vi "Cobra GUI_5.14.vi"(8 "error in":errorcluster) -> (0 "Error Out":errorcluster)   [LabVIEW 2019, in "GUI.lvlib"]
doc: "GUI 21.6.7"
uses:
  GUI.lvlib
  Private Controls/Main Waveform.ctl
  Private Controls/Profile Sequence.ctl
  Private Controls/System Graphs.ctl
  Private Controls/Module Graphs.ctl
  Private Controls/Dial Gauges.ctl
  Private Controls/Gauge Graphs/Compression Ratio.ctl
  Private Controls/Gauge Graphs/Subcooling.ctl
  Private Controls/Gauge Graphs/Superheat.ctl
  Private Controls/Gauge Graphs/Current.ctl
  Private Controls/Module Key Values.ctl
  Private Controls/Event.ctl
  Custom Controls/login.ctl
  Private Controls/Messaging Actions.ctl
  Private Controls/GUI Variables.ctl
  Private Controls/Network Data Down_set back.ctl
  Private Controls/NS New Data.ctl
  <vilib>/NI/STM/TCP/TCP Connection Info.ctl
  <vilib>/NI/STM/SubVIs/MetaDataElement.ctl
  Private Controls/Dataset.ctl
  Private Controls/System Status.ctl
  Private Controls/Module Status.ctl
  Private Controls/M2 Status.ctl
  Private Controls/Config Data.ctl
  <vilib>/Utility/miscctls.llb/LVPositionTypeDef.ctl
  Private Controls/WebDAV states.ctl
  <vilib>/NI/STM/TCP/TCP Read Options.ctl
  46123981-91be-4060-8772-f60ae0a7e702.vi
  <vilib>/Analysis/baseanly.llb/Mean (DBL).vi
  b9938fbe-5ccd-4e62-98e3-88d978d07e59.vi
  795e1a79-78c9-4e5b-9a6d-4827452a9509.vi
  894b418a-eb83-4c03-97c2-0273c02a970a.vi
  81edff22-585a-4beb-bf15-c06a681b6c24.vi
  <vilib>/NI/STM/TCP/Read Meta Data (TCP Ref).vi
  <vilib>/NI/STM/TCP/Get Connection Reference (TCP).vi
  <vilib>/NI/STM/TCP/Read Meta Data (TCP Clst).vi
  <vilib>/NI/STM/TCP/Read Message (TCP).vi
  <vilib>/NI/STM/TCP/Write Message (TCP).vi
  <vilib>/regexp/Match Regular Expression.xnode
  <vilib>/nisyscfg/nisyscfg.lvlib
  <resource>/objmgr/ni.dex.rc
  Private Controls/Save Log State.ctl
  <vilib>/Analysis/NI_AALBase.lvlib
  <vilib>/WebDAVClient/NI_WebDAV.lvlib
  <vilib>/NI/STM/NI STM.lvlib
  <vilib>/addons/_JKI.lib/Serialization/JSON/JKI JSON Serialization.lvlib
panel:
  out "RT Version":string=" May 1st 2021 Cobra GUI v1.0\n\nModule Core.  This is the main VI for a new module. This module is self contained in that it can run on it's own without any other top level VIs. Alternatively you can call this VI from a top level VI and use it as an actor. By default the front panel will open.\n" caption="Cobra GUI Version :"
  in  "Reboot RT":bool
  in  "Shutdown":bool caption="Stop RT"
  in  "M1 Feedback":u8(ring)=1 caption="Enable" items=["Evap Temp", "Case Temp", "Intec Temp", "TSD  Temp", "Autotune", "Extra"]
  in  "M2 Feedback":u8(ring)=1 caption="Enable" items=["Evap Temp", "Case Temp", "Intec Temp", "TSD  Temp", "Autotune", "Extra"]
  out "M2 Data":T1={"Set Temp"=20.0, "Read Temp"=0.0, "Package"="", "Force"=0.0, "Feedback"=1} caption="M2 Status" {"Feedback" items=["Evap Temp", "Case Temp", "Intec Temp", "TSD  Temp", "Autotune", "Extra"]; "Force" format="%4.1f"; "Read Temp" format="%4.1f"; "Set Temp" format="%4.0f"}
  out "M1 Data":T1={"Set Temp"=25.0, "Read Temp"=24.9375, "Package"="new_chip", "Force"=0.0, "Feedback"=1} caption="M1 Status" {"Feedback" items=["Evap Temp", "Case Temp", "Intec Temp", "TSD  Temp", "Autotune", "Extra"]; "Force" format="%4.1f"; "Read Temp" format="%4.1f"; "Set Temp" format="%4.0f"}
  out "Comp":bool caption="System"
  out "Stack light states":T2(ring) caption="System Status"
  in  "Change TSD":bool
  out "TSD Data":T3={"TSD Millivolts"=nan, "X factor"=1.0, "Offset"=0.0, "TSD Temp"=nan, "TSD Feedback"=FALSE, "TSD Max"=225.0, "TSD Min"=-60.0}
  out "M1 AC Load V":dbl
  in  "Net Cluster":T4={"Menu Ring"=0, "System Ready"=TRUE, "Manual IP"="", "Refresh"=FALSE, "IP Override"=FALSE} {"Menu Ring" items=["DemoCobra (192.168.1.76)", "DualCobra109 (192.168.2.9)", "Gen3Cobra127 (192.168.2.27)", "Gen3Cobra129 (192.168.2.29)", "KingCobra118 (192.168.2.18)", "QC-Test (192.168.1.57)", "SeaCobra (192.168.1.49)", "Small-Conduit (192.168.1.201)", "SoftwareTest (192.168.1.109)", "WCGen3Cobra135 (192.168.2.35)"]}
  out "AI (V)":dbl[](array[numeric])=[166.05056229495688, 163.3879875486135, 1.0149508946841042, 0.23376584646698365, 4300076.0, 10.427943481045022, 0.0, 0.0, 0.0, 0.0, 5.0, 5.0, 1625.0, 0.0, 0.0, 0.0, 0.0, 0.0, 0.0, 0.0, 0.0, 0.0, 0.0, 0.0, 0.0, 0.0, 0.0, 0.0, 0.0]
  out "data out":T5={"Condensing Pressure"=165.57116807812622, "Suction Pressure"=163.4397897916897, "Bypass steps"=0, "Operating Time"=0.0, "SubCooling"=-0.3521433751365066, "Superheat"=1.4584003876754537, "M1 Superheat"=0.3615205447980685, "M2 Superheat"=-44.244729455201934, "Autotune output"=0.0, "M1 Testing Elapsed Time"=0.0, "M2 Testing Elapsed Time"=0.0, "M1 Valve Control Mode"=0, "System Amps"=0.23203638796819376, "Compressor Run Time"=0.0, "SD card free Space"=31890.0, "Free Memory"=0.0, "M1 Pressure Feedback"=0.0, "M2 Pressure Feedback"=0.0, "Compression Ratio"=1.0119646390563775, "Serial Number"=0.0, "M1 AC Load V"=0.0, "M1 AC Load W"=10.333236906418378, "M1 DC Load W"=0.0, "M1 RH"=35.98163525597156, "RH Threshold"=120.0}
  in  "Tab Control":T6(tab)=enum."Debug"
  out "M2 Safe Temp and Head State":bool
  out "M2 Bin String":string
  out "M2 PV":dbl caption="M2 Read Temp" format="%4.1f"
  in  "M2 Package":u16(ring)=6 items=["new_chip", "AI_chip", "CPU", "GPU", "300", "250", "", "", "", ""]
  in  "M2 Set Temp":dbl=20.0 min=-50.0 max=150.0 step=5.0 format="%#.1f"
  in  "M2 Commands Panel":T7
  out "M1 Bin String":string
  in  "M1 Set Temp":dbl=25.0 min=-50.0 max=150.0 step=5.0 format="%#.1f"
  in  "M1 Package":u16(ring) items=["new_chip", "AI_chip", "CPU", "GPU", "300", "250", "", "", "", ""]
  out "M1 PV":dbl=24.9375 caption="M1 Read Temp" format="%4.1f"
  in  "M1 Commands Panel":T8={"M1 Enable"=TRUE, "M1 TSD Feedback"=FALSE}
  out "M1 Safe Temp and Head State":bool
  in  "M2 Power Drive Control":bool
  out "M1 Main Waveform":T9=[{"t0"=timestamp(3702896154.5972223 s since 1904-01-01), "dt"=1.0, "Y"=[25.0]}, {"t0"=timestamp(3702896154.5972223 s since 1904-01-01), "dt"=1.0, "Y"=[24.8046875]}, {"t0"=timestamp(3702896154.5972223 s since 1904-01-01), "dt"=1.0, "Y"=[24.9375]}, {"t0"=timestamp(3702896154.5972223 s since 1904-01-01), "dt"=1.0, "Y"=[nan]}]
  in  "M1 Power Drive Control":bool
  out "M2 Power Drive Indicator":bool caption="M2 Power Drive Control"
  out "M1 Power Drive Indicator":bool caption="M1 Power Drive Control"
  in  "Power On-Off":bool
  out "Play/Pause":bool
  out "M2 Main Waveform":T9=[{"t0"=timestamp(3702896154.5972223 s since 1904-01-01), "dt"=1.0, "Y"=[20.0]}, {"t0"=timestamp(3702896154.5972223 s since 1904-01-01), "dt"=1.0, "Y"=[0.0]}, {"t0"=timestamp(3702896154.5972223 s since 1904-01-01), "dt"=1.0, "Y"=[0.0]}, {"t0"=timestamp(3702896154.5972223 s since 1904-01-01), "dt"=1.0, "Y"=[0.0]}]
  out "M1 Channels":dbl[](array[numeric])=[25.0, 24.8046875, 24.9375, nan, 10.492394664499656] format="%4.1f"
  out "M2 Channels":dbl[](array[numeric])=[20.0, 0.0, 0.0, 0.0, 0.0] format="%4.1f"
  out "M1 Humidity":cluster{"M1 RH":dbl, "RH Threshold":dbl}(graph)={"M1 RH"=120.0, "RH Threshold"=35.98163525597156}
  out "Low Side RPM":dbl
  out "High Side RPM":dbl
  out "M2 Thermal State":T10(ring)
  out "System Graphs":T11={"Ambient Temp"=77.534379824996, "Suction Temp"=77.78750485181808, "Condensor Temp"=77.29531729966402, "Discharge Temp"=78.09687988460064, "Bypass Steps"=72.0}
  out "M1 Thermal State":T12(ring)=enum."Steady State"
  out "Gauges":T13={"Condensing Pressure(psi)"=165.57116807812622, "Compression Ratio"=1.0119646390563775, "Subcool"=-0.3368072880168427, "Superheat"=1.4200558413526494, "Current(A)"=0.2333286882987343, "Suction Pressure(psi)"=163.4397897916897} {"Suction Pressure(psi)" scale=0.0..100.0; "Current(A)" scale=5.0..15.0 scale format="%_1f"; "Superheat" scale=0.0..100.0; "Subcool" scale=-10.0..20.0 scale format="%#4.1f"; "Compression Ratio" scale=0.0..30.0 scale format="%#.0f"; "Condensing Pressure(psi)" scale=150.0..375.0}
  in  "Graph Tab CTL":enum32{"Head #1", "Head #2"}(tab)
  out "M1 Graphs":T18={"Case Temp"=24.9375, "Evap Temp"=24.8046875, "Heater Power (%)"=0.0, "EEV Steps"=0.0, "M1 AC Load(W)"=10.492394664499656} caption="Head #1"
  out "M2 Graphs":T18 caption="Head #2"
  in  "Login":T19
  in  "Package":bool
  in  "Configure":bool
  out "Errors":string[](array[string])
  in  "Event Tab":enum32{"Cobra Events", "GUI Events"}(tab)
  out "Event log":T20(array[cluster])=[{"Name"="M1 Set Point", "Time Stamp"=timestamp(3700388973.706829 s since 1904-01-01), "Code"="", "Source"="GUI Event", "Value"=25.0, "Boolean"=FALSE, "String"="", "Error"=FALSE, "Warning"=FALSE, " Fault"=FALSE}, {"Name"="M1 Setpoint Change", "Time Stamp"=timestamp(3700315331.502225 s since 1904-01-01), "Code"="", "Source"="APP:Send Set Temp", "Value"=0.0, "Boolean"=FALSE, "String"="", "Error"=FALSE, "Warning"=TRUE, " Fault"=FALSE}, {"Name"="Bypass Target Change", "Time Stamp"=timestamp(3700299509.350346 s since 1904-01-01), "Code"="", "Source"="Bypass:Get Target", "Value"=110.0, "Boolean"=FALSE, "String"="", "Error"=FALSE, "Warning"=FALSE, " Fault"=FALSE}, {"Name"="PID Bypassed", "Time Stamp"=timestamp(3700299508.870928 s since 1904-01-01), "Code"="", "Source"="APP:Set/Send PID Bypass", "Value"=0.0, "Boolean"=FALSE, "String"="", "Error"=FALSE, "Warning"=FALSE, " Fault"=FALSE}, {"Name"="Read Saved State", "Time Stamp"=timestamp(3700299508.498104 s since 1904-01-01), "Code"="", "Source"="", "Value"=0.0, "Boolean"=FALSE, "String"="", "Error"=FALSE, "Warning"=FALSE, " Fault"=FALSE}, {"Name"="EEV PID Output", "Time Stamp"=timestamp(3700299508.343369 s since 1904-01-01), "Code"="", "Source"="APP:Send EEV PID Out", "Value"=0.0, "Boolean"=FALSE, "String"="Value Change", "Error"=FALSE, "Warning"=FALSE, " Fault"=FALSE}, {"Name"="System Power", "Time Stamp"=timestamp(3700299507.820702 s since 1904-01-01), "Code"="", "Source"="GUI Event", "Value"=nan, "Boolean"=FALSE, "String"="", "Error"=FALSE, "Warning"=FALSE, " Fault"=FALSE}, {"Name"="Bypass PID Gains Change", "Time Stamp"=timestamp(3700299503.315827 s since 1904-01-01), "Code"="", "Source"="Bypass:Get Gains", "Value"=0.0, "Boolean"=FALSE, "String"="", "Error"=FALSE, "Warning"=FALSE, " Fault"=FALSE}, {"Name"="Bypass Target Change", "Time Stamp"=timestamp(3700299503.264928 s since 1904-01-01), "Code"="", "Source"="Bypass:Get Target", "Value"=5.0, "Boolean"=FALSE, "String"="", "Error"=FALSE, "Warning"=FALSE, " Fault"=FALSE}, {"Name"="Send EEV PID Target", "Time Stamp"=timestamp(3700299502.731363 s since 1904-01-01), "Code"="", "Source"="APP:Send EEV PID Target", "Value"=50.0, "Boolean"=FALSE, "String"="", "Error"=FALSE, "Warning"=FALSE, " Fault"=FALSE}, {"Name"="PID Bypassed", "Time Stamp"=timestamp(3700299502.601656 s since 1904-01-01), "Code"="", "Source"="APP:Set/Send PID Bypass", "Value"=0.0, "Boolean"=FALSE, "String"="", "Error"=FALSE, "Warning"=FALSE, " Fault"=FALSE}, {"Name"="Create New Datalog File", "Time Stamp"=timestamp(3700299502.01322 s since 1904-01-01), "Code"="", "Source"="", "Value"=0.0, "Boolean"=FALSE, "String"="", "Error"=FALSE, "Warning"=FALSE, " Fault"=FALSE}, {"Name"="Read Saved State", "Time Stamp"=timestamp(3700299501.897162 s since 1904-01-01), "Code"="", "Source"="", "Value"=0.0, "Boolean"=FALSE, "String"="", "Error"=FALSE, "Warning"=FALSE, " Fault"=FALSE}, {"Name"="System Power", "Time Stamp"=timestamp(3700299500.193215 s since 1904-01-01), "Code"="", "Source"="GUI Event", "Value"=nan, "Boolean"=TRUE, "String"="", "Error"=FALSE, "Warning"=FALSE, " Fault"=FALSE}, {"Name"="Thermal Status Change", "Time Stamp"=timestamp(3700299426.299148 s since 1904-01-01), "Code"="", "Source"="APP:Thermal Status", "Value"=0.0, "Boolean"=FALSE, "String"="", "Error"=FALSE, "Warning"=FALSE, " Fault"=FALSE}, {"Name"="M1 Setpoint Change", "Time Stamp"=timestamp(3700299426.185991 s since 1904-01-01), "Code"="", "Source"="APP:Send Set Temp", "Value"=25.0, "Boolean"=FALSE, "String"="", "Error"=FALSE, "Warning"=TRUE, " Fault"=FALSE}, {"Name"="Bypass Target Change", "Time Stamp"=timestamp(3700146637.449938 s since 1904-01-01), "Code"="", "Source"="Bypass:Get Target", "Value"=110.0, "Boolean"=FALSE, "String"="", "Error"=FALSE, "Warning"=FALSE, " Fault"=FALSE}, {"Name"="PID Bypassed", "Time Stamp"=timestamp(3700146637.072199 s since 1904-01-01), "Code"="", "Source"="APP:Set/Send PID Bypass", "Value"=0.0, "Boolean"=FALSE, "String"="", "Error"=FALSE, "Warning"=FALSE, " Fault"=FALSE}, {"Name"="Read Saved State", "Time Stamp"=timestamp(3700146636.7019 s since 1904-01-01), "Code"="", "Source"="", "Value"=0.0, "Boolean"=FALSE, "String"="", "Error"=FALSE, "Warning"=FALSE, " Fault"=FALSE}, {"Name"="EEV PID Output", "Time Stamp"=timestamp(3700146636.547449 s since 1904-01-01), "Code"="", "Source"="APP:Send EEV PID Out", "Value"=0.0, "Boolean"=FALSE, "String"="Value Change", "Error"=FALSE, "Warning"=FALSE, " Fault"=FALSE}, {"Name"="System Power", "Time Stamp"=timestamp(3700146635.436145 s since 1904-01-01), "Code"="", "Source"="GUI Event", "Value"=nan, "Boolean"=FALSE, "String"="", "Error"=FALSE, "Warning"=FALSE, " Fault"=FALSE}, {"Name"="Bypass Reset", "Time Stamp"=timestamp(3700145043.86988 s since 1904-01-01), "Code"="", "Source"="Bypass:Reset Bypass", "Value"=0.0, "Boolean"=FALSE, "String"="", "Error"=FALSE, "Warning"=FALSE, " Fault"=FALSE}, {"Name"="Bypass Reset", "Time Stamp"=timestamp(3700145042.728279 s since 1904-01-01), "Code"="", "Source"="Bypass:Reset Bypass", "Value"=0.0, "Boolean"=TRUE, "String"="", "Error"=FALSE, "Warning"=FALSE, " Fault"=FALSE}, {"Name"="Bypass PID Gains Change", "Time Stamp"=timestamp(3700145042.677721 s since 1904-01-01), "Code"="", "Source"="Bypass:Get Gains", "Value"=0.0, "Boolean"=FALSE, "String"="", "Error"=FALSE, "Warning"=FALSE, " Fault"=FALSE}, {"Name"="Send EEV PID Target", "Time Stamp"=timestamp(3700145041.342134 s since 1904-01-01), "Code"="", "Source"="APP:Send EEV PID Target", "Value"=10.0, "Boolean"=FALSE, "String"="", "Error"=FALSE, "Warning"=FALSE, " Fault"=FALSE}, {"Name"="EEV PID Output", "Time Stamp"=timestamp(3700145041.326132 s since 1904-01-01), "Code"="", "Source"="APP:Send EEV PID Out", "Value"=0.0, "Boolean"=FALSE, "String"="Value Change", "Error"=FALSE, "Warning"=FALSE, " Fault"=FALSE}, {"Name"="M1 Setpoint Change", "Time Stamp"=timestamp(3700145041.207587 s since 1904-01-01), "Code"="", "Source"="APP:Send Set Temp", "Value"=-40.0, "Boolean"=FALSE, "String"="", "Error"=FALSE, "Warning"=TRUE, " Fault"=FALSE}, {"Name"="Bypass Reset", "Time Stamp"=timestamp(3700145028.649825 s since 1904-01-01), "Code"="", "Source"="Bypass:Reset Bypass", "Value"=0.0, "Boolean"=FALSE, "String"="", "Error"=FALSE, "Warning"=FALSE, " Fault"=FALSE}, {"Name"="Bypass Reset", "Time Stamp"=timestamp(3700145027.500021 s since 1904-01-01), "Code"="", "Source"="Bypass:Reset Bypass", "Value"=0.0, "Boolean"=TRUE, "String"="", "Error"=FALSE, "Warning"=FALSE, " Fault"=FALSE}, {"Name"="Bypass PID Gains Change", "Time Stamp"=timestamp(3700145027.445379 s since 1904-01-01), "Code"="", "Source"="Bypass:Get Gains", "Value"=0.0, "Boolean"=FALSE, "String"="", "Error"=FALSE, "Warning"=FALSE, " Fault"=FALSE}, {"Name"="Bypass Target Change", "Time Stamp"=timestamp(3700145027.393371 s since 1904-01-01), "Code"="", "Source"="Bypass:Get Target", "Value"=5.0, "Boolean"=FALSE, "String"="", "Error"=FALSE, "Warning"=FALSE, " Fault"=FALSE}, {"Name"="Send EEV PID Target", "Time Stamp"=timestamp(3700145026.918826 s since 1904-01-01), "Code"="", "Source"="APP:Send EEV PID Target", "Value"=50.0, "Boolean"=FALSE, "String"="", "Error"=FALSE, "Warning"=FALSE, " Fault"=FALSE}, {"Name"="PID Bypassed", "Time Stamp"=timestamp(3700145026.784981 s since 1904-01-01), "Code"="", "Source"="APP:Set/Send PID Bypass", "Value"=0.0, "Boolean"=FALSE, "String"="", "Error"=FALSE, "Warning"=FALSE, " Fault"=FALSE}, {"Name"="Create New Datalog File", "Time Stamp"=timestamp(3700145026.176328 s since 1904-01-01), "Code"="", "Source"="", "Value"=0.0, "Boolean"=FALSE, "String"="", "Error"=FALSE, "Warning"=FALSE, " Fault"=FALSE}, {"Name"="Read Saved State", "Time Stamp"=timestamp(3700145025.971426 s since 1904-01-01), "Code"="", "Source"="", "Value"=0.0, "Boolean"=FALSE, "String"="", "Error"=FALSE, "Warning"=FALSE, " Fault"=FALSE}, {"Name"="System Power", "Time Stamp"=timestamp(3700145024.855234 s since 1904-01-01), "Code"="", "Source"="GUI Event", "Value"=nan, "Boolean"=TRUE, "String"="", "Error"=FALSE, "Warning"=FALSE, " Fault"=FALSE}, {"Name"="Bypass Target Change", "Time Stamp"=timestamp(3700144860.396659 s since 1904-01-01), "Code"="", "Source"="Bypass:Get Target", "Value"=110.0, "Boolean"=FALSE, "String"="", "Error"=FALSE, "Warning"=FALSE, " Fault"=FALSE}, {"Name"="Mains Frequency", "Time Stamp"=timestamp(3700144859.665863 s since 1904-01-01), "Code"="", "Source"="Init System Module", "Value"=60.021391215683806, "Boolean"=FALSE, "String"="", "Error"=FALSE, "Warning"=FALSE, " Fault"=FALSE}, {"Name"="PID Bypassed", "Time Stamp"=timestamp(3700144856.200222 s since 1904-01-01), "Code"="", "Source"="APP:Set/Send PID Bypass", "Value"=0.0, "Boolean"=FALSE, "String"="", "Error"=FALSE, "Warning"=FALSE, " Fault"=FALSE}, {"Name"="M1 Setpoint Change", "Time Stamp"=timestamp(3700144856.062369 s since 1904-01-01), "Code"="", "Source"="APP:Send Set Temp", "Value"=25.0, "Boolean"=FALSE, "String"="", "Error"=FALSE, "Warning"=TRUE, " Fault"=FALSE}, {"Name"="Bypass Inintialize", "Time Stamp"=timestamp(3700144855.986915 s since 1904-01-01), "Code"="", "Source"="", "Value"=4594.0, "Boolean"=FALSE, "String"="Complete", "Error"=FALSE, "Warning"=FALSE, " Fault"=FALSE}, {"Name"="M1 EEV Check Position", "Time Stamp"=timestamp(3700144845.750249 s since 1904-01-01), "Code"="", "Source"="EEV:Check Position", "Value"=0.0, "Boolean"=FALSE, "String"="", "Error"=FALSE, "Warning"=FALSE, " Fault"=FALSE}, {"Name"="", "Time Stamp"=timestamp(3700144845.71115 s since 1904-01-01), "Code"="", "Source"="EEV:Config", "Value"=0.0, "Boolean"=FALSE, "String"="", "Error"=FALSE, "Warning"=FALSE, " Fault"=FALSE}, {"Name"="Config Loaded", "Time Stamp"=timestamp(3700144844.323102 s since 1904-01-01), "Code"="", "Source"="Config Read Initialize", "Value"=0.0, "Boolean"=FALSE, "String"="", "Error"=FALSE, "Warning"=FALSE, " Fault"=FALSE}, {"Name"="Config Read", "Time Stamp"=timestamp(3700144844.317077 s since 1904-01-01), "Code"="Found", "Source"="M2 TSD", "Value"=0.0, "Boolean"=FALSE, "String"="V Offset", "Error"=FALSE, "Warning"=FALSE, " Fault"=FALSE}, {"Name"="Config Read", "Time Stamp"=timestamp(3700144844.305088 s since 1904-01-01), "Code"="Found", "Source"="M2 TSD", "Value"=1.0, "Boolean"=FALSE, "String"="Gain", "Error"=FALSE, "Warning"=FALSE, " Fault"=FALSE}, {"Name"="Config Read", "Time Stamp"=timestamp(3700144844.293052 s since 1904-01-01), "Code"="Found", "Source"="M1 TSD", "Value"=0.0, "Boolean"=FALSE, "String"="Offset", "Error"=FALSE, "Warning"=FALSE, " Fault"=FALSE}, {"Name"="Config Read", "Time Stamp"=timestamp(3700144844.273617 s since 1904-01-01), "Code"="Found", "Source"="M1 T-Case Calibration", "Value"=0.0, "Boolean"=FALSE, "String"="Offset", "Error"=FALSE, "Warning"=FALSE, " Fault"=FALSE}, {"Name"="Config Read", "Time Stamp"=timestamp(3700144844.259388 s since 1904-01-01), "Code"="Found", "Source"="Heater PID TSD", "Value"=0.264, "Boolean"=FALSE, "String"="Integral Value", "Error"=FALSE, "Warning"=FALSE, " Fault"=FALSE}, {"Name"="Config Read", "Time Stamp"=timestamp(3700144844.236238 s since 1904-01-01), "Code"="Found", "Source"="M2 EEV PID", "Value"=-1.0, "Boolean"=FALSE, "String"="Gain P", "Error"=FALSE, "Warning"=FALSE, " Fault"=FALSE}, {"Name"="Config Read", "Time Stamp"=timestamp(3700144844.209533 s since 1904-01-01), "Code"="Found", "Source"="EEV PID", "Value"=0.0, "Boolean"=FALSE, "String"="Gain D", "Error"=FALSE, "Warning"=FALSE, " Fault"=FALSE}, {"Name"="Config Read", "Time Stamp"=timestamp(3700144844.188812 s since 1904-01-01), "Code"="Found", "Source"="EEV PID", "Value"=30.0, "Boolean"=FALSE, "String"="SS Steps", "Error"=FALSE, "Warning"=FALSE, " Fault"=FALSE}, {"Name"="Config Read", "Time Stamp"=timestamp(3700144844.156754 s since 1904-01-01), "Code"="Found", "Source"="EEV PID", "Value"=70.0, "Boolean"=FALSE, "String"="EBB Steps Open", "Error"=FALSE, "Warning"=FALSE, " Fault"=FALSE}, {"Name"="Config Read", "Time Stamp"=timestamp(3700144844.131652 s since 1904-01-01), "Code"="Found", "Source"="EEV PID", "Value"=50.0, "Boolean"=FALSE, "String"="RU Target", "Error"=FALSE, "Warning"=FALSE, " Fault"=FALSE}, {"Name"="Config Read", "Time Stamp"=timestamp(3700144844.102271 s since 1904-01-01), "Code"="Found", "Source"="Set Point Range", "Value"=-50.0, "Boolean"=FALSE, "String"="Min", "Error"=FALSE, "Warning"=FALSE, " Fault"=FALSE}, {"Name"="Config Read", "Time Stamp"=timestamp(3700144844.07361 s since 1904-01-01), "Code"="Found", "Source"="M2 Heater PID", "Value"=0.0, "Boolean"=FALSE, "String"="Derivative Value", "Error"=FALSE, "Warning"=FALSE, " Fault"=FALSE}, {"Name"="M1 EEV Check Position", "Time Stamp"=timestamp(3700144844.059525 s since 1904-01-01), "Code"="", "Source"="", "Value"=0.0, "Boolean"=TRUE, "String"="Complete", "Error"=FALSE, "Warning"=FALSE, " Fault"=FALSE}, {"Name"="Config Read", "Time Stamp"=timestamp(3700144844.04058 s since 1904-01-01), "Code"="Found", "Source"="Heater PID", "Value"=8.207, "Boolean"=FALSE, "String"="Proportional Value", "Error"=FALSE, "Warning"=FALSE, " Fault"=FALSE}, {"Name"="Config Read", "Time Stamp"=timestamp(3700144844.027634 s since 1904-01-01), "Code"="Found", "Source"="Piston Settings", "Value"=5000.0, "Boolean"=FALSE, "String"="Delay (ms)", "Error"=FALSE, "Warning"=FALSE, " Fault"=FALSE}, {"Name"="Config Read", "Time Stamp"=timestamp(3700144844.012692 s since 1904-01-01), "Code"="Found", "Source"="Piston Settings", "Value"=0.4, "Boolean"=FALSE, "String"="Transition Force", "Error"=FALSE, "Warning"=FALSE, " Fault"=FALSE}, {"Name"="Config Read", "Time Stamp"=timestamp(3700144843.999205 s since 1904-01-01), "Code"="Found", "Source"="Bypass PID", "Value"=0.0, "Boolean"=FALSE, "String"="Derivative Value", "Error"=FALSE, "Warning"=FALSE, " Fault"=FALSE}, {"Name"="Config Value Read", "Time Stamp"=timestamp(3700144843.985241 s since 1904-01-01), "Code"="", "Source"="", "Value"=0.0, "Boolean"=TRUE, "String"="Cascade", "Error"=FALSE, "Warning"=FALSE, " Fault"=FALSE}, {"Name"="Config Value Read", "Time Stamp"=timestamp(3700144843.957428 s since 1904-01-01), "Code"="", "Source"="", "Value"=0.0, "Boolean"=TRUE, "String"="Benchtop", "Error"=FALSE, "Warning"=FALSE, " Fault"=FALSE}, {"Name"="Config Value Read", "Time Stamp"=timestamp(3700144843.937723 s since 1904-01-01), "Code"="", "Source"="", "Value"=0.0, "Boolean"=TRUE, "String"="HandClamp", "Error"=FALSE, "Warning"=FALSE, " Fault"=FALSE}, {"Name"="Config Value Read", "Time Stamp"=timestamp(3700144843.913773 s since 1904-01-01), "Code"="", "Source"="", "Value"=0.0, "Boolean"=TRUE, "String"="FTC200", "Error"=FALSE, "Warning"=FALSE, " Fault"=FALSE}, {"Name"="Read Saved State", "Time Stamp"=timestamp(3700144843.835266 s since 1904-01-01), "Code"="", "Source"="", "Value"=0.0, "Boolean"=FALSE, "String"="", "Error"=FALSE, "Warning"=FALSE, " Fault"=FALSE}, {"Name"="EMO Not Detected", "Time Stamp"=timestamp(3700144843.758465 s since 1904-01-01), "Code"="", "Source"="", "Value"=0.0, "Boolean"=FALSE, "String"="", "Error"=FALSE, "Warning"=FALSE, " Fault"=FALSE}, {"Name"="EEV PID Output", "Time Stamp"=timestamp(3700144843.701921 s since 1904-01-01), "Code"="", "Source"="APP:Send EEV PID Out", "Value"=2000.0, "Boolean"=FALSE, "String"="Value Change", "Error"=FALSE, "Warning"=FALSE, " Fault"=FALSE}, {"Name"="Read Compressor Minutes", "Time Stamp"=timestamp(3700144843.672015 s since 1904-01-01), "Code"="", "Source"="", "Value"=3551.0, "Boolean"=TRUE, "String"="PASS", "Error"=FALSE, "Warning"=FALSE, " Fault"=FALSE}, {"Name"="FPGA Load Complete", "Time Stamp"=timestamp(3700144843.612085 s since 1904-01-01), "Code"="", "Source"="Init FPGA IO.vi", "Value"=0.0, "Boolean"=FALSE, "String"="", "Error"=FALSE, "Warning"=FALSE, " Fault"=FALSE}, {"Name"="Pressure Test", "Time Stamp"=timestamp(3700144841.60851 s since 1904-01-01), "Code"="", "Source"="Init FPGA IO 2.0.vi", "Value"=1.0061036087586785, "Boolean"=FALSE, "String"="FAIL", "Error"=FALSE, "Warning"=TRUE, " Fault"=FALSE}, {"Name"="Stop LCD", "Time Stamp"=timestamp(3700144836.391427 s since 1904-01-01), "Code"="", "Source"="Init FPGA IO.vi", "Value"=11.0, "Boolean"=FALSE, "String"="", "Error"=FALSE, "Warning"=FALSE, " Fault"=FALSE}, {"Name"="wait", "Time Stamp"=timestamp(3700144835.388984 s since 1904-01-01), "Code"="", "Source"="Init FPGA IO.vi", "Value"=10.0, "Boolean"=FALSE, "String"="", "Error"=FALSE, "Warning"=FALSE, " Fault"=FALSE}, {"Name"="IP Address", "Time Stamp"=timestamp(3700144834.385193 s since 1904-01-01), "Code"="", "Source"="Init FPGA IO.vi", "Value"=12.0, "Boolean"=FALSE, "String"="þQ", "Error"=FALSE, "Warning"=FALSE, " Fault"=FALSE}, {"Name"="wait", "Time Stamp"=timestamp(3700144832.839035 s since 1904-01-01), "Code"="", "Source"="Init FPGA IO.vi", "Value"=10.0, "Boolean"=FALSE, "String"="", "Error"=FALSE, "Warning"=FALSE, " Fault"=FALSE}, {"Name"="Rev Display", "Time Stamp"=timestamp(3700144831.835933 s since 1904-01-01), "Code"="", "Source"="Init FPGA IO.vi", "Value"=9.0, "Boolean"=FALSE, "String"="Ver: CC 21.4.8.1", "Error"=FALSE, "Warning"=FALSE, " Fault"=FALSE}, {"Name"="wait", "Time Stamp"=timestamp(3700144831.786862 s since 1904-01-01), "Code"="", "Source"="Init FPGA IO.vi", "Value"=10.0, "Boolean"=FALSE, "String"="", "Error"=FALSE, "Warning"=FALSE, " Fault"=FALSE}, {"Name"="Chroma Display", "Time Stamp"=timestamp(3700144830.785101 s since 1904-01-01), "Code"="", "Source"="Init FPGA IO.vi", "Value"=8.0, "Boolean"=FALSE, "String"="Chroma ATE", "Error"=FALSE, "Warning"=FALSE, " Fault"=FALSE}, {"Name"="wait", "Time Stamp"=timestamp(3700144830.711098 s since 1904-01-01), "Code"="", "Source"="Init FPGA IO.vi", "Value"=10.0, "Boolean"=FALSE, "String"="", "Error"=FALSE, "Warning"=FALSE, " Fault"=FALSE}, {"Name"="Clear LCD Text", "Time Stamp"=timestamp(3700144829.705271 s since 1904-01-01), "Code"="", "Source"="Init FPGA IO.vi", "Value"=0.0, "Boolean"=FALSE, "String"="", "Error"=FALSE, "Warning"=FALSE, " Fault"=FALSE}, {"Name"="BootLoad", "Time Stamp"=timestamp(3700144828.60264 s since 1904-01-01), "Code"="", "Source"="Init FPGA IO.vi", "Value"=0.0, "Boolean"=FALSE, "String"="", "Error"=FALSE, "Warning"=FALSE, " Fault"=FALSE}, {"Name"="Extra Settings Loaded", "Time Stamp"=timestamp(3700144827.700333 s since 1904-01-01), "Code"="", "Source"="", "Value"=0.0, "Boolean"=FALSE, "String"="", "Error"=FALSE, "Warning"=FALSE, " Fault"=FALSE}, {"Name"="Warmup ", "Time Stamp"=timestamp(3700144827.667711 s since 1904-01-01), "Code"="", "Source"="Extra Settings", "Value"=0.0, "Boolean"=FALSE, "String"="", "Error"=FALSE, "Warning"=TRUE, " Fault"=FALSE}, {"Name"="Heads Disabled", "Time Stamp"=timestamp(3700144827.642226 s since 1904-01-01), "Code"="", "Source"="Extra Settings", "Value"=0.0, "Boolean"=TRUE, "String"="", "Error"=FALSE, "Warning"=FALSE, " Fault"=FALSE}, {"Name"="Low Amperage", "Time Stamp"=timestamp(3700144827.619487 s since 1904-01-01), "Code"="", "Source"="Extra Settings", "Value"=0.0, "Boolean"=TRUE, "String"="", "Error"=FALSE, "Warning"=FALSE, " Fault"=FALSE}, {"Name"="Warnings/Faults 1", "Time Stamp"=timestamp(3700144827.570458 s since 1904-01-01), "Code"="", "Source"="Extra Settings 3", "Value"=0.0, "Boolean"=TRUE, "String"="", "Error"=FALSE, "Warning"=FALSE, " Fault"=FALSE}, {"Name"="Read System Settings", "Time Stamp"=timestamp(3700144827.547197 s since 1904-01-01), "Code"="", "Source"="Read Extra Settings", "Value"=0.0, "Boolean"=FALSE, "String"="", "Error"=FALSE, "Warning"=TRUE, " Fault"=FALSE}, {"Name"="Config Loaded", "Time Stamp"=timestamp(3700144827.514774 s since 1904-01-01), "Code"="", "Source"="Config Read Initialize", "Value"=0.0, "Boolean"=FALSE, "String"="", "Error"=FALSE, "Warning"=FALSE, " Fault"=FALSE}, {"Name"="Config Read", "Time Stamp"=timestamp(3700144827.494679 s since 1904-01-01), "Code"="Found", "Source"="M1 T-Case Calibration", "Value"=0.0, "Boolean"=FALSE, "String"="Offset", "Error"=FALSE, "Warning"=FALSE, " Fault"=FALSE}, {"Name"="Config Read", "Time Stamp"=timestamp(3700144827.471638 s since 1904-01-01), "Code"="Found", "Source"="EEV PID", "Value"=0.0, "Boolean"=FALSE, "String"="Output Low", "Error"=FALSE, "Warning"=FALSE, " Fault"=FALSE}, {"Name"="Config Read", "Time Stamp"=timestamp(3700144827.449028 s since 1904-01-01), "Code"="Found", "Source"="EEV PID", "Value"=70.0, "Boolean"=FALSE, "String"="EBB Steps Open", "Error"=FALSE, "Warning"=FALSE, " Fault"=FALSE}, {"Name"="Config Read", "Time Stamp"=timestamp(3700144827.428326 s since 1904-01-01), "Code"="Found", "Source"="Set Point Range", "Value"=150.0, "Boolean"=FALSE, "String"="Max", "Error"=FALSE, "Warning"=FALSE, " Fault"=FALSE}, {"Name"="Config Read", "Time Stamp"=timestamp(3700144827.414612 s since 1904-01-01), "Code"="Found", "Source"="M2 Heater PID", "Value"=8.0, "Boolean"=FALSE, "String"="Proportional Value", "Error"=FALSE, "Warning"=FALSE, " Fault"=FALSE}, {"Name"="Config Read", "Time Stamp"=timestamp(3700144827.386952 s since 1904-01-01), "Code"="Found", "Source"="Bypass PID", "Value"=0.0, "Boolean"=FALSE, "String"="Derivative Value", "Error"=FALSE, "Warning"=FALSE, " Fault"=FALSE}, {"Name"="Config Value Read", "Time Stamp"=timestamp(3700144827.362201 s since 1904-01-01), "Code"="", "Source"="", "Value"=0.0, "Boolean"=TRUE, "String"="Sensors", "Error"=FALSE, "Warning"=FALSE, " Fault"=FALSE}] {"Value" format="%4.1f"; "Time Stamp" format="%<%x %.3X>T"}
  out "GUI Events":T21[](array[typedef]) {"Time Stamp" format="%<%x %.3X>T"}
  in  "Datalog":bool
  out "M2 Buffer":dbl(slide)=0.9999999999999998 scale=-4.0..4.0
  out "M2 Valve Output":dbl(knob) scale=0.0..100.0
  in  "Y-scale":bool
  out "Boot Up Time":timestamp=timestamp(3700144843.654765 s since 1904-01-01)
  out "M2 Heater %":dbl format="%3.0f"
  out "M2 Error":bool
  out "M2 Actuated":bool
  out "M2 Head State":enum16{"Disabled", "Run", "Error"}(ring)=enum."Run"
  out "M2 Thermal Status":T12(ring)
  in  "M2 EEV Manual":u16
  in  "M2 Heater Output":dbl
  in  "M1 EEV Manual":u16
  in  "Manual Bypass Mode":bool[](array[boolean])
  in  "M1 Heater output":dbl
  out "M1 Valve Output":dbl(knob) scale=0.0..100.0
  out "M1 Buffer":dbl(slide)=0.9999999999999998 scale=-4.0..4.0
  out "Detected Systems":string[](array[string])=["DemoCobra (192.168.1.76)", "DualCobra108 (192.168.2.8)", "Gen3Cobra123 (192.168.2.23)", "Gen3Cobra124 (192.168.2.24)", "Gen3Cobra125 (192.168.2.25)", "KingCobra115 (192.168.2.15)", "KingCobra117 (192.168.2.17)", "QC-Test (192.168.1.57)", "Small-Conduit (192.168.1.201)"]
  out "Data Rx Timestamp":timestamp=timestamp(3700634217.978288 s since 1904-01-01)
  out "M1 Superheat":dbl=0.3615205447980685 format="%#.1f"
  out "M1 Testing Elapsed Time":dbl caption="Test Elapsed Time" format="%<%H:%M:%S>t"
  out "TCP Connections":T22(array[cluster])=[{"port "=1300, "remote address"="", "Connection timeout ms"=100, "Waiting for connection"=TRUE, "Waiting for Command"=FALSE, "timeout ms"=5000}, {"port "=1100, "remote address"="", "Connection timeout ms"=100, "Waiting for connection"=TRUE, "Waiting for Command"=FALSE, "timeout ms"=-1}, {"port "=1000, "remote address"="", "Connection timeout ms"=100, "Waiting for connection"=TRUE, "Waiting for Command"=FALSE, "timeout ms"=60000}, {"port "=1001, "remote address"="", "Connection timeout ms"=100, "Waiting for connection"=TRUE, "Waiting for Command"=FALSE, "timeout ms"=60000}, {"port "=2100, "remote address"="", "Connection timeout ms"=100, "Waiting for connection"=FALSE, "Waiting for Command"=FALSE, "timeout ms"=-1}, {"port "=2001, "remote address"="", "Connection timeout ms"=100, "Waiting for connection"=FALSE, "Waiting for Command"=FALSE, "timeout ms"=60000}, {"port "=2000, "remote address"="", "Connection timeout ms"=100, "Waiting for connection"=FALSE, "Waiting for Command"=FALSE, "timeout ms"=5000}]
  out "Error":string[](array[string])
  in  "Cascade Compressor controls":T23 {"Manual Low Stage frequency" min=40.0 max=150.0 step=1.0; "Manual High stage frequency" min=50.0 max=150.0 step=1.0}
  out "TCP commands":string[](array[string])=["M1 ENABLE()\r\n", "Tue 23 Mar 2021 01:23:29 PM PDT"]
  out "M1 Head State":enum16{"Disabled", "Run", "Error"}(ring)
  out "M1 Thermal Status":T12(ring)=enum."Steady State"
  out "M1 Error":bool
  out "M1 Actuated":bool
  out "M1 Heater %":dbl format="%3.0f"
  out "Sleep":bool=TRUE
  out "Sleep Timer":dbl=-1.0
  out "Comp Temp":dbl=78.09687988460064 format="%#.1f"
  out "SOM":T24={"Software Version"="SW Version:CC 21.4.8.1", "CPU Usage"=40.953570959266244, "Memory Available"=353.72, "SOM Storage(MB)"=243.036, "SD card free space"=31.886} caption="System of Module" {"SD card free space" format="%#4.1f"; "CPU Usage" format="%#.1f"; "Memory Available" format="%#4.1f"; "SOM Storage(MB)" format="%4.1f"}
  out "Compressor Hours":dbl=59.65 caption="Comp hrs" format="%#.1f"
  out "Serial Number":string="204300076"
  in  "Graph Temp Unit":bool
  in  "Average Graph":bool
  in  "Fixed Y-Range":dbl=4.0
  in  "Login TO":i32=10 caption="Login Timeout(min)" min=-1
  in  "Iteration No":i32=2 caption="Head Load(W)"
  in  "Power Seq":T25=[{"Duration"=0, "Head Load(W)"=0, "Name"="Step1"}, {"Duration"=10, "Head Load(W)"=0, "Name"="Step2"}, {"Duration"=10, "Head Load(W)"=0, "Name"="Step3"}, {"Duration"=20, "Head Load(W)"=0, "Name"="Step4"}, {"Duration"=20, "Head Load(W)"=0, "Name"="Step5"}, {"Duration"=30, "Head Load(W)"=0, "Name"="Step6"}, {"Duration"=30, "Head Load(W)"=0, "Name"="Step7"}, {"Duration"=40, "Head Load(W)"=0, "Name"="Step8"}, {"Duration"=40, "Head Load(W)"=0, "Name"="Step9"}, {"Duration"=50, "Head Load(W)"=0, "Name"="Step10"}]
  in  "Pattern File":string(combo)="S1.ini" caption="Default Pattern Folder"
  in  "Seq Controls":T26
  out "Cycle":i32=1
  in  "Serial Port":string(combo)="COM5" caption="Default Pattern Folder"
  in  "Power":bool caption="Test/Stop"
  out "Time":dbl caption="Time(sec)" format="%<%H:%M:%S>t"
  in  "Reset Test":bool
  in  "Stop Test":bool
  in  "Start Test":bool
  out "Test Graph":dbl[](graph)
  out "Boot Time(s)":u32=8
  in  "Boot Time out(s)":u32=4
  out "Step":string
  out "Infinite Test":string caption="Infinite Cycle"
  out "Response":string
  in  "Command":string="VOLTAGE:AC 0"
  in  "Custom Command":bool caption="Send"
  # "System Module"
  # "M1 Module"
  # "M2 Module"
  # "Tuning"
  # "Manual Controls"
  # "AC Power Supply"
  # "on"
  # "Step"
  # "Duration"
  # "Heat Load(W)"
  # "off"
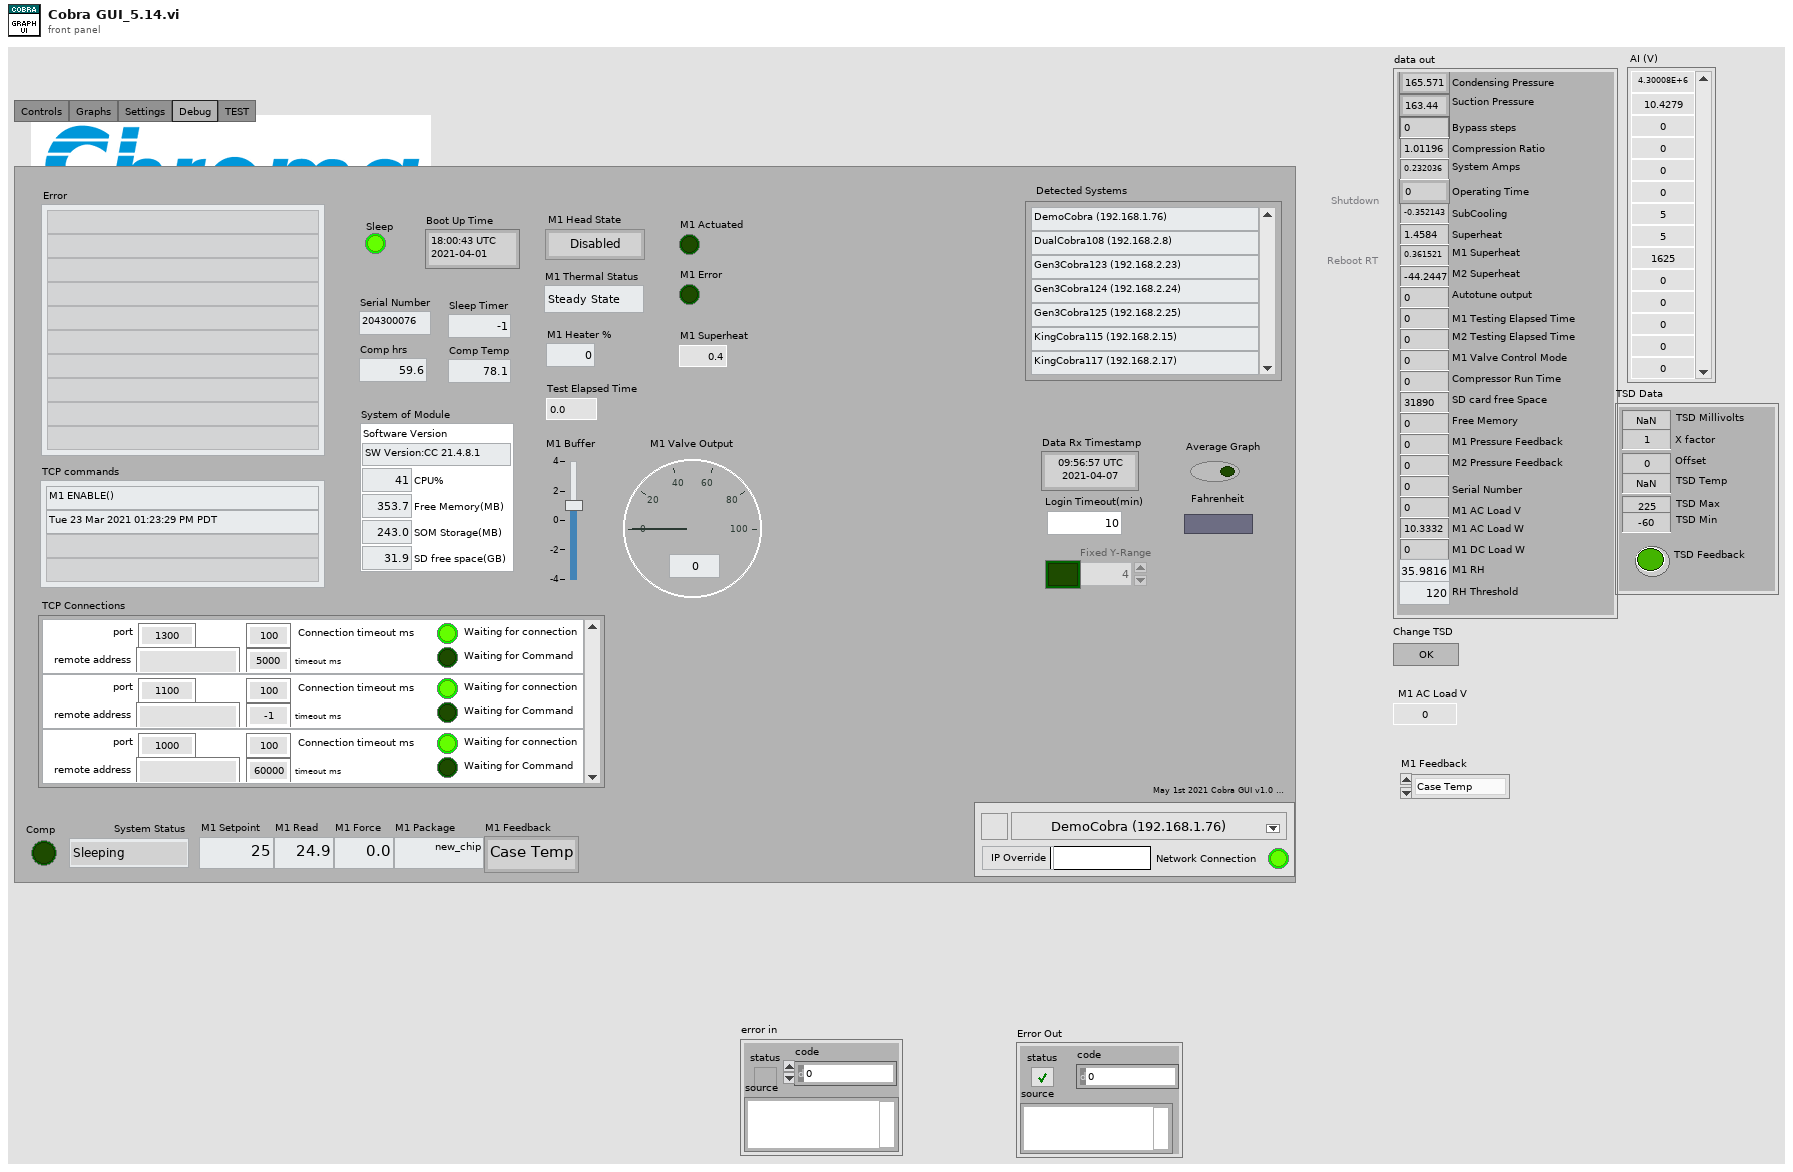
[diagram p1: front panel]
types:
  T1 = typedef "GUI.lvlib/Module Key Values.ctl" = cluster{"Set Temp":dbl, "Read Temp":dbl, "Package":string, "Force":dbl, "Feedback":u8}
  T2 = enum16{"Sleeping", "Warming up", "Ready", "Testing", "Restless", "Idle", "Sleeping Fault", "warning"}
  T3 = cluster{"TSD Millivolts":dbl, "X factor":dbl, "Offset":dbl, "TSD Temp":dbl, "TSD Feedback":bool, "TSD Max":dbl, "TSD Min":dbl}
  T4 = cluster{"Menu Ring":u16, "System Ready":bool, "Manual IP":string, "Refresh":bool, "IP Override":bool}
  T5 = cluster{"Condensing Pressure":dbl, "Suction Pressure":dbl, "Bypass steps":u16, "Operating Time":dbl, "SubCooling":dbl, "Superheat":dbl, "M1 Superheat":dbl, "M2 Superheat":dbl, "Autotune output":dbl, "M1 Testing Elapsed Time":dbl, "M2 Testing Elapsed Time":dbl, "M1 Valve Control Mode":u8, "System Amps":dbl, "Compressor Run Time":dbl, "SD card free Space":dbl, "Free Memory":dbl, "M1 Pressure Feedback":dbl, "M2 Pressure Feedback":dbl, "Compression Ratio":dbl, "Serial Number":dbl, "M1 AC Load V":dbl, "M1 AC Load W":dbl, "M1 DC Load W":dbl, "M1 RH":dbl, "RH Threshold":dbl}
  T6 = enum32{"Controls", "Graphs", "Settings", "Debug", "TEST"}
  T7 = cluster{"M2 Enable":bool, "M2 TSD Feedback":bool}
  T8 = cluster{"M1 Enable":bool, "M1 TSD Feedback":bool}
  T9 = typedef "GUI.lvlib/Main Waveform.ctl" = waveform(dbl)[]
  T10 = enum16{"Ramp Up", "Ramp Down", "Steady State", "Ebb and Flow", "Up", "Under Load", "Cryo Mode", "Shuttle Mode"}
  T11 = typedef "GUI.lvlib/System Graphs.ctl" = cluster{"Ambient Temp":dbl, "Suction Temp":dbl, "Condensor Temp":dbl, "Discharge Temp":dbl, "Bypass Steps":dbl}
  T12 = enum16{"Ramp Up", "Ramp Down", "Steady State", "Ebb and Flow", "Up", "Under Load", "Cryo Mode"}
  T13 = typedef "GUI.lvlib/Dial Gauges.ctl" = cluster{"Condensing Pressure(psi)":dbl, "Compression Ratio":T14, "Subcool":T15, "Superheat":T16, "Current(A)":T17, "Suction Pressure(psi)":dbl}
  T14 = typedef "GUI.lvlib/Compression Ratio.ctl" = dbl
  T15 = typedef "GUI.lvlib/Subcooling.ctl" = dbl
  T16 = typedef "GUI.lvlib/Superheat.ctl" = dbl
  T17 = typedef "GUI.lvlib/Current.ctl" = dbl
  T18 = typedef "GUI.lvlib/Module Graphs.ctl" = cluster{"Case Temp":dbl, "Evap Temp":dbl, "Heater Power (%)":dbl, "EEV Steps":dbl, "M1 AC Load(W)":dbl}
  T19 = typedef "GUI.lvlib/login.ctl" = bool
  T20 = cluster{"Name":string, "Time Stamp":timestamp, "Code":string, "Source":string, "Value":dbl, "Boolean":bool, "String":string, "Error":bool, "Warning":bool, " Fault":bool}[]
  T21 = typedef "GUI.lvlib/Event.ctl" = cluster{"Name":string, "Time Stamp":timestamp, "Code":i32, "Source":string, "Value":string, "Boolean":bool, "Description":string, "Error":bool, "Warning":bool, " Fault":bool}
  T22 = cluster{"port ":u16, "remote address":string, "Connection timeout ms":i32, "Waiting for connection":bool, "Waiting for Command":bool, "timeout ms":i32}[]
  T23 = cluster{"High Stage manual speed control":bool, "Manual High stage frequency":dbl, "Low Stage manual speed control":bool, "Manual Low Stage frequency":dbl}
  T24 = cluster{"Software Version":string, "CPU Usage":dbl, "Memory Available":dbl, "SOM Storage(MB)":dbl, "SD card free space":dbl}
  T25 = typedef "GUI.lvlib/Profile Sequence.ctl" = cluster{"Duration":i32, "Head Load(W)":u32, "Name":string}[]
  T26 = cluster{"Refresh Seq":bool, "Save Seq":bool, "Delete Seq":bool, "Clear Seq":bool}
  T27 = typedef "GUI.lvlib/GUI Variables.ctl" = cluster{"Core":cluster{"Current VI":refnum<vi>, "Close Panel on Exit?":bool, "VI Name":string, "VI Path":path}, "Log?":bool, "Current Case":string, "Shared Variable Address":string, "reader endpoint":refnum<k21>, "writer endpoint":refnum<k21>, "Detected Systems":string[], "IP Address":string, "Network Connection":bool, "URI Directory":string, "File list in SoM":string[], "System State":enum16{"Idle", "Running"}, "TTV Test":cluster{"Power Seq":T25, "PS Connection":bool, "OutputState":bool, "Step":i32, "Current Cycle":i32}, "Profile":cluster{"Profile Temp":bool, "Current Cycle":i32}, "M1 History Temps":dbl[][], "M2 History Temps":dbl[][], "System Ready":bool, "M2 Bootup":bool, "Network Data Down":T28, "Event Log":T21[], "Login":bool, "Connected System":string, "TCP connection info":T30, "TCP Connection":bool, "Dataset":T32}
  T28 = typedef "GUI.lvlib/Network Data Down_set back.ctl" = cluster{"M1 Commands":cluster{"Set Temp":dbl, "Power Drive":bool, "Feedback":u8, "Package":u16, "Enable":bool}, "M2 Commands":cluster{"Set Temp":dbl, "Power Drive":bool, "Feedback":u8, "Package ":u16, "Enable":bool}, "Config Data":cluster{"Packages":cluster{"DUT Force lbf":cluster{" 0":u32, " 1":u32, " 2":u32, "3":u32, "4":u32, "5":u32, " 6":u32, "7":u32, "8":u32, "9":u32}, "DUT Names":cluster{"0":string, "1":string, "2":string, "3":string, "4":string, "5":string, "6":string, "7":string, "8":string, "9":string}}, "Heater PID":cluster{"P":dbl, "I":dbl, "D":dbl}, "Piston Settings":cluster{"Forces Slope":dbl, "Forces Intercept":dbl, "Transition Force":dbl, "Up Force":dbl, "Diameter (mm)":dbl, "Delay (ms)":dbl, "Pressure Ramp Delay (ms)":dbl}, "Safe Temps":cluster{"Minimum":i32, "Enabled":bool, "Maximum":i32}, "System Settings":cluster{"Number of Heads":i32, "60Hz Power":bool, "FTC200":bool, "AutoStartup":bool, "Purge":bool, "Sensors":bool, "HandClamp":bool, "ATE":bool, "Benchtop":bool, "Production":bool, "Refrigerant":enum16{"r404a", "r507", "r508", "r410a", "r134a"}, "Handler":bool, "Shuttle":bool, "220V":bool, "Cascade":bool, "Suction Sensor":enum16{"YCQB02H01", "YCQB02L01", "Carel"}, "Discharge Sensor":enum16{"YCQB05H01", "YCQB05L01", "Carel"}}, "Stepper Settings ":cluster{"Microstepping":enum16{"Full", "Half", "Quarter", "1/16th"}, "Velocity":u8}, "Set Point Range":cluster{"Max":dbl, "Min":dbl}, "Pedestal Check DeltaT":dbl, "Ramp Delta T":dbl, "Ramp-SS Threshold":dbl, "SS Tolerance":dbl, "EEV PID":cluster{"Ramp Up Target":dbl, "Ramp Down Target":dbl, "Steady State Target":dbl, "Output":cluster{"Max":dbl, "Min":dbl}, "EBB and Flow Temp TH":dbl, "Cryomode EEV Max":dbl, "Valve minimum opening ":dbl, "Ramp Up EEV Steps":dbl, "Ramp Down EEV Steps":dbl, "SS EEV Steps Reset":dbl, "EBB and Flow Tol":dbl, "Gains":cluster{"P":dbl, "I":dbl, "D":dbl}, "Dissabled Target":dbl, "CryoMode Gains":cluster{"P":dbl, "I":dbl, "D":dbl}, "M1 SuperHeat Setpoint":dbl, "M2 Gains":cluster{"P":dbl, "I":dbl, "D":dbl}, "Flow Curve":enum16{""}}, "Sleep Timeout":dbl, "Bypass Values":cluster{"Bypass Valve":bool, "Flow Curve":enum16{"0", "1"}, "Output":cluster{"Max":u32, "Min":u32}, "Feedback":enum16{"Temperature", "Pressure", "Superheat", "Pressure 2.0"}, "Cyth Bypass":bool, "PID":cluster{"P":dbl, "I":dbl, "D":dbl}, "Pressure setpoint":i16, "Cryo Temp":i16, "Superheat Setpoint":i16, "Cryo Setpoint":i16}, "Default Temp":dbl, "InTEC":cluster{"Enabled":bool, "IP":string, "Port":u16}, "M1 TSD":cluster{"Gain":dbl, "Offset":dbl, "V Offset ":dbl}, "M2 TSD":cluster{"Gain":dbl, "Offset":dbl, "V Offset ":dbl}, "M1 T-Case Calibration":cluster{"Gain":dbl, "Offset":dbl}, "M2 T-Case Calibration":cluster{"Gain":dbl, "Offset":dbl}, "Heater PID TSD":cluster{"P":dbl, "I":dbl, "D":dbl}, "M2 Heater PID":cluster{"P":dbl, "I":dbl, "D":dbl}}, "System Power On Off":bool, "New Data":T29, "Stop RT":bool}
  T29 = typedef "GUI.lvlib/NS New Data.ctl" = enum16{"M1 Set Point", "M1 Power Drive", "M1 Feedback", "M1 Package", "M1 Enable", "M2 Set Point", "M2 Power Drive", "M2 Feedback", "M2 Package", "M2 Enable", "System Power", "Config Data", "Stop RT"}
  T30 = typedef "NI STM.lvlib/TCP Connection Info.ctl" = cluster{"connection ID":refnum<k5>, "meta data":T31[]}
  T31 = typedef "NI STM.lvlib/MetaDataElement.ctl" = string
  T32 = typedef "GUI.lvlib/Dataset.ctl" = cluster{"System Status":T33, "M1 Status":T34, "M2 Status":T35, "Config Data":T36}
  T33 = typedef "GUI.lvlib/System Status.ctl" = cluster{"Power On Off":bool, "Discharge Temp":dbl, "Liquid Temp":dbl, "Suction Temp":dbl, "Ambient Temp":dbl, "Sleep":bool, "System Status":u16, "M1 Actuated":bool, "M2 Actuated":bool, "Sleep Timer":dbl, "M1 Bin":cluster{"Bin String":string, "Bin Color":u16}, "M2 Bin":cluster{"Bin String":string, "Bin Color":u16}, "Discharge Pressure":dbl, "Suction Pressure":dbl, "Compression Ratio":dbl, "Compressor Amps":dbl, "Compressor Hours":dbl, "Bypass Steps":u16, "SubCooling":dbl, "SuperHeat":dbl, "Serial Number":string, "EMO detected":bool, "EMO Tripped":bool, "Thermal cutoff":bool, "Thermal cutoff 2":bool, "High Pressure switch":bool, "Running Time":timestamp, "SOM Status":cluster{"Boot Up Time":timestamp, "Software Version":string, "CPU Usage":dbl, "Memory Available":dbl, "SD card free space":dbl, "SOM Storage":dbl}, "Cascade Extra":cluster{"Discharge Temp High Side":dbl, "Suction Temp High Side":dbl, "Liquid Temp High side":dbl, "Discharge Pressure 2":dbl, "Suction Pressure 2":dbl, "Low Side RPM":dbl, "High Side RPM":dbl}}
  T34 = typedef "GUI.lvlib/Module Status.ctl" = cluster{"Case Temp":dbl, "Evap Temp":dbl, "Heater %":dbl, "EEV Steps":u32, "Set Temp":dbl, "Feedback":u8, "Power Drive":bool, "Piston Volts":dbl, "Safe Temp":bool, "Power":bool, "Thermal State":u16, "Error":bool, "In tollerance":bool, "Head State":u16, "Piston Force":dbl, "Package":string, "Dynamic SV":dbl, "PV":dbl, "TSD Temp":dbl, "DC Load Watts":dbl, "AC Load Watts":dbl, "Intec Feedback":dbl}
  T35 = typedef "GUI.lvlib/M2 Status.ctl" = cluster{"Case Temp":dbl, "Evap Temp":dbl, "Heater %":dbl, "EEV Steps":u32, "Set Temp":dbl, "Feedback":u8, "Power Drive":bool, "Piston Volts":dbl, "Safe Temp":bool, "Power":bool, "Thermal State":u16, "Error":bool, "In tollerance":bool, "Head State":u16, "Piston Force":dbl, "Package":string, "PV":dbl, "Dynamic SV":dbl, "TSD":dbl, "AC Load Watts":dbl}
  T36 = typedef "GUI.lvlib/Config Data.ctl" = cluster{"Packages":cluster{"DUT Force lbf":cluster{" 0":u32, " 1":u32, " 2":u32, "3":u32, "4":u32, "5":u32, " 6":u32, "7":u32, "8":u32, "9":u32}, "DUT Names":cluster{"0":string, "1":string, "2":string, "3":string, "4":string, "5":string, "6":string, "7":string, "8":string, "9":string}}, "Heater PID":cluster{"P":dbl, "I":dbl, "D":dbl}, "Piston Settings":cluster{"Forces Slope":dbl, "Forces Intercept":dbl, "Transition Force":dbl, "Up Force":dbl, "Diameter (mm)":dbl, "Delay (ms)":dbl, "Pressure Ramp Delay (ms)":dbl}, "Safe Temps":cluster{"Minimum":i32, "Enabled":bool, "Maximum":i32}, "System Settings":cluster{"Number of Heads":i32, "60Hz Power":bool, "FTC200":bool, "AutoStartup":bool, "Purge":bool, "Sensors":bool, "HandClamp":bool, "ATE":bool, "Benchtop":bool, "Production":bool, "Refrigerant":u16, "Handler":bool, "Shuttle":bool, "220V":bool, "Cascade":bool, "Suction Sensor":u16, "Discharge Sensor":u16}, "Stepper Settings ":cluster{"Microstepping":u16, "Velocity":u8}, "Set Point Range":cluster{"Max":dbl, "Min":dbl}, "Pedestal Check DeltaT":dbl, "Ramp Delta T":dbl, "Ramp-SS Threshold":dbl, "SS Tolerance":dbl, "EEV PID":cluster{"Ramp Up Target":dbl, "Ramp Down Target":dbl, "Steady State Target":dbl, "Output":cluster{"Max":dbl, "Min":dbl}, "EBB and Flow Temp TH":dbl, "Cryomode EEV Max":dbl, "Valve minimum opening ":dbl, "Ramp Up EEV Steps":dbl, "Ramp Down EEV Steps":dbl, "SS EEV Steps Reset":dbl, "EBB and Flow Tol":dbl, "Gains":cluster{"P":dbl, "I":dbl, "D":dbl}, "Dissabled Target":dbl, "CryoMode Gains":cluster{"P":dbl, "I":dbl, "D":dbl}, "M1 SuperHeat Setpoint":dbl, "M2 Gains":cluster{"P":dbl, "I":dbl, "D":dbl}, "Flow Curve":u16}, "Sleep Timeout":dbl, "Bypass Values":cluster{"Bypass Valve":bool, "Flow Curve":u16, "Output":cluster{"Max":u32, "Min":u32}, "Feedback":u16, "Cyth Bypass":bool, "PID":cluster{"P":dbl, "I":dbl, "D":dbl}, "Pressure setpoint":i16, "Cryo Temp":i16, "Superheat Setpoint":i16, "Cryo Setpoint":i16}, "Default Temp":dbl, "InTEC":cluster{"Enabled":bool, "IP":string, "Port":u16}, "M1 TSD":cluster{"Gain":dbl, "Offset":dbl, "V Offset ":dbl}, "M2 TSD":cluster{"Gain":dbl, "Offset":dbl, "V Offset ":dbl}, "M1 T-Case Calibration":cluster{"Gain":dbl, "Offset":dbl}, "M2 T-Case Calibration":cluster{"Gain":dbl, "Offset":dbl}, "Heater PID TSD":cluster{"P":dbl, "I":dbl, "D":dbl}, "M2 Heater PID":cluster{"P":dbl, "I":dbl, "D":dbl}}
  T37 = typedef "GUI.lvlib/Messaging Actions.ctl" = enum16{"Create", "Get", "Destroy"}
  T38 = typedef "GUI.lvlib/Save Log State.ctl" = enum16{"Idle", "Init", "Write", "Exit"}
  T39 = enum32{"Invalid", "Standard", "Closed", "Hidden", "Minimized", "Maximized"}
  T40 = enum8{"Enabled", "Disabled", "Disabled and Grayed Out"}
  T41 = enum32{"Page Enabled", "Page Disabled", "Page Disabled & Grayed"}
  T42 = typedef "LVPositionTypeDef.ctl" = cluster{"Left":i32, "Top":i32}
  T43 = cluster{"Set Temp":dbl, "Power Drive":bool, "Feedback":u8, "Package":u16, "Enable":bool}
  T44 = typedef "GUI.lvlib/WebDAV states.ctl" = enum16{"Open Sess", "Refresh Dir", "Create Dir", "Upload", "Download", "Delete", "Close Sess"}
  T45 = typedef "NI STM.lvlib/TCP Read Options.ctl" = cluster{"ignore timeout error":bool, "timeout ms (1000)":i32}
  T46 = enum16{"Supervisor", "Engineer", "Operator", "Guest"}
  T47 = cluster{"baud rate":u32, "data bits":u16, "parity":enum16{"None", "Odd", "Even", "Mark", "Space"}, "stop bits":u16, "flow control":u16}
  T48 = enum16{"Start Timer", "Read Time", "Pause", "Resume"}
  T49 = cluster{"Boot Up Time":timestamp, "Software Version":string, "CPU Usage":dbl, "Memory Available":dbl, "SD card free space":dbl, "SOM Storage":dbl}
  T50 = cluster{"0":string, "1":string, "2":string, "3":string, "4":string, "5":string, "6":string, "7":string, "8":string, "9":string}
  T51 = typedef "NI_WebDAV.lvlib/SessionHandle.ctl" = refnum<k1>
  T52 = typedef "NI_WebDAV.lvlib/FileInfo.ctl" = cluster{"type":string, "size":u64, "last modification":timestamp, "display name":string, "uri":string}
  T53 = cluster{"Power On Off":bool, "Discharge Temp":dbl, "Liquid Temp":dbl, "Suction Temp":dbl, "Ambient Temp":dbl, "Sleep":bool, "System Status":u16, "M1 Actuated":bool, "M2 Actuated":bool, "Sleep Timer":dbl, "M1 Bin":cluster{"Bin String":string, "Bin Color":u16}, "M2 Bin":cluster{"Bin String":string, "Bin Color":u16}, "Discharge Pressure":dbl, "Suction Pressure":dbl, "Compression Ratio":dbl, "Compressor Amps":dbl, "Compressor Hours":dbl, "Bypass Steps":u16, "SubCooling":dbl, "SuperHeat":dbl, "Serial Number":string, "EMO detected":bool, "EMO Tripped":bool, "Thermal cutoff":bool, "Thermal cutoff 2":bool, "High Pressure switch":bool, "Running Time":string, "SOM Status":cluster{"Boot Up Time":string, "Software Version":string, "CPU Usage":dbl, "Memory Available":dbl, "SD card free space":dbl, "SOM Storage":dbl}, "Cascade Extra":cluster{"Discharge Temp High Side":dbl, "Suction Temp High Side":dbl, "Liquid Temp High side":dbl, "Discharge Pressure 2":dbl, "Suction Pressure 2":dbl, "Low Side RPM":dbl, "High Side RPM":dbl}}
  T54 = cluster{"DUT Force lbf":cluster{" 0":u32, " 1":u32, " 2":u32, "3":u32, "4":u32, "5":u32, " 6":u32, "7":u32, "8":u32, "9":u32}, "DUT Names":cluster{"0":string, "1":string, "2":string, "3":string, "4":string, "5":string, "6":string, "7":string, "8":string, "9":string}}
  T55 = cluster{"Force - pounds":cluster{" 0":u32, " 1":u32, " 2":u32, "3":u32, "4":u32, "5":u32, " 6":u32, "7":u32, "8":u32, "9":u32}, "DUT Names":cluster{"0":string, "1":string, "2":string, "3":string, "4":string, "5":string, "6":string, "7":string, "8":string, "9":string}}
  T56 = enum16{"Left Button", "Center Button", "Right Button", "Window Close"}
  T57 = cluster{"Duration":i32, "Head Load(W)":u32, "Name":string}
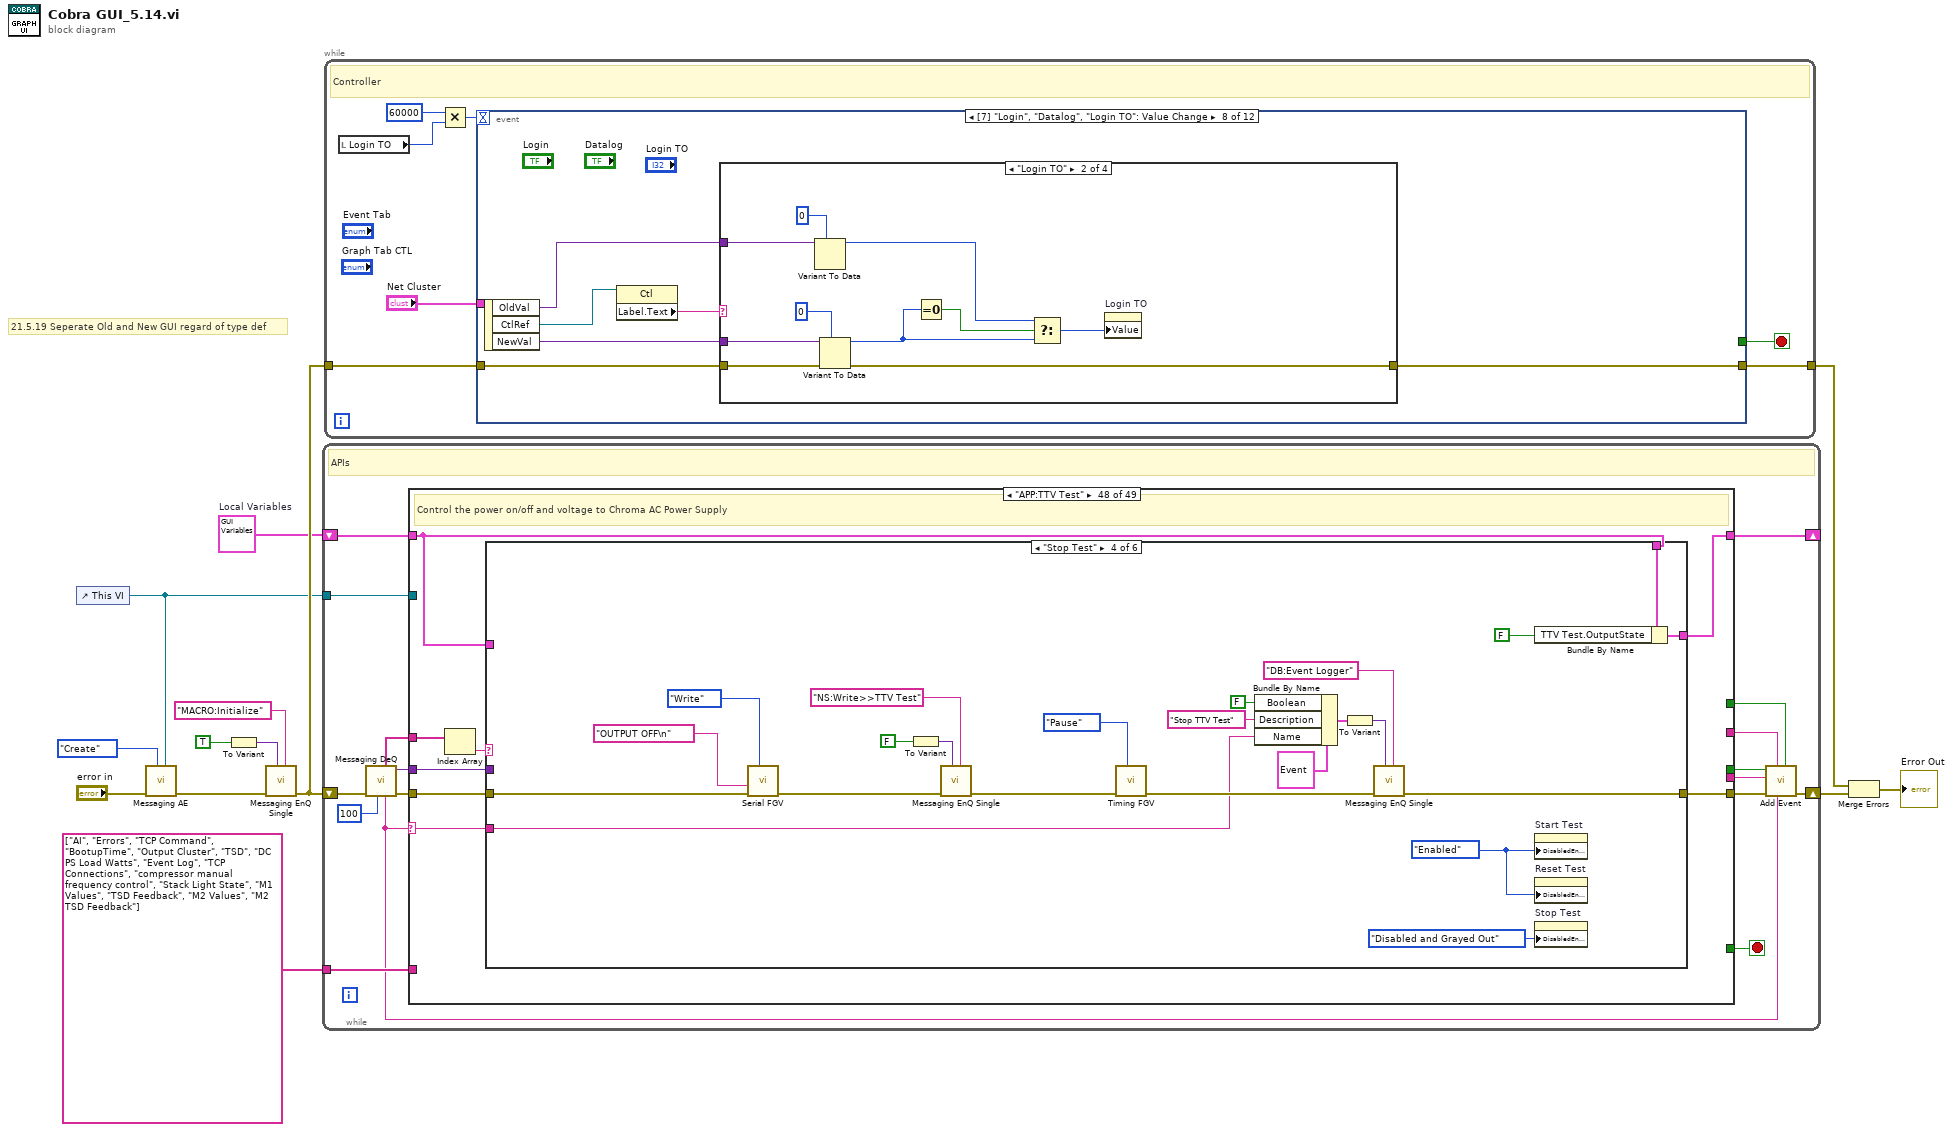
[diagram p0: block diagram]
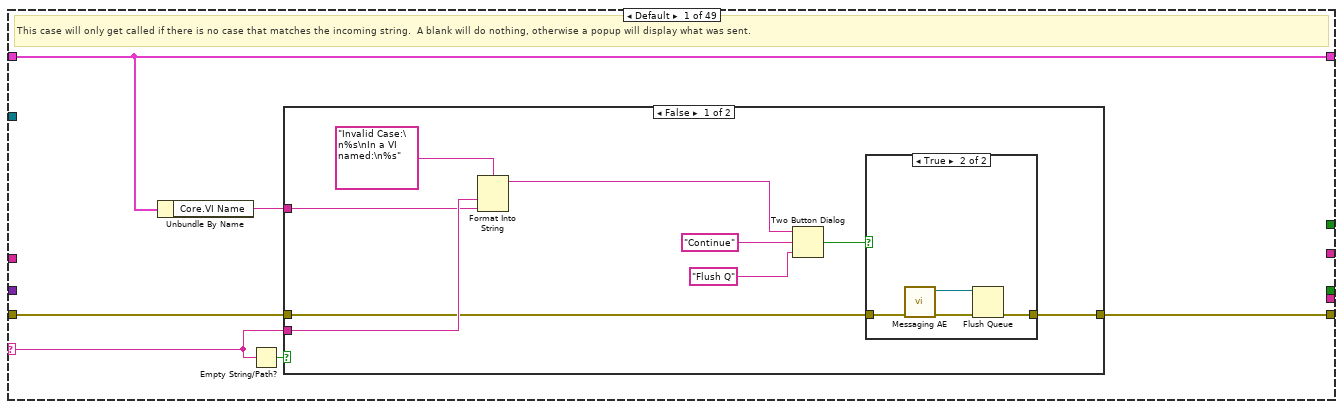
[diagram p2: hidden frame]
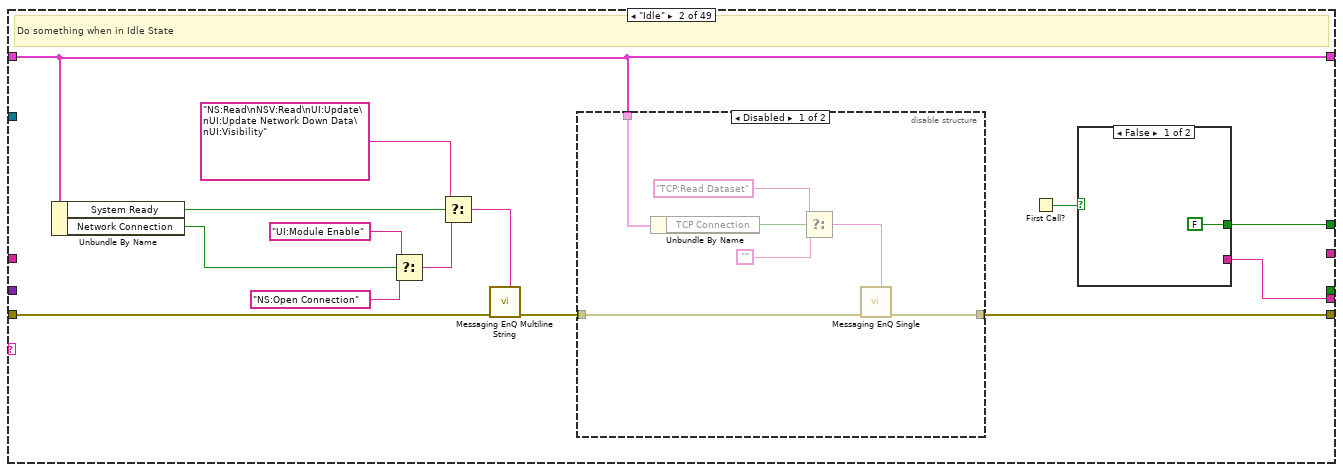
[diagram p5: hidden frame]
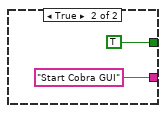
[diagram p7: hidden frame]
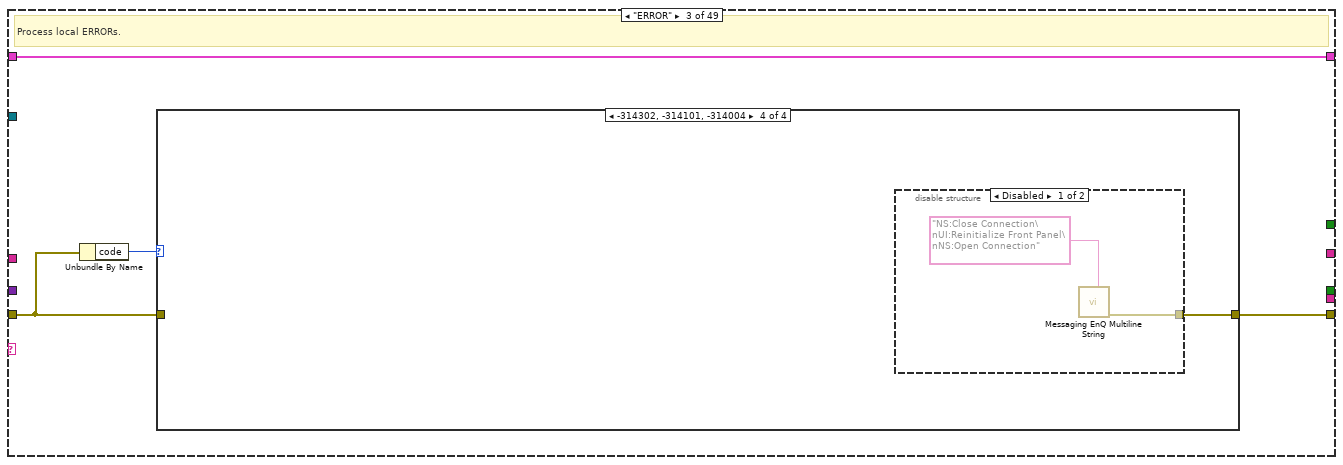
[diagram p8: hidden frame]
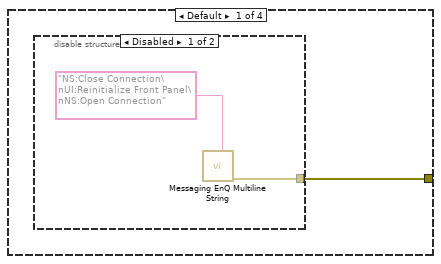
[diagram p9: hidden frame]
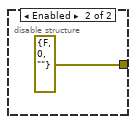
[diagram p10: hidden frame]
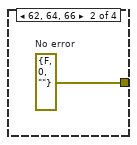
[diagram p11: hidden frame]
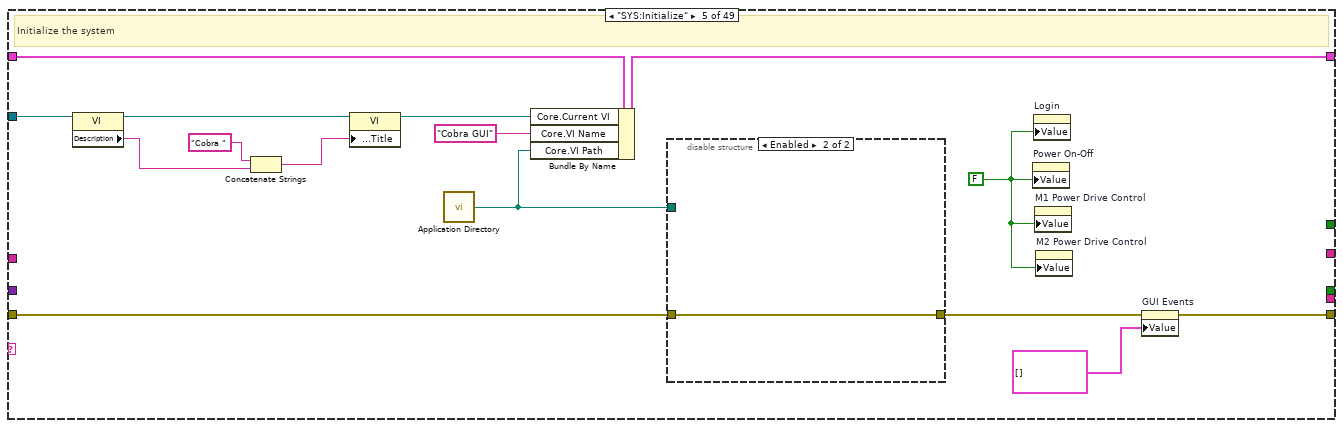
[diagram p15: hidden frame]
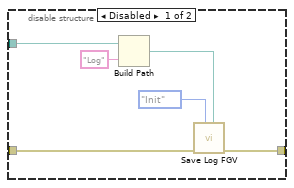
[diagram p16: hidden frame]
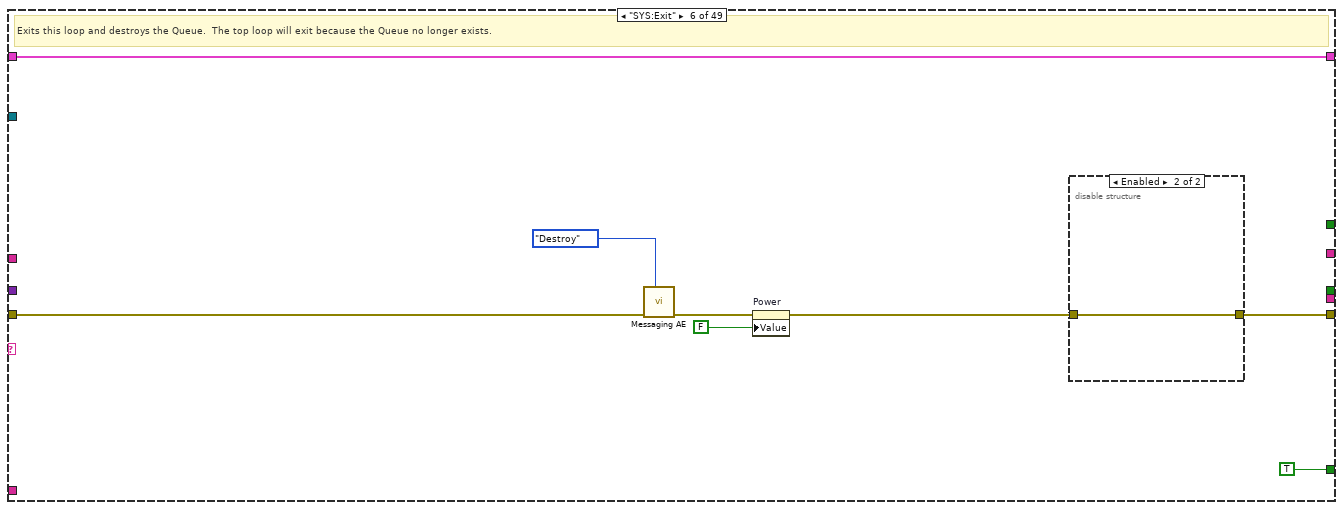
[diagram p17: hidden frame]
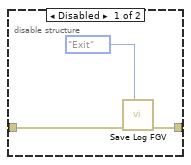
[diagram p18: hidden frame]
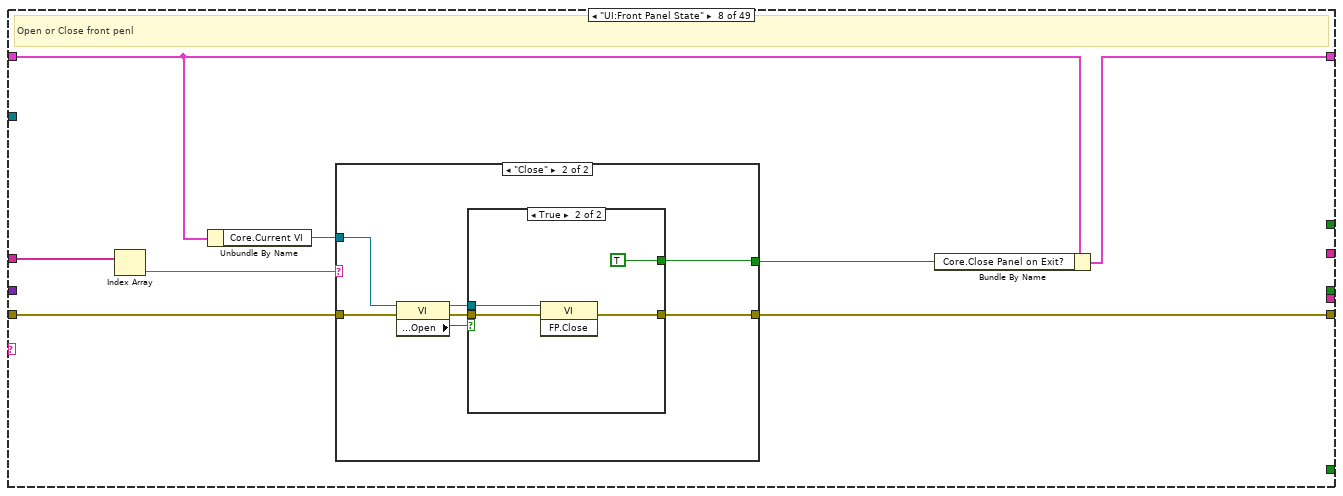
[diagram p20: hidden frame]
diagram:
  w2 = T27 {"Core"={"Current VI"=refnum, "Close Panel on Exit?"=FALSE, "VI Name"="", "VI Path"=path ""}, "Log?"=FALSE, "Current Case"="", "Shared Variable Address"="", "reader endpoint"="", "writer endpoint"="", "Detected Systems"=[], "IP Address"="", "Network Connection"=FALSE, "URI Directory"="", "File list in SoM"=[], "System State"=enum."Idle", "TTV Test"={"Power Seq"=[], "PS Connection"=FALSE, "OutputState"=FALSE, "Step"=0, "Current Cycle"=0}, "Profile"={"Profile Temp"=FALSE, "Current Cycle"=0}, "M1 History Temps"=[], "M2 History Temps"=[], "System Ready"=FALSE, "M2 Bootup"=FALSE, "Network Data Down"={"M1 Commands"={"Set Temp"=20.0, "Power Drive"=FALSE, "Feedback"=1, "Package"=0, "Enable"=FALSE}, "M2 Commands"={"Set Temp"=20.0, "Power Drive"=FALSE, "Feedback"=1, "Package "=0, "Enable"=FALSE}, "Config Data"={"Packages"={"DUT Force lbf"={" 0"=0, " 1"=0, " 2"=0, "3"=0, "4"=0, "5"=0, " 6"=0, "7"=0, "8"=0, "9"=0}, "DUT Names"={"0"="", "1"="", "2"="", "3"="", "4"="", "5"="", "6"="", "7"="", "8"="", "9"=""}}, "Heater PID"={"P"=0.0, "I"=0.0, "D"=0.0}, "Piston Settings"={"Forces Slope"=0.0, "Forces Intercept"=0.0, "Transition Force"=0.0, "Up Force"=0.0, "Diameter (mm)"=0.0, "Delay (ms)"=0.0, "Pressure Ramp Delay (ms)"=0.0}, "Safe Temps"={"Minimum"=17, "Enabled"=TRUE, "Maximum"=95}, "System Settings"={"Number of Heads"=0, "60Hz Power"=TRUE, "FTC200"=TRUE, "AutoStartup"=FALSE, "Purge"=TRUE, "Sensors"=TRUE, "HandClamp"=TRUE, "ATE"=TRUE, "Benchtop"=TRUE, "Production"=TRUE, "Refrigerant"=enum."r404a", "Handler"=TRUE, "Shuttle"=TRUE, "220V"=FALSE, "Cascade"=FALSE, "Suction Sensor"=enum."YCQB02H01", "Discharge Sensor"=enum."YCQB05H01"}, "Stepper Settings "={"Microstepping"=enum."Full", "Velocity"=8}, "Set Point Range"={"Max"=0.0, "Min"=0.0}, "Pedestal Check DeltaT"=0.0, "Ramp Delta T"=0.0, "Ramp-SS Threshold"=0.0, "SS Tolerance"=0.0, "EEV PID"={"Ramp Up Target"=0.0, "Ramp Down Target"=0.0, "Steady State Target"=0.0, "Output"={"Max"=0.0, "Min"=0.0}, "EBB and Flow Temp TH"=0.0, "Cryomode EEV Max"=0.0, "Valve minimum opening "=0.0, "Ramp Up EEV Steps"=0.0, "Ramp Down EEV Steps"=0.0, "SS EEV Steps Reset"=0.0, "EBB and Flow Tol"=0.0, "Gains"={"P"=0.0, "I"=0.0, "D"=0.0}, "Dissabled Target"=0.0, "CryoMode Gains"={"P"=0.0, "I"=0.0, "D"=0.0}, "M1 SuperHeat Setpoint"=0.0, "M2 Gains"={"P"=0.0, "I"=0.0, "D"=0.0}, "Flow Curve"=enum.""}, "Sleep Timeout"=0.0, "Bypass Values"={"Bypass Valve"=TRUE, "Flow Curve"=enum."0", "Output"={"Max"=0, "Min"=0}, "Feedback"=enum."Temperature", "Cyth Bypass"=TRUE, "PID"={"P"=0.0, "I"=0.0, "D"=0.0}, "Pressure setpoint"=0, "Cryo Temp"=0, "Superheat Setpoint"=0, "Cryo Setpoint"=0}, "Default Temp"=0.0, "InTEC"={"Enabled"=FALSE, "IP"="192.168.1.100", "Port"=5000}, "M1 TSD"={"Gain"=0.0, "Offset"=0.0, "V Offset "=0.0}, "M2 TSD"={"Gain"=0.0, "Offset"=0.0, "V Offset "=0.0}, "M1 T-Case Calibration"={"Gain"=0.0, "Offset"=0.0}, "M2 T-Case Calibration"={"Gain"=0.0, "Offset"=0.0}, "Heater PID TSD"={"P"=0.0, "I"=0.0, "D"=0.0}, "M2 Heater PID"={"P"=0.0, "I"=0.0, "D"=0.0}}, "System Power On Off"=FALSE, "New Data"=enum."M1 Set Point", "Stop RT"=FALSE}, "Event Log"=[], "Login"=FALSE, "Connected System"="", "TCP connection info"={"connection ID"=refnum, "meta data"=[]}, "TCP Connection"=FALSE, "Dataset"={"System Status"={"Power On Off"=FALSE, "Discharge Temp"=0.0, "Liquid Temp"=0.0, "Suction Temp"=0.0, "Ambient Temp"=0.0, "Sleep"=FALSE, "System Status"=0, "M1 Actuated"=FALSE, "M2 Actuated"=FALSE, "Sleep Timer"=0.0, "M1 Bin"={"Bin String"="", "Bin Color"=1}, "M2 Bin"={"Bin String"="", "Bin Color"=1}, "Discharge Pressure"=0.0, "Suction Pressure"=0.0, "Compression Ratio"=0.0, "Compressor Amps"=0.0, "Compressor Hours"=0.0, "Bypass Steps"=0, "SubCooling"=0.0, "SuperHeat"=0.0, "Serial Number"="", "EMO detected"=FALSE, "EMO Tripped"=FALSE, "Thermal cutoff"=FALSE, "Thermal cutoff 2"=FALSE, "High Pressure switch"=FALSE, "Running Time"=timestamp(0 s since 1904-01-01), "SOM Status"={"Boot Up Time"=timestamp(0 s since 1904-01-01), "Software Version"="", "CPU Usage"=0.0, "Memory Available"=0.0, "SD card free space"=0.0, "SOM Storage"=0.0}, "Cascade Extra"={"Discharge Temp High Side"=0.0, "Suction Temp High Side"=0.0, "Liquid Temp High side"=0.0, "Discharge Pressure 2"=0.0, "Suction Pressure 2"=0.0, "Low Side RPM"=0.0, "High Side RPM"=0.0}}, "M1 Status"={"Case Temp"=0.0, "Evap Temp"=0.0, "Heater %"=0.0, "EEV Steps"=0, "Set Temp"=0.0, "Feedback"=0, "Power Drive"=FALSE, "Piston Volts"=0.0, "Safe Temp"=FALSE, "Power"=FALSE, "Thermal State"=0, "Error"=FALSE, "In tollerance"=FALSE, "Head State"=0, "Piston Force"=0.0, "Package"="", "Dynamic SV"=0.0, "PV"=0.0, "TSD Temp"=0.0, "DC Load Watts"=0.0, "AC Load Watts"=0.0, "Intec Feedback"=0.0}, "M2 Status"={"Case Temp"=0.0, "Evap Temp"=0.0, "Heater %"=0.0, "EEV Steps"=0, "Set Temp"=0.0, "Feedback"=0, "Power Drive"=FALSE, "Piston Volts"=0.0, "Safe Temp"=FALSE, "Power"=FALSE, "Thermal State"=0, "Error"=FALSE, "In tollerance"=FALSE, "Head State"=0, "Piston Force"=0.0, "Package"="", "PV"=0.0, "Dynamic SV"=0.0, "TSD"=0.0, "AC Load Watts"=0.0}, "Config Data"={"Packages"={"DUT Force lbf"={" 0"=0, " 1"=0, " 2"=0, "3"=0, "4"=0, "5"=0, " 6"=0, "7"=0, "8"=0, "9"=0}, "DUT Names"={"0"="", "1"="", "2"="", "3"="", "4"="", "5"="", "6"="", "7"="", "8"="", "9"=""}}, "Heater PID"={"P"=0.0, "I"=0.0, "D"=0.0}, "Piston Settings"={"Forces Slope"=0.0, "Forces Intercept"=0.0, "Transition Force"=0.0, "Up Force"=0.0, "Diameter (mm)"=0.0, "Delay (ms)"=0.0, "Pressure Ramp Delay (ms)"=0.0}, "Safe Temps"={"Minimum"=17, "Enabled"=TRUE, "Maximum"=95}, "System Settings"={"Number of Heads"=0, "60Hz Power"=TRUE, "FTC200"=TRUE, "AutoStartup"=FALSE, "Purge"=TRUE, "Sensors"=TRUE, "HandClamp"=TRUE, "ATE"=TRUE, "Benchtop"=TRUE, "Production"=TRUE, "Refrigerant"=0, "Handler"=TRUE, "Shuttle"=TRUE, "220V"=FALSE, "Cascade"=FALSE, "Suction Sensor"=0, "Discharge Sensor"=0}, "Stepper Settings "={"Microstepping"=0, "Velocity"=8}, "Set Point Range"={"Max"=0.0, "Min"=0.0}, "Pedestal Check DeltaT"=0.0, "Ramp Delta T"=0.0, "Ramp-SS Threshold"=0.0, "SS Tolerance"=0.0, "EEV PID"={"Ramp Up Target"=0.0, "Ramp Down Target"=0.0, "Steady State Target"=0.0, "Output"={"Max"=0.0, "Min"=0.0}, "EBB and Flow Temp TH"=0.0, "Cryomode EEV Max"=0.0, "Valve minimum opening "=0.0, "Ramp Up EEV Steps"=0.0, "Ramp Down EEV Steps"=0.0, "SS EEV Steps Reset"=0.0, "EBB and Flow Tol"=0.0, "Gains"={"P"=0.0, "I"=0.0, "D"=0.0}, "Dissabled Target"=0.0, "CryoMode Gains"={"P"=0.0, "I"=0.0, "D"=0.0}, "M1 SuperHeat Setpoint"=0.0, "M2 Gains"={"P"=0.0, "I"=0.0, "D"=0.0}, "Flow Curve"=0}, "Sleep Timeout"=0.0, "Bypass Values"={"Bypass Valve"=TRUE, "Flow Curve"=0, "Output"={"Max"=0, "Min"=0}, "Feedback"=0, "Cyth Bypass"=TRUE, "PID"={"P"=0.0, "I"=0.0, "D"=0.0}, "Pressure setpoint"=0, "Cryo Temp"=0, "Superheat Setpoint"=0, "Cryo Setpoint"=0}, "Default Temp"=0.0, "InTEC"={"Enabled"=FALSE, "IP"="192.168.1.100", "Port"=5000}, "M1 TSD"={"Gain"=0.0, "Offset"=0.0, "V Offset "=0.0}, "M2 TSD"={"Gain"=0.0, "Offset"=0.0, "V Offset "=0.0}, "M1 T-Case Calibration"={"Gain"=0.0, "Offset"=0.0}, "M2 T-Case Calibration"={"Gain"=0.0, "Offset"=0.0}, "Heater PID TSD"={"P"=0.0, "I"=0.0, "D"=0.0}, "M2 Heater PID"={"P"=0.0, "I"=0.0, "D"=0.0}}}}  # Local Variables
  # "21.5.19 Seperate Old and New GUI regard of type def"
  n1 = control-ref of="This VI"() -> (w1:refnum<vi>)
  n2 = call "Messaging AE.vi"("VI Refnum"=w1, "Action"=Messaging_Actions."Create", "Error In"="error in") -> ("Error Out"=w6:errorcluster)  [unwired: 7 in, 1 out]
  n3 = To Variant(anything=TRUE ("kill")) -> (Variant=w8:variant)
  n4 = call "Messaging EnQ Single.vi"("Command"="MACRO:Initialize", "Data"=w8, "error in (no error)"=w6) -> ("error out"=w10:errorcluster)  [unwired: 8 in]
  n5 = while {
    shift-right: [w20] -> w12
    shift-left: w10 -> [w29]
    shift-right: [w27] -> _
    shift-left: w2 -> [w23]
    tunnel: string[] ["AI", "Errors", "TCP Command", "BootupTime", "Output Cluster", "TSD", "DC PS Load Watts", "Event Log", "TCP Connections", "compressor manual frequency control", "Stack Light State", "M1 Values", "TSD Feedback", "M2 Values", "M2 TSD Feedback"] -> [w22]
    tunnel: w1 -> [w14]
    stop <- w30 stop-if-true
    # "APIs"
    n6 = call "Messaging DeQ.vi"("Time out"=100 ("SV Update Rate"), "Error In"=w29) -> ("error out"=w28:errorcluster, "Data"=w25:variant, "Command"=w19:string, "[String Data]"=w24:string[])  [unwired: 6 in]
    n7 = case shown="\"APP:TTV Test\"" w19 {
      selector: w19 -> [w32 _ _ _ _ _ _ _ _ _ _ _ _ _ _ _ _ _ _ _ _ _ _ _ _ _ _ _ _ _ _ _ _ _ _ _ _ _ _ _ _ _ _ w1752 _ _ _ w1976 _]
      tunnel: w28 -> [w34 w65 w77 w90 w105 w117 w126 w134 w163 w517 w546 w552 w622 w631 w678 w683 w707 w745 w807 w826 w834 w854 w858 w862 w871 w885 w905 w924 w937 w983 w1168 w1175 w1285 w1434 w1445 w1474 w1477 w1490 w1504 w1593 w1712 w1716 w1732 w1760 w1771 w1773 w1804 w1981 w2303]
      tunnel: [w33 w60 w78 w90 w101 w116 w126 w133 w163 w510 w531 w550 w602 w644 w678 w682 w716 w745 w807 w809 w830 w842 w857 w862 w867 w876 w892 w920 w938 w989 w1168 w1173 w1284 w1434 w1442 w1473 w1477 w1482 w1499 w1597 w1705 w1716 w1733 w1755 w1771 w1781 w1801 w1979 w2305] -> w21
      tunnel: [_ _ _ _ _ TRUE _ _ _ _ _ _ _ _ _ _ _ _ _ _ _ _ _ _ _ _ _ _ _ _ _ _ _ _ _ _ _ _ _ _ _ _ _ _ _ _ _ _ _] -> w30
      tunnel: [w31 w53 w76 w89 w98 w118 w125 w128 w162 w520 w547 w551 w620 w647 w663 w704 w708 w746 w806 w808 w837 w853 w859 w861 w869 w883 w894 w918 w940 w981 w1167 w1179 w1288 w1433 w1446 w1471 w1476 w1484 w1495 w1596 w1711 w1715 w1728 w1756 w1770 w1780 w1800 w1978 w2306] -> w27
      tunnel: w23 -> [w31 w53 w76 w89 w99 w118 w125 w129 w161 w520 w547 w551 w619 w647 w662 w684 w708 w746 w806 w808 w837 w853 w859 w861 w870 w881 w902 w919 w931 w982 w1167 w1179 w1288 w1433 w1448 w1471 w1476 w1485 w1496 w1596 w1711 w1715 w1729 w1761 w1770 w1780 w1799 w1977 w2306]
      tunnel: w24 -> [_ _ _ _ _ _ _ w132 _ _ _ _ _ _ _ _ _ _ _ _ _ _ _ _ _ _ _ _ _ w993 _ w1176 _ _ _ _ _ _ _ w1594 _ _ _ _ _ w1779 w1808 w1983 _]
      tunnel: w25 -> [_ _ _ _ _ _ _ _ _ w516 w545 _ w621 _ _ _ _ _ _ w824 w835 _ _ _ _ w884 _ _ _ w984 _ w1174 _ _ _ _ _ _ _ w1592 _ _ w1731 w1759 _ _ w1805 w1980 _]
      tunnel: w22 -> [_ _ _ _ _ _ _ _ _ _ _ _ _ _ _ _ _ _ _ _ _ _ _ _ _ _ _ _ _ _ _ _ w1286 _ _ _ _ _ _ _ _ _ _ _ _ _ _ _ _]
      tunnel: [_ w63 _ _ _ _ _ _ _ _ _ _ _ _ _ w679 _ _ _ _ _ _ TRUE ("Boolean") _ _ _ w886 _ w929 TRUE ("Connected") _ TRUE ("Connected") _ _ TRUE ("Connected") TRUE ("Connected") _ TRUE ("Visible") _ TRUE ("Visible") TRUE ("Visible") _ w1721 _ _ _ _ _ _] -> w18
      tunnel: [_ _ _ _ _ _ _ _ _ _ _ _ _ _ _ w679 _ _ _ _ _ _ _ _ _ _ w886 _ w928 _ _ w1169 _ _ _ _ _ TRUE ("TSD Feedback") _ w1589 _ _ _ _ _ _ _ _ _] -> w17
      tunnel: [_ w62 _ _ _ _ _ _ _ _ _ _ _ _ _ "System Ready" ("Command") _ _ _ _ _ _ "Stop Cobra GUI" ("String") _ _ _ w893 _ w927 w979 _ w1171 _ _ w1436 w1469 _ "Open a TCP port " ("Name") _ w1590 "Close the connected client" ("Name") _ w1719 _ _ _ _ _ _] -> w16
      tunnel: [_ _ _ _ _ _ _ _ _ _ _ _ _ _ _ _ _ _ _ _ _ _ _ _ _ _ _ _ _ w978 _ w1170 _ _ _ _ _ w1483 _ w1586 _ _ _ _ _ _ _ _ _] -> w15
      tunnel: w14 -> [_ _ _ _ w95 _ _ _ _ _ _ _ _ _ _ _ _ _ _ _ _ _ _ _ _ _ _ _ _ _ _ _ _ _ _ _ _ _ _ _ _ _ _ _ _ _ _ _ _]
      frame Default {
        # "This case will only get called if there is no case that matches the incoming string.  A blank will do nothing, otherwise a popup will display what was sent."
        n8 = Unbundle By Name(w31) -> ("Core.VI Name"=w35:string)
        n9 = Empty String/Path?(string/path=w32) -> (empty?=w36:bool)
        n10 = case shown="False" w36 {
          tunnel: [w44 w51] -> w33
          tunnel: w34 -> [w37 w51]
          tunnel: w32 -> [w39 _]
          tunnel: w35 -> [w38 _]
          frame False {
            n11 = Format Into String(format string="Invalid Case:\n%s\nIn a VI named:\n%s", w39, w38) -> (resulting string=w41:string)  [unwired: 2 in, 1 out]
            n12 = Two Button Dialog(message=w41, 1:"Flush Q" ("T button name (\"OK\")"), 2:"Continue" ("T button name (\"OK\")")) -> (T button?=w45:bool)
            n13 = case shown="True" w45 {
              tunnel: w37 -> [w46 w49]
              tunnel: [w46 w50] -> w44
              frame False {
              }
              frame True {
                n14 = call "Messaging AE.vi"("Error In"=w49) -> ("Error Out"=w48:errorcluster, "queue out"=w47:refnum<queue>)  [unwired: 9 in]
                n15 = Flush Queue(queue=w47, error in (no error)=w48) -> (error out=w50:errorcluster)  [unwired: 2 out]
              }
            }
          }
          frame True {
          }
        }
      }
      frame "Idle" {
        # "Do something when in Idle State"
        n16 = Unbundle By Name(w53) -> ("System Ready"=w54:bool, "Network Connection"=w56:bool)
        n17 = Select(t="UI:Module Enable" ("Command"), s=w56, f="NS:Open Connection" ("Command")) -> (s? t:f=w57:string)
        n18 = Select(t="NS:Read\nNSV:Read\nUI:Update\nUI:Update Network Down Data\nUI:Visibility" ("Command(s)"), s=w54, f=w57) -> (s? t:f=w52:string)
        n19 = call "Messaging EnQ Multiline String.vi"("Command(s)"=w52, "error in (no error)"=w65) -> ("error out"=w61:errorcluster)  [unwired: 9 in]
        n20 = disable-structure shown="Disabled" {
          disable-tunnel: w61 -> [w72 _]
          disable-tunnel: [w71 _] -> w60
          disable-tunnel: w53 -> [w66 _]
          frame Disabled {
            n21 = Unbundle By Name(w66) -> ("TCP Connection"=w70:bool)
            n22 = Select(t="TCP:Read Dataset" ("Command"), s=w70, f="") -> (s? t:f=w67:string)
            n23 = call "Messaging EnQ Single.vi"("Command"=w67, "error in (no error)"=w72) -> ("error out"=w71:errorcluster)  [unwired: 9 in]
          }
          frame Enabled {
          }
        }
        n24 = First Call?() -> (First Call?: T/F=w64:bool)
        n25 = case shown="False" w64 {
          tunnel: [FALSE ("Boolean") TRUE ("Boolean")] -> w63
          tunnel: [_ "Start Cobra GUI" ("String")] -> w62
          frame False {
          }
          frame True {
          }
        }
      }
      frame "ERROR" {
        # "Process local ERRORs."
        n26 = Unbundle By Name(w77) -> ("code"=w79:i32)
        n27 = case shown="-314302, -314101, -314004" w79 {
          tunnel: [w80 w84 w85 w86] -> w78
          tunnel: w77 -> [_ _ w85 _]
          frame Default {
            n28 = disable-structure shown="Disabled" {
              disable-tunnel: [w81 errorcluster {"status"=FALSE, "code"=0, "source"=""} ("error out")] -> w80
              frame Disabled {
                n29 = call "Messaging EnQ Multiline String.vi"("Command(s)"="NS:Close Connection\nUI:Reinitialize Front Panel\nNS:Open Connection" ("Command")) -> ("error out"=w81:errorcluster)  [unwired: 10 in]
              }
              frame Enabled {
              }
            }
          }
          frame 62, 64, 66 {
            w84 = errorcluster {"status"=FALSE, "code"=0, "source"=""}  # No error
          }
          frame -1950679035 {
          }
          frame -314302, -314101, -314004 {
            n30 = disable-structure shown="Disabled" {
              disable-tunnel: [w88 _] -> w86
              frame Disabled {
                n31 = call "Messaging EnQ Multiline String.vi"("Command(s)"="NS:Close Connection\nUI:Reinitialize Front Panel\nNS:Open Connection" ("Command")) -> ("error out"=w88:errorcluster)  [unwired: 10 in]
              }
              frame Enabled {
              }
            }
          }
        }
      }
      frame "-----System-----" {
        # "Command Format:\nCAT:Command>>Data1,Data2,DataN"
        # "SYSTEM is used for things that directly effect this module"
      }
      frame "SYS:Initialize" {
        w104 = FALSE ("Power On-Off")
        # "Initialize the system"
        n32 = property class="VI"(reference=w95) -> (reference out=w94:refnum<vi>, "Description"=w91:string)  [unwired: 1 in, 1 out]
        n33 = Concatenate Strings("Cobra " ("initial string"), w91) -> (w92:string)
        n34 = property class="VI"(reference=w94, "Front Panel.Title"=w92) -> (reference out=w96:refnum<vi>)  [unwired: 1 in, 1 out]
        n35 = call <vilib>:"Application Directory.vi"() -> ("Application Directory"=w97:path)
        n36 = Bundle By Name(cluster=w99, "Core.Current VI"=w96, "Core.VI Name"="Cobra GUI" ("VI Name"), "Core.VI Path"=w97) -> (w98:T27)
        n37 = disable-structure shown="Enabled" {
          disable-tunnel: w105 -> [w110 w112]
          disable-tunnel: [w107 w112] -> w102
          disable-tunnel: w97 -> [w106 _]
          frame Disabled {
            n38 = Build Path(base path=w106, name or relative path="Log") -> (appended path=w108:path)
            n39 = call "Save Log FGV.vi"("Log Path"=w108, "State"=Save_Log_State."Init", "Error In"=w110) -> ("Error Out"=w107:errorcluster)  [unwired: 8 in]
          }
          frame Enabled {
          }
        }
        n40 = property on="Power On-Off" class="Bool (strict)"("Value"=w104) -> ()  [unwired: 2 in, 2 out]
        n41 = property on="Login" class="Bool (strict)"("Value"=w104) -> ()  [unwired: 2 in, 2 out]
        n42 = property on="M1 Power Drive Control" class="Bool (strict)"("Value"=w104) -> ()  [unwired: 2 in, 2 out]
        n43 = property on="M2 Power Drive Control" class="Bool (strict)"("Value"=w104) -> ()  [unwired: 2 in, 2 out]
        n44 = property on="GUI Events" class="Arr (strict)"(error in=w102, "Value"=T21[] [] ("GUI Events")) -> (error out=w101:errorcluster)  [unwired: 1 in, 1 out]
      }
      frame "SYS:Exit" {
        # "Exits this loop and destroys the Queue.  The top loop will exit because the Queue no longer exists."
        n45 = call "Messaging AE.vi"("Action"=Messaging_Actions."Destroy", "Error In"=w117) -> ("Error Out"=w114:errorcluster)  [unwired: 8 in, 1 out]
        n46 = property on="Power" class="Bool (strict)"(error in=w114, "Value"=FALSE ("Value (Signaling)")) -> (error out=w113:errorcluster)  [unwired: 1 in, 1 out]
        n47 = disable-structure shown="Enabled" {
          disable-tunnel: [w123 w124] -> w116
          disable-tunnel: w113 -> [w121 w124]
          frame Disabled {
            n48 = call "Save Log FGV.vi"("State"=Save_Log_State."Exit", "Error In"=w121) -> ("Error Out"=w123:errorcluster)  [unwired: 9 in]
          }
          frame Enabled {
          }
        }
      }
      frame "-----User Interface-----" {
        # "UI is used for things that will change the UI.,"
      }
      frame "UI:Front Panel State" {
        # "Open or Close front penl"
        n49 = Index Array(array=w132) -> (element=w131:string)  [unwired: 1 in]
        n50 = Unbundle By Name(w129) -> ("Core.Current VI"=w130:refnum<vi>)
        n51 = case shown="\"Close\"" w131 {
          tunnel: w134 -> [w139 w153]
          tunnel: [w141 w154] -> w133
          tunnel: w130 -> [w140 w151]
          tunnel: [FALSE ("Core.Close Panel on Exit?") w148] -> w127
          frame "Open", Default {
            n52 = property class="VI"(reference=w140, error in=w139) -> (reference out=w137:refnum<vi>, error out=w138:errorcluster, "Front Panel.Open"=w136:bool)
            n53 = case shown="False" w136 {
              tunnel: [w144 w147] -> w141
              tunnel: w138 -> [w143 w147]
              tunnel: w137 -> [w142 _]
              frame False {
                n54 = invoke class="VI" method="FP.Open"(reference=w142, error in=w143, "Activate"=TRUE, "State"=T39."Standard") -> (error out=w144:errorcluster)  [unwired: 1 in, 4 out]
              }
              frame True {
              }
            }
          }
          frame "Close" {
            n55 = property class="VI"(reference=w151, error in=w153) -> (reference out=w150:refnum<vi>, error out=w152:errorcluster, "Front Panel.Open"=w149:bool)
            n56 = case shown="True" w149 {
              tunnel: [w156 w160] -> w154
              tunnel: w152 -> [w156 w159]
              tunnel: w150 -> [_ w158]
              tunnel: [FALSE ("Core.Close Panel on Exit?") TRUE ("Core.Close Panel on Exit?")] -> w148
              frame False {
              }
              frame True {
                n57 = invoke class="VI" method="FP.Close"(reference=w158, error in=w159) -> (error out=w160:errorcluster)  [unwired: 1 in, 2 out]
              }
            }
          }
        }
        n58 = Bundle By Name(cluster=w129, "Core.Close Panel on Exit?"=w127) -> (w128:T27)
      }
      frame "UI:Update" {
        n59 = stacked-sequence {
          tunnel: w161 -> [w169 w198 w217 w244 w272 w309 w357 w379 w456 w488]
          tunnel: w161 -> [_ _ _ _ _ _ _ w403 _ _]
          tunnel: [_ _ _ _ _ _ _ w402 _ _] -> w162
          frame #0 {
            # "Update System Module Data"
            n60 = Unbundle By Name(w169) -> ("Dataset.System Status"=w176:T33)
            n61 = Unbundle By Name(w176) -> ("Compression Ratio"=w173:dbl, "Compressor Amps"=w172:dbl, "Discharge Pressure"=w171:dbl, "Suction Pressure"=w170:dbl, "SubCooling"=w168:dbl, "SuperHeat"=w167:dbl, "Cascade Extra.High Side RPM"=w177:dbl, "Cascade Extra.Low Side RPM"=w179:dbl)
            n62 = Round To Nearest(number=w179) -> (nearest integer value=→"Low Side RPM":dbl)
            n63 = Round To Nearest(number=w177) -> (nearest integer value=→"High Side RPM":dbl)
            n64 = local read "Graph Temp Unit"() -> (w164:bool)
            n65 = case shown="True" w164 {
              tunnel: w168 -> [w182 w188]
              tunnel: w167 -> [w181 w187]
              tunnel: [w182 w184] -> w166
              tunnel: [w181 w183] -> w165
              frame False {
              }
              frame True {
                n66 = Build Array(w188, w187) -> (w186:dbl[])
                n67 = for {
                  tunnel: w186 -> [w190] mode=indexing
                  tunnel: [w189] -> w185 mode=indexing
                  n68 = expression code="5/9*(x-32)"(w190) -> (w189:dbl)
                }
                n69 = Index Array(array=w185) -> (element #1=w184:dbl, element #2=w183:dbl)  [unwired: 2 in]
              }
            }
            n70 = Bundle By Name(cluster=T13 {"Condensing Pressure(psi)"=0.0, "Compression Ratio"=0.0, "Subcool"=0.0, "Superheat"=0.0, "Current(A)"=0.0, "Suction Pressure(psi)"=0.0} ("Gauges"), "Compression Ratio"=w173, "Current(A)"=w172, "Condensing Pressure(psi)"=w171, "Suction Pressure(psi)"=w170, "Subcool"=w166, "Superheat"=w165) -> (→"Gauges":T13)
          }
          frame #1 {
            # "Update M1 Module Data"
            n71 = Unbundle By Name(w198) -> ("Dataset.System Status.M1 Bin.Bin String"=→"M1 Bin String":string, "Dataset.System Status.M1 Bin.Bin Color"=w199:u16)
            n72 = Unbundle By Name(w198) -> ("Dataset.M1 Status.Evap Temp"=w193:dbl, "Dataset.M1 Status.Feedback"=w194:u8, "Dataset.M1 Status.Case Temp"=w195:dbl, "Dataset.M1 Status.Thermal State"=→"M1 Thermal State":u16, "Dataset.M1 Status.Power Drive"=→"M1 Power Drive Indicator":bool)
            n73 = case shown="0, Default" w199 {
              tunnel: [u32 14342874 u32 16777215 u32 16712704 u32 56399 u32 1185791 u32 2818010 u32 15701504] -> w201
              frame 0, Default {
              }
              frame 1 {
              }
              frame 2 {
              }
              frame 3 {
              }
              frame 4 {
              }
              frame 5 {
              }
              frame 6 {
              }
            }
            n74 = property on="M1 Bin String" class="Str"("Text.BGColor"=w201) -> ()  [unwired: 2 in, 2 out]
            n75 = Equal?(x=w194, y=u8 0) -> (x = y?=w197:bool)
            n76 = Select(t=w193, s=w197, f=w195) -> (s? t:f=→"M1 PV":dbl)
          }
          frame #2 {
            # "Update M2 Module Data"
            n77 = Unbundle By Name(w217) -> ("Dataset.System Status.M2 Bin.Bin String"=→"M2 Bin String":string, "Dataset.System Status.M2 Bin.Bin Color"=w220:u16)
            n78 = Unbundle By Name(w217) -> ("Dataset.M2 Status.Evap Temp"=w212:dbl, "Dataset.M2 Status.Feedback"=w214:u8, "Dataset.M2 Status.Case Temp"=w213:dbl, "Dataset.M2 Status.Thermal State"=→"M2 Thermal State":u16, "Dataset.M2 Status.Power Drive"=→"M2 Power Drive Indicator":bool)
            n79 = case shown="1" w220 {
              tunnel: [u32 14342874 u32 16777215 u32 16712704 u32 56399 u32 1185791 u32 2818010 u32 15701504] -> w219
              frame 0, Default {
              }
              frame 1 {
              }
              frame 2 {
              }
              frame 3 {
              }
              frame 4 {
              }
              frame 5 {
              }
              frame 6 {
              }
            }
            n80 = Equal?(x=w214, y=u8 0) -> (x = y?=w216:bool)
            n81 = Select(t=w212, s=w216, f=w213) -> (s? t:f=→"M2 PV":dbl)
            n82 = property on="M2 Bin String" class="Str"("Text.BGColor"=w219) -> ()  [unwired: 2 in, 2 out]
          }
          frame #3 {
            # "System information For Debugging"
            n83 = Unbundle By Name(w244) -> ("Dataset.M1 Status"=w260:T34)
            n84 = Unbundle By Name(w244) -> ("Dataset.M2 Status"=w257:T35)
            n85 = Unbundle By Name(w244) -> ("Dataset.System Status"=w243:T33)
            n86 = Unbundle By Name(w260) -> ("Head State"=→"M1 Head State":u16, "Thermal State"=→"M1 Thermal Status":u16, "Error"=→"M1 Error":bool, "Heater %"=→"M1 Heater %":dbl)
            n87 = Unbundle By Name(w257) -> ("Head State"=→"M2 Head State":u16, "Thermal State"=→"M2 Thermal Status":u16, "Error"=→"M2 Error":bool, "Heater %"=→"M2 Heater %":dbl)
            n88 = Unbundle By Name(w243) -> ("SOM Status"=w242:T49)
            n89 = Unbundle By Name(w242) -> ("Memory Available"=w241:dbl, "SOM Storage"=w240:dbl, "SD card free space"=w231:dbl, "CPU Usage"=w236:dbl, "Software Version"=w229:string)
            "RT Version" <- w229
            n90 = Unbundle By Name(w243) -> ("M1 Actuated"=→"M1 Actuated":bool, "M2 Actuated"=→"M2 Actuated":bool, "Sleep"=→"Sleep":bool, "Sleep Timer"=→"Sleep Timer":dbl, "Discharge Temp"=→"Comp Temp":dbl, "Compressor Hours"=→"Compressor Hours":dbl, "Serial Number"=→"Serial Number":string)
            n91 = Build Array(w241, w240, w231) -> (w239:dbl[])
            n92 = for {
              tunnel: w239 -> [w262] mode=indexing
              tunnel: [w261] -> w238 mode=indexing
              n93 = Divide(x=w262, y=1000.0) -> (x/y=w261:dbl)
            }
            n94 = Index Array(array=w238) -> (element #1=w237:dbl, element #2=w234:dbl, element #3=w230:dbl)  [unwired: 3 in]
            n95 = Bundle By Name(cluster=T24 {"Software Version"="SW Version:CC 21.5.11.0", "CPU Usage"=46.7905609206245, "Memory Available"=349.908, "SOM Storage(MB)"=241.236, "SD card free space"=31661.0} ("SOM"), "Memory Available"=w237, "SOM Storage(MB)"=w234, "SD card free space"=w230, "CPU Usage"=w236, "Software Version"=w229) -> (→"SOM":T24)
          }
          frame #4 {
            # "Graphs in Control Tab (Fit Y-Scale at Main Waveform Charts )"
            n96 = Unbundle By Name(w272) -> ("Dataset.M1 Status"=w283:T34)
            n97 = Unbundle By Name(w272) -> ("Dataset.M2 Status"=w279:T35)
            n98 = Unbundle By Name(w279) -> ("Set Temp"=w273:dbl, "Evap Temp"=w278:dbl, "Case Temp"=w277:dbl, "TSD"=w276:dbl, "AC Load Watts"=w275:dbl)
            n99 = Unbundle By Name(w283) -> ("Set Temp"=w274:dbl, "Evap Temp"=w282:dbl, "Case Temp"=w280:dbl, "TSD Temp"=w281:dbl, "Intec Feedback"=w264:dbl, "AC Load Watts"=w265:dbl)
            n100 = Build Array(w274, w282, w280, w281, w264, w265) -> (w270:dbl[])
            "M1 Channels" <- w270
            n101 = Build Array(w273, w278, w277, w276, w275) -> (w268:dbl[])
            "M2 Channels" <- w268
            n102 = control-ref of="M1 Main Waveform"() -> (w271:refnum<vi>)
            n103 = control-ref of="M2 Main Waveform"() -> (w269:refnum<vi>)
            n104 = case shown="False" "Y-scale" {
              tunnel: w271 -> [w288 w304]
              tunnel: w270 -> [_ w303]
              tunnel: w269 -> [w285 w302]
              tunnel: w268 -> [_ w301]
              tunnel: [T40."Disabled and Grayed Out" ("Disabled") T40."Enabled" ("Disabled")] -> w266
              frame False {
                # "Y- Autoscale"
                n105 = property on="Property Node" class="WFChart (strict)"(reference=w288, "YScale.ScaleFit"=u8 2 ("Y Scale.Scale Fit")) -> ()  [unwired: 1 in, 2 out]
                n106 = property on="Property Node" class="WFChart (strict)"(reference=w285, "YScale.ScaleFit"=u8 2 ("Y Scale.Scale Fit")) -> ()  [unwired: 1 in, 2 out]
              }
              frame True {
                # "Manually fix the Y-scale"
                n107 = Array Max & Min(array=w303) -> (max value=w297:dbl, min value=w298:dbl)  [unwired: 2 out]
                n108 = Array Max & Min(array=w301) -> (max value=w292:dbl, min value=w293:dbl)  [unwired: 2 out]
                n109 = Add(x=w297, y="Fixed Y-Range") -> (x+y=w299:dbl)
                n110 = Subtract(x=w298, y="Fixed Y-Range") -> (x-y=w300:dbl)
                n111 = Add(x=w292, y="Fixed Y-Range") -> (x+y=w294:dbl)
                n112 = Subtract(x=w293, y="Fixed Y-Range") -> (x-y=w295:dbl)
                n113 = property on="Property Node" class="WFChart (strict)"(reference=w304, "YScale.Maximum"=w299, "YScale.Minimum"=w300, "YScale.ScaleFit"=u8 0 ("Y Scale.Scale Fit")) -> ()  [unwired: 1 in, 2 out]
                n114 = property on="Property Node" class="WFChart (strict)"(reference=w302, "YScale.Maximum"=w294, "YScale.Minimum"=w295, "YScale.ScaleFit"=u8 0 ("Y Scale.Scale Fit")) -> ()  [unwired: 1 in, 2 out]
              }
            }
            n115 = property on="Fixed Y-Range" class="DigNum (strict)"("DisabledEnum"=w266) -> ()  [unwired: 2 in, 2 out]
          }
          frame #5 {
            w308 = T1 {"Set Temp"=0.0, "Read Temp"=23.7890625, "Package"="50", "Force"=0.0, "Feedback"=0} ("M1 Status")
            # "Display the status of M1 and M2 below the main page"
            n116 = Unbundle By Name(w309) -> ("Dataset.M1 Status.Set Temp"=w327:dbl, "Dataset.M1 Status.Package"=w326:string, "Dataset.M1 Status.Piston Force"=w325:dbl, "Dataset.M1 Status.Evap Temp"=w322:dbl, "Dataset.M1 Status.Feedback"=w319:u8, "Dataset.M1 Status.Case Temp"=w321:dbl)
            n117 = Unbundle By Name(w309) -> ("Dataset.M2 Status.Set Temp"=w318:dbl, "Dataset.M2 Status.Package"=w317:string, "Dataset.M2 Status.Piston Force"=w316:dbl, "Dataset.M2 Status.Evap Temp"=w314:dbl, "Dataset.M2 Status.Feedback"=w310:u8, "Dataset.M2 Status.Case Temp"=w312:dbl)
            n118 = Equal?(x=w319, y=u8 0) -> (x = y?=w323:bool)
            n119 = Equal?(x=w310, y=u8 0) -> (x = y?=w313:bool)
            n120 = Unbundle By Name(w309) -> ("Dataset.System Status.Power On Off"=→"Play/Pause" →"Comp":bool)
            n121 = Select(t=w322, s=w323, f=w321) -> (s? t:f=w320:dbl)
            n122 = Select(t=w314, s=w313, f=w312) -> (s? t:f=w311:dbl)
            n123 = Bundle By Name(cluster=w308, "Set Temp"=w327, "Package"=w326, "Force"=w325, "Read Temp"=w320, "Feedback"=w319) -> (→"M1 Data":T1)
            n124 = Bundle By Name(cluster=w308, "Set Temp"=w318, "Package"=w317, "Force"=w316, "Read Temp"=w311, "Feedback"=w310) -> (→"M2 Data":T1)
          }
          frame #6 {
            # "(°F - 32) × 5/9 => °C"
            # "Display module and sytem graphs on Graph tab"
            n125 = Unbundle By Name(w357) -> ("Dataset.M1 Status.AC Load Watts"=w329:dbl, "Dataset.M1 Status.Case Temp"=w353:dbl, "Dataset.M1 Status.Evap Temp"=w352:dbl, "Dataset.M1 Status.Heater %"=w351:dbl, "Dataset.M1 Status.EEV Steps"=w355:u32)
            n126 = Unbundle By Name(w357) -> ("Dataset.M2 Status.AC Load Watts"=w330:dbl, "Dataset.M2 Status.Case Temp"=w349:dbl, "Dataset.M2 Status.Evap Temp"=w348:dbl, "Dataset.M2 Status.Heater %"=w347:dbl, "Dataset.M2 Status.EEV Steps"=w345:u32)
            n127 = To Double Precision Float(number=w355) -> (double precision float=w354:dbl)
            n128 = To Double Precision Float(number=w345) -> (double precision float=w346:dbl)
            n129 = Unbundle By Name(w357) -> ("Dataset.System Status.Bypass Steps"=w339:u16, "Dataset.System Status.Discharge Temp"=w340:dbl, "Dataset.System Status.Liquid Temp"=w341:dbl, "Dataset.System Status.Suction Temp"=w342:dbl, "Dataset.System Status.Ambient Temp"=w343:dbl)
            n130 = Bundle By Name(cluster=T18 {"Case Temp"=0.0, "Evap Temp"=0.0, "Heater Power (%)"=0.0, "EEV Steps"=0.0, "M1 AC Load(W)"=nan} ("M1 Temp Graphs"), "M1 AC Load(W)"=w329, "Case Temp"=w353, "Evap Temp"=w352, "Heater Power (%)"=w351, "EEV Steps"=w354) -> (→"M1 Graphs":T18)
            n131 = Bundle By Name(cluster=T18 {"Case Temp"=0.0, "Evap Temp"=0.0, "Heater Power (%)"=0.0, "EEV Steps"=0.0, "M1 AC Load(W)"=nan} ("M1 Temp Graphs"), "M1 AC Load(W)"=w330, "Case Temp"=w349, "Evap Temp"=w348, "Heater Power (%)"=w347, "EEV Steps"=w346) -> (→"M2 Graphs":T18)
            n132 = local read "Graph Temp Unit"() -> (w331:bool)
            n133 = To Double Precision Float(number=w339) -> (double precision float=w337:dbl)
            n134 = case shown="False" w331 {
              tunnel: w340 -> [w361 w371]
              tunnel: w341 -> [w360 w370]
              tunnel: w342 -> [w359 w369]
              tunnel: w343 -> [w358 w368]
              tunnel: [w361 w365] -> w333
              tunnel: [w360 w364] -> w334
              tunnel: [w359 w363] -> w335
              tunnel: [w358 w362] -> w336
              frame False {
              }
              frame True {
                n135 = Build Array(w371, w370, w369, w368) -> (w367:dbl[])
                n136 = for {
                  tunnel: w367 -> [w378] mode=indexing
                  tunnel: [w372] -> w366 mode=indexing
                  n137 = Subtract(x=w378, y=32.0) -> (x-y=w376:dbl)
                  n138 = Divide(x=5.0, y=9.0) -> (x/y=w373:dbl)
                  n139 = Multiply(x=w376, y=w373) -> (x*y=w372:dbl)
                }
                n140 = Index Array(array=w366) -> (element #1=w365:dbl, element #2=w364:dbl, element #3=w363:dbl, element #4=w362:dbl)  [unwired: 4 in]
              }
            }
            n141 = Bundle By Name(cluster=T11 {"Ambient Temp"=0.0, "Suction Temp"=0.0, "Condensor Temp"=0.0, "Discharge Temp"=0.0, "Bypass Steps"=0.0} ("System Graphs"), "Bypass Steps"=w337, "Discharge Temp"=w333, "Condensor Temp"=w334, "Suction Temp"=w335, "Ambient Temp"=w336) -> (→"System Graphs":T11)
          }
          frame #7 {
            # "Remove the ripple at the M1 main graph"
            n142 = Unbundle By Name(w379) -> ("Dataset.M2 Status"=w398:T35)
            n143 = Unbundle By Name(w379) -> ("Dataset.M1 Status"=w404:T34)
            n144 = Unbundle By Name(w379) -> ("M2 History Temps"=w390:dbl[][])
            n145 = Unbundle By Name(w398) -> ("Evap Temp"=w397:dbl, "Case Temp"=w396:dbl, "TSD"=w395:dbl, "Set Temp"=w388:dbl)
            n146 = Unbundle By Name(w379) -> ("M1 History Temps"=w392:dbl[][])
            n147 = Unbundle By Name(w404) -> ("Evap Temp"=w401:dbl, "Case Temp"=w400:dbl, "TSD Temp"=w399:dbl, "Intec Feedback"=w380:dbl, "Set Temp"=w391:dbl)
            n148 = Build Array(w397, w396, w395) -> (w389:dbl[])
            n149 = Build Array(w401, w400, w399, w380) -> (w393:dbl[])
            n150 = case shown="False" "Average Graph" {
              tunnel: w393 -> [w421 w424]
              tunnel: w392 -> [w413 w425]
              tunnel: w391 -> [w420 w432]
              tunnel: w390 -> [w416 w430]
              tunnel: w389 -> [w417 w433]
              tunnel: w388 -> [w418 w431]
              tunnel: [w415 w429] -> w385
              tunnel: [w414 w428] -> w383
              tunnel: [w413 w423] -> w382
              tunnel: [w416 w427] -> w381
              frame False {
                n151 = Insert Into Array(array=w421, index=0, new element=w420) -> (w414:dbl[])
                n152 = Insert Into Array(array=w417, index=0, new element=w418) -> (w415:dbl[])
              }
              frame True {
                n153 = Build Array (concatenate)(w425, w424) -> (w423:dbl[][])
                n154 = Build Array (concatenate)(w430, w433) -> (w427:dbl[][])
                n155 = Transpose 2D Array(2D array=w423) -> (transposed array=w438:dbl[][])
                n156 = Transpose 2D Array(2D array=w427) -> (transposed array=w434:dbl[][])
                n157 = for {
                  tunnel: w438 -> [w445] mode=indexing
                  tunnel: [w448] -> w437 mode=indexing
                  n158 = Reverse 1D Array(array=w445) -> (reversed array=w444:dbl[])
                  n159 = Array Subset(array=w444, length=30) -> (w446:dbl[])  [unwired: 1 in]
                  n160 = call-poly <vilib>:"Mean.vi"("X"=w446) -> ("mean"=w448:dbl)  [unwired: 1 out]
                }
                n161 = for {
                  tunnel: w434 -> [w440] mode=indexing
                  tunnel: [w441] -> w426 mode=indexing
                  n162 = Reverse 1D Array(array=w440) -> (reversed array=w439:dbl[])
                  n163 = Array Subset(array=w439, length=30) -> (w442:dbl[])  [unwired: 1 in]
                  n164 = call-poly <vilib>:"Mean.vi"("X"=w442) -> ("mean"=w441:dbl)  [unwired: 1 out]
                }
                n165 = Insert Into Array(array=w437, index=0, new element=w432) -> (w428:dbl[])
                n166 = Insert Into Array(array=w426, index=0, new element=w431) -> (w429:dbl[])
              }
            }
            n167 = Get Date/Time In Seconds() -> (seconds since 1Jan1904=w384:timestamp)
            n168 = for {
              tunnel: [w408] -> w386 mode=indexing
              tunnel: w384 -> [w407]
              tunnel: w383 -> [w406] mode=indexing
              n169 = Build Array(w406) -> (w405:dbl[])
              n170 = Bundle By Name("Y"=w405, "t0"=w407) -> (w408:waveform(dbl))  [unwired: 1 in]
            }
            "M1 Main Waveform" <- w386
            n171 = for {
              tunnel: w384 -> [w411]
              tunnel: [w412] -> w387 mode=indexing
              tunnel: w385 -> [w410] mode=indexing
              n172 = Build Array(w410) -> (w409:dbl[])
              n173 = Bundle By Name("t0"=w411, "Y"=w409) -> (w412:waveform(dbl))  [unwired: 1 in]
            }
            "M2 Main Waveform" <- w387
            n174 = Bundle By Name(cluster=w403, "M1 History Temps"=w382, "M2 History Temps"=w381) -> (w402:T27)
          }
          frame #8 {
            # "Update M1 and M2 conmand module when both first call and chaged value"
            n175 = Unbundle By Name(w456) -> ("Dataset.M1 Status"=w463:T34, "Dataset.M1 Status.Head State"=w454:u16)
            n176 = Unbundle By Name(w456) -> ("Dataset.M2 Status"=w462:T35, "Dataset.M2 Status.Head State"=w450:u16)
            n177 = Unbundle By Name(w456) -> ("Network Connection"=w455:bool, "Dataset.Config Data.Packages.DUT Names"=w457:T50)
            n178 = Equal?(x=w450, y=enum16{"Disabled", "Run", "Error"}."Run" ("Dataset.M1 Status.Head State")) -> (x = y?=w449:bool)
            n179 = Equal?(x=w454, y=enum16{"Disabled", "Run", "Error"}."Run" ("Dataset.M1 Status.Head State")) -> (x = y?=w452:bool)
            n180 = Unbundle By Name(w462) -> ("Package"=w458:string, "Set Temp"=w459:dbl)
            n181 = Unbundle By Name(w463) -> ("Set Temp"=w461:dbl, "Package"=w460:string)
            n182 = case shown="True" w455 {
              tunnel: w461 -> [_ w471]
              tunnel: w460 -> [_ w473]
              tunnel: w459 -> [_ w468]
              tunnel: w458 -> [_ w474]
              tunnel: w457 -> [_ w475]
              tunnel: w449 -> [_ w464]
              tunnel: w452 -> [_ w465]
              frame False {
              }
              frame True {
                n183 = property on="M2 Enable" class="Bool (strict)"("Value"=w464) -> ()  [unwired: 2 in, 2 out]
                n184 = property on="M1 Enable" class="Bool (strict)"("Value"=w465) -> ()  [unwired: 2 in, 2 out]
                n185 = Cluster To Array(cluster=w475) -> (array=w472:string[])
                n186 = Search 1D Array(1D array=w472, element=w474) -> (index of element=w467:i32)  [unwired: 1 in]
                n187 = Search 1D Array(1D array=w472, element=w473) -> (index of element=w470:i32)  [unwired: 1 in]
                n188 = To Unsigned Word Integer(number=w467) -> (unsigned 16bit integer=w466:u16)
                n189 = To Unsigned Word Integer(number=w470) -> (unsigned 16bit integer=w469:u16)
                n190 = local write "M1 Set Temp"(w471) -> ()
                n191 = local write "M1 Package"(w469) -> ()
                n192 = local write "M2 Package"(w466) -> ()
                n193 = local write "M2 Set Temp"(w468) -> ()
              }
            }
          }
          frame #9 {
            # "ETC"
            n194 = property on="Heater Power (%)" class="WFChart (strict)"() -> ("YScale.ScaleFit"=w483:u8)  [unwired: 2 in, 2 out]
            n195 = Unbundle By Name(w488) -> ("Dataset.Config Data.Set Point Range"=w492:cluster{"Max":dbl, "Min":dbl}, "Dataset.Config Data.Packages.DUT Names"=w485:T50)
            n196 = Equal To 0?(x=w483) -> (x = 0?=w482:bool)
            n197 = case shown="True" w482 {
              frame False {
              }
              frame True {
                n198 = property on="Heater Power (%)" class="WFChart (strict)"("YScale.Maximum"=100.0 ("Y Scale.Range:Maximum"), "YScale.Minimum"=0.0 ("Y Scale.Range:Minimum")) -> ()  [unwired: 2 in, 2 out]
              }
            }
            n199 = property on="EEV Steps" class="WFChart (strict)"() -> ("YScale.ScaleFit"=w481:u8)  [unwired: 2 in, 2 out]
            n200 = control-ref of="M1 Set Temp"() -> (w489:refnum<vi>)
            n201 = control-ref of="M2 Set Temp"() -> (w490:refnum<vi>)
            n202 = control-ref of="M1 Package"() -> (w487:refnum<vi>)
            n203 = control-ref of="M2 Package"() -> (w486:refnum<vi>)
            n204 = Build Array(w487, w486) -> (w484:refnum<vi>[])
            n205 = Build Array(w489, w490) -> (w491:refnum<vi>[])
            n206 = Equal To 0?(x=w481) -> (x = 0?=w480:bool)
            n207 = for {
              tunnel: w491 -> [w505] mode=indexing
              tunnel: w492 -> [w504]
              tunnel: w485 -> [w502]
              tunnel: w484 -> [w503] mode=indexing
              n208 = Unbundle By Name(w504) -> ("Max"=w506:dbl, "Min"=w507:dbl)
              n209 = Cluster To Array(cluster=w502) -> (array=w501:string[])
              n210 = property class="DigNum (strict)"(reference=w505, "Maximum"=w506, "Minimum"=w507) -> ()  [unwired: 1 in, 2 out]
              n211 = property class="Ring (strict)"(reference=w503, "Strings []"=w501) -> ()  [unwired: 1 in, 2 out]
            }
            n212 = case shown="True" w480 {
              frame False {
              }
              frame True {
                n213 = property on="EEV Steps" class="WFChart (strict)"("YScale.Maximum"=600.0 ("Y Scale.Range:Maximum"), "YScale.Minimum"=0.0 ("Y Scale.Range:Minimum")) -> ()  [unwired: 2 in, 2 out]
              }
            }
            n214 = property on="Heater Power (%)" class="WFChart (strict)"() -> ("YScale.ScaleFit"=w479:u8)  [unwired: 2 in, 2 out]
            n215 = property on="EEV Steps" class="WFChart (strict)"() -> ("YScale.ScaleFit"=w477:u8)  [unwired: 2 in, 2 out]
            n216 = Equal To 0?(x=w479) -> (x = 0?=w478:bool)
            n217 = case shown="True" w478 {
              frame False {
              }
              frame True {
                n218 = property on="Heater Power (%)" class="WFChart (strict)"("YScale.Maximum"=100.0 ("Y Scale.Range:Maximum"), "YScale.Minimum"=0.0 ("Y Scale.Range:Minimum")) -> ()  [unwired: 2 in, 2 out]
              }
            }
            n219 = Equal To 0?(x=w477) -> (x = 0?=w476:bool)
            n220 = case shown="True" w476 {
              frame False {
              }
              frame True {
                n221 = property on="EEV Steps" class="WFChart (strict)"("YScale.Maximum"=600.0 ("Y Scale.Range:Maximum"), "YScale.Minimum"=0.0 ("Y Scale.Range:Minimum")) -> ()  [unwired: 2 in, 2 out]
              }
            }
          }
        }
      }
      frame "UI:Enable Tabs" {
        n222 = Variant To Data(error in=w517, type=i32[] [] ("Page array"), Variant=w516) -> (data=w508:i32[], error out=w510:errorcluster)
        n223 = control-ref of="Tab Control"() -> (w518:refnum<vi>)
        n224 = property class="TabCtl (strict)"(reference=w518) -> ("Pages"=w515:refnum<vi>[])  [unwired: 1 in, 2 out]
        n225 = Array Size(array=w508) -> (size(s)=w514:i32)
        n226 = Split 1D Array(array=w515, index=w514) -> (first subarray=w513:refnum<vi>[], second subarray=w512:refnum<vi>[])
        n227 = for {
          tunnel: w513 -> [w523] mode=indexing
          tunnel: T41."Page Enabled" ("Page Enabled State") -> [w524]
          n228 = property class="Page"(reference=w523, "PageEnb"=w524) -> ()  [unwired: 1 in, 2 out]
        }
        n229 = for {
          tunnel: w512 -> [w521] mode=indexing
          tunnel: T41."Page Disabled & Grayed" ("Page Enabled State") -> [w522]
          n230 = property class="Page"(reference=w521, "PageEnb"=w522) -> ()  [unwired: 1 in, 2 out]
        }
      }
      frame "UI:Enable Controls" {
        n231 = control-ref of="?"() -> (w535:refnum<vi>)
        n232 = control-ref of="?"() -> (w529:refnum<vi>)
        n233 = control-ref of="?"() -> (w528:refnum<vi>)
        n234 = control-ref of="?"() -> (w527:refnum<vi>)
        n235 = control-ref of="?"() -> (w526:refnum<vi>)
        n236 = control-ref of="?"() -> (w525:refnum<vi>)
        n237 = Variant To Data(error in=w546, type=FALSE ("Visible"), Variant=w545) -> (data=w536:bool, error out=w542:errorcluster)
        n238 = Build Array(w535, w529, w528, w527, w526, w525) -> (w543:refnum<vi>[])
        n239 = property on="Configure" class="Bool"(error in=w542, "Visible"=w536) -> (error out=w539:errorcluster)  [unwired: 1 in, 1 out]
        n240 = for {
          tunnel: w536 -> [w549]
          tunnel: w543 -> [w548] mode=indexing
          n241 = property class="DigNum (strict)"(reference=w548, "Visible"=w549) -> ()  [unwired: 1 in, 2 out]
        }
        n242 = property on="Subcool" class="Knob (strict)"(error in=w539, "Visible"=w536) -> (error out=w538:errorcluster)  [unwired: 1 in, 1 out]
        n243 = property on="Superheat" class="Knob (strict)"(error in=w538, "Visible"=w536) -> (error out=w537:errorcluster)  [unwired: 1 in, 1 out]
        n244 = Select(t=T40."Enabled" ("Disabled"), s=w536, f=T40."Disabled") -> (s? t:f=w530:T40)
        n245 = property on="M1 EEV Manual" class="DigNum (strict)"(error in=w537, "DisabledEnum"=w530) -> (error out=w534:errorcluster)  [unwired: 1 in, 1 out]
        n246 = property on="M1 Heater output" class="DigNum (strict)"(error in=w534, "DisabledEnum"=w530) -> (error out=w533:errorcluster)  [unwired: 1 in, 1 out]
        n247 = property on="M2 EEV Manual" class="DigNum (strict)"(error in=w533, "DisabledEnum"=w530) -> (error out=w532:errorcluster)  [unwired: 1 in, 1 out]
        n248 = property on="M2 Heater Output" class="DigNum (strict)"(error in=w532, "DisabledEnum"=w530) -> (error out=w531:errorcluster)  [unwired: 1 in, 1 out]
      }
      frame "UI:Visible Controls" {
        n249 = stacked-sequence {
          tunnel: [w553 _] -> w550
          tunnel: w551 -> [w558 w565]
          tunnel: w552 -> [w560 w566]
          frame #0 {
            # "Module#2 Page makes disable"
            n250 = Unbundle By Name(w558) -> ("M2 Bootup"=w557:bool)
            n251 = Select(t=T41."Page Enabled" ("Page Enabled State"), s=w557, f=T41."Page Disabled & Grayed" ("Page Enabled State")) -> (s? t:f=w554:T41)
            n252 = control-ref of="Graph Tab CTL"() -> (w562:refnum<vi>)
            n253 = property class="TabCtl (strict)"(reference=w562, error in=w560) -> (error out=w559:errorcluster, "Pages"=w563:refnum<vi>[])  [unwired: 1 out]
            n254 = Index Array(array=w563, index=1) -> (element=w564:refnum<vi>)
            n255 = property class="Page"(reference=w564, error in=w559, "PageEnb"=w554) -> (error out=w553:errorcluster)  [unwired: 1 out]
          }
          frame #1 {
            # "Visibility of Tab Control"
            n256 = control-ref of="Tab Control"() -> (w567:refnum<vi>)
            n257 = Unbundle By Name(w565) -> ("System Ready"=w570:bool, "M2 Bootup"=w571:bool)
            n258 = property class="TabCtl (strict)"(reference=w567, error in=w566) -> (error out=w569:errorcluster, "Pages"=w568:refnum<vi>[])  [unwired: 1 out]
            n259 = for {
              tunnel: w568 -> [w578] mode=indexing
              tunnel: w569 -> [w576]
              tunnel: w571 -> [w574]
              tunnel: w570 -> [w573]
              tunnel: [w572] -> _
              n260 = property class="Page"(reference=w578, error in=w576) -> (error out=w575:errorcluster, "ControlsOnPage"=w577:refnum<vi>[])  [unwired: 1 out]
              n261 = for {
                tunnel: w577 -> [w589] mode=indexing
                tunnel: w575 -> [w588]
                tunnel: w574 -> [w587]
                tunnel: w573 -> [w586]
                tunnel: [w585] -> w572
                n262 = property class="Ctl"(reference=w589, error in=w588) -> (reference out=w583:refnum<vi>, error out=w582:errorcluster, "Label.Text"=w580:string)
                n263 = Scan From String(format string="%s", input string=w580) -> (output 1=w581:string)  [unwired: 3 in, 3 out]
                n264 = case shown="Default" w581 {
                  tunnel: w586 -> [w590 _]
                  tunnel: w587 -> [_ w591]
                  tunnel: [w590 w591] -> w579
                  frame Default {
                  }
                  frame "M2" {
                  }
                }
                n265 = property class="Ctl"(reference=w583, error in=w582, "Visible"=w579) -> (error out=w585:errorcluster)  [unwired: 1 out]
              }
            }
          }
        }
      }
      frame "UI:Refresh Graph" {
        w600 = 0.0 ("M1 Heater output")
        w601 = u16 0 ("M1 EEV Manual")
        w604 = dbl[][] [] ("M1 Original Temps")
        w612 = waveform(dbl)[][] [] ("M1 Main Waveform")
        n266 = Variant To Data(error in=w622, type="", Variant=w621) -> (data=w594:string, error out=w607:errorcluster)
        n267 = control-ref of="Ambient Temp"() -> (w614:refnum<vi>)
        n268 = Format Into String(format string="(%s)", initial string="Superheat" ("Command"), w594) -> (resulting string=w592:string)  [unwired: 1 in, 1 out]
        n269 = Format Into String(format string="(%s)", initial string="Subcool" ("Command"), w594) -> (resulting string=w593:string)  [unwired: 1 in, 1 out]
        n270 = Format Into String(format string="(%s)", initial string="Temperature" ("Command"), w594) -> (resulting string=w615:string)  [unwired: 1 in, 1 out]
        n271 = property on="Subcool" class="Knob (strict)"("Caption.Text"=w593) -> ()  [unwired: 2 in, 2 out]
        n272 = property on="Superheat" class="Knob (strict)"("Caption.Text"=w592) -> ()  [unwired: 2 in, 2 out]
        n273 = control-ref of="System Graphs"() -> (w608:refnum<vi>)
        n274 = control-ref of="M1 Graphs"() -> (w611:refnum<vi>)
        n275 = control-ref of="M2 Graphs"() -> (w610:refnum<vi>)
        n276 = property class="WFChart (strict)"(reference=w614, "YScale.NameLbl.Text"=w615) -> ()  [unwired: 1 in, 2 out]
        n277 = Build Array(w611, w610, w608) -> (w609:refnum<vi>[])
        n278 = property on="M1 Humidity" class="WFChart (strict)"(error in=w607, "History Data"=cluster{"M1 RH":dbl, "RH Threshold":dbl}[] []) -> (error out=w606:errorcluster)  [unwired: 1 in, 1 out]
        n279 = for {
          tunnel: w609 -> [w626] mode=indexing
          n280 = property class="Clust (strict)"(reference=w626) -> ("Controls[]"=w624:refnum<vi>[])  [unwired: 1 in, 2 out]
          n281 = for {
            tunnel: dbl[] [] ("History Data") -> [w630]
            tunnel: w624 -> [w629] mode=indexing
            tunnel: refnum<vi> refnum ("M1 Heater Power (%)") -> [w627]
            n282 = To More Specific Class(target class=w627, reference=w629) -> (specific class reference=w628:refnum<vi>)  [unwired: 1 in, 1 out]
            n283 = property class="WFChart (strict)"(reference=w628, "History Data"=w630) -> ()  [unwired: 1 in, 2 out]
          }
        }
        n284 = property on="M2 Main Waveform" class="WFChart (strict)"(error in=w606, "History Data"=w612) -> (error out=w613:errorcluster)  [unwired: 1 in, 1 out]
        n285 = property on="M1 Main Waveform" class="WFChart (strict)"(error in=w613, "History Data"=w612) -> (error out=w599:errorcluster)  [unwired: 1 in, 1 out]
        n286 = property on="M1 EEV Manual" class="DigNum (strict)"("Value"=w601) -> ()  [unwired: 2 in, 2 out]
        n287 = property on="M2 EEV Manual" class="DigNum (strict)"("Value"=w601) -> ()  [unwired: 2 in, 2 out]
        n288 = property on="M1 Heater output" class="DigNum (strict)"("Value"=w600) -> ()  [unwired: 2 in, 2 out]
        n289 = property on="M2 Heater Output" class="DigNum (strict)"("Value"=w600) -> ()  [unwired: 2 in, 2 out]
        n290 = property on="Manual Bypass Mode" class="Arr (strict)"(error in=w599, "Value"=bool[] [] ("Manual Bypass Mode")) -> (error out=w602:errorcluster)  [unwired: 1 in, 1 out]
        n291 = Bundle By Name(cluster=w619, "M1 History Temps"=w604, "M2 History Temps"=w604) -> (w620:T27)
      }
      frame "UI:Arrange Controls" {
        # "Resize the main Graph"
        n292 = Unbundle By Name(w647) -> ("M2 Bootup"=w632:bool)
        n293 = property on="M1 Enable" class="Bool (strict)"(error in=w631, "Visible"=w632) -> (error out=w633:errorcluster)  [unwired: 1 in, 1 out]
        n294 = Select(t=u32 4 ("Number of Rows"), s=w632, f=u32 2 ("Number of Rows")) -> (s? t:f=w637:u32)
        n295 = property on="M2 Data" class="Clust (strict)"(error in=w633, "Visible"=w632) -> (error out=w640:errorcluster)  [unwired: 1 in, 1 out]
        n296 = property on="Manual Bypass Mode" class="Arr (strict)"("Number of Rows"=w637) -> ()  [unwired: 2 in, 2 out]
        n297 = Select(t=u32 239 ("Plot Area:Size:Height"), s=w632, f=u32 530 ("Plot Area:Size:Height")) -> (s? t:f=w653:u32)
        n298 = property on="M1 Main Waveform" class="WFChart (strict)"(error in=w640, "Height"=w653) -> (error out=w634:errorcluster)  [unwired: 1 in, 1 out]
        n299 = case shown="False" w632 {
          tunnel: [T42 {"Left"=2900, "Top"=-20} ("Position") T42 {"Left"=1930, "Top"=40} ("Position")] -> w651
          tunnel: [T42 {"Left"=2880, "Top"=-43} ("Position") T42 {"Left"=1905, "Top"=20} ("Position")] -> w650
          frame False {
          }
          frame True {
          }
        }
        n300 = property on="Power On-Off" class="Bool (strict)"("Position"=w651) -> ()  [unwired: 2 in, 2 out]
        n301 = property on="Play/Pause" class="Bool"("Position"=w650) -> ()  [unwired: 2 in, 2 out]
        n302 = property on="Event Tab" class="TabCtl (strict)"(error in=w634, "Value"=enum32{"Cobra Events", "GUI Events"}."Cobra Events" ("Event Tab")) -> (error out=w642:errorcluster)  [unwired: 1 in, 1 out]
        n303 = case shown="False" w632 {
          tunnel: [w658 w660] -> w643
          tunnel: [T42 {"Left"=1915, "Top"=190} ("Position") T42 {"Left"=2890, "Top"=-70} ("Position")] -> w652
          tunnel: [w658 w660] -> w636
          frame False {
            w658 = T42 {"Left"=1880, "Top"=150} ("Position")
          }
          frame True {
            w660 = T42 {"Left"=2850, "Top"=-110} ("Position")
          }
        }
        n304 = property on="Tab Control" class="TabCtl (strict)"(error in=w642, "Value"=T6."Controls" ("Tab Control")) -> (error out=w645:errorcluster)  [unwired: 1 in, 1 out]
        n305 = property on="M1 Power Drive Control" class="Bool (strict)"("Position"=w652) -> ()  [unwired: 2 in, 2 out]
        n306 = property on="M1 Power Drive Indicator" class="Bool"("Position"=w643) -> ()  [unwired: 2 in, 2 out]
        n307 = property on="M1 Safe Temp and Head State" class="Bool (strict)"("Position"=w636) -> ()  [unwired: 2 in, 2 out]
        n308 = property on="Graph Tab CTL" class="TabCtl (strict)"(error in=w645, "Value"=enum32{"Head #1", "Head #2"}."Head #1" ("Graph Tab CTL")) -> (error out=w644:errorcluster)  [unwired: 1 in, 1 out]
      }
      frame "UI:Update Network Down Data" {
        # "Keep RT status if not change"
        n309 = Unbundle By Name(w662) -> ("Dataset"=w672:T32)
        n310 = Unbundle By Name(w662) -> ("Dataset.Config Data.Packages.DUT Names"=w675:T50)
        n311 = Unbundle By Name(w672) -> ("System Status.Power On Off"=w670:bool, "Config Data"=w671:T36, "System Status.M1 Actuated"=w665:bool, "M1 Status"=w666:T34)
        n312 = Unbundle By Name(w666) -> ("Set Temp"=w669:dbl, "Power Drive"=w668:bool, "Feedback"=w667:u8, "Package"=w676:string)
        n313 = Cluster To Array(cluster=w675) -> (array=w674:string[])
        n314 = Search 1D Array(1D array=w674, element=w676) -> (index of element=w677:i32)  [unwired: 1 in]
        n315 = Bundle By Name(cluster=T43 {"Set Temp"=0.0, "Power Drive"=FALSE, "Feedback"=0, "Package"=0, "Enable"=FALSE} ("Network Data Down.M1 Commands"), "Enable"=w665, "Set Temp"=w669, "Power Drive"=w668, "Feedback"=w667, "Package"=w677) -> (w664:T43)
        n316 = Bundle By Name(cluster=w662, "Network Data Down.System Power On Off"=w670, "Network Data Down.Config Data"=w671, "Network Data Down.M1 Commands"=w664) -> (w663:T27)
      }
      frame "UI:Module Enable" {
        n317 = Unbundle By Name(w684) -> ("Dataset.M2 Status.Case Temp"=w686:dbl, "Dataset.M2 Status.Evap Temp"=w687:dbl)
        n318 = Unbundle By Name(w684) -> ("Dataset.M1 Status.Case Temp"=w693:dbl, "Dataset.M1 Status.Evap Temp"=w692:dbl)
        n319 = Unbundle By Name(w684) -> ("Network Connection"=w701:bool)
        n320 = Not Equal To 0?(x=w686) -> (x != 0?=w688:bool)
        n321 = Not Equal To 0?(x=w693) -> (x != 0?=w691:bool)
        n322 = Not Equal To 0?(x=w687) -> (x != 0?=w689:bool)
        n323 = Not Equal To 0?(x=w692) -> (x != 0?=w690:bool)
        n324 = Compound Arithmetic op=AND(w688, w689) -> (w681:bool)
        n325 = Compound Arithmetic op=AND(w691, w690) -> (w679:bool)
        n326 = Select(t="NS:Read\nUI:Reinitialize Front Panel\nUI:Module Enable" ("Command"), s=w701, f="NS:Open Connection" ("Command")) -> (s? t:f=w694:string)
        n327 = Select(t="MACRO:Display Panel" ("Command"), s=w679, f=w694) -> (s? t:f=w702:string)
        n328 = call "Messaging EnQ Multiline String.vi"("Command(s)"=w702, "error in (no error)"=w683) -> ("error out"=w703:errorcluster)  [unwired: 9 in]
        n329 = Select(t=T40."Enabled" ("Disabled"), s=w679, f=T40."Disabled" ("Disabled")) -> (s? t:f=w698:T40)
        n330 = Not(x=w679) -> (.not. x?=w697:bool)
        n331 = property on="System Ready" class="Bool (strict)"(error in=w703, "Blinking"=w697, "Value"=w679, "DisabledEnum"=w698) -> (error out=w682:errorcluster)  [unwired: 1 in, 1 out]
        n332 = Bundle By Name(cluster=w684, "M2 Bootup"=w681, "System Ready"=w679) -> (w704:T27)
      }
      frame "UI:Reinitialize Front Panel" {
        # "Time delay on display"
        # "Visible or Invisible Components in Front Panel"
        n333 = Unbundle By Name(w708) -> ("System Ready"=w705:bool, "M2 Bootup"=w714:bool, "Core.Current VI"=w713:refnum<vi>)
        n334 = property class="VI"(reference=w713, error in=w707) -> (error out=w709:errorcluster, "Panel"=w712:refnum<vi>)  [unwired: 1 out]
        n335 = property class="Pnl"(reference=w712, error in=w709) -> (error out=w710:errorcluster, "Controls[]"=w711:refnum<vi>[])  [unwired: 1 out]
        n336 = for {
          tunnel: w711 -> [w728] mode=indexing
          tunnel: w710 -> [w729]
          tunnel: w705 -> [w725]
          tunnel: w714 -> [w724]
          tunnel: [w721] -> w706
          n337 = property class="Ctl"(reference=w728, error in=w729) -> (reference out=w726:refnum<vi>, error out=w727:errorcluster, "Label.Text"=w723:string)
          n338 = case shown="Default" w723 {
            selector: w723 -> [_ w735]
            tunnel: [w730 w738] -> w722
            tunnel: w727 -> [w730 w738]
            tunnel: w726 -> [w731 w733]
            tunnel: w725 -> [_ w737]
            tunnel: w724 -> [_ w736]
            tunnel: [TRUE ("Network Connection") w734] -> w720
            tunnel: [w731 w733] -> w719
            frame "Net Cluster" {
            }
            frame Default {
              n339 = Scan From String(format string="%s", input string=w735) -> (output 1=w740:string)  [unwired: 3 in, 3 out]
              n340 = case shown="Default" w740 {
                tunnel: [w741 w742] -> w734
                tunnel: w737 -> [w741 _]
                tunnel: w736 -> [_ w742]
                frame Default {
                }
                frame "M2" {
                }
              }
            }
          }
          n341 = property class="Ctl"(reference=w719, error in=w722, "Visible"=w720) -> (error out=w721:errorcluster)  [unwired: 1 out]
        }
        n342 = Not(x=w705) -> (.not. x?=w718:bool)
        n343 = property on="System Ready" class="Bool (strict)"(error in=w706, "Blinking"=w718, "Value"=w705) -> (error out=w715:errorcluster)  [unwired: 1 in, 1 out]
        n344 = flat-sequence {
          tunnel: u32 500 ("milliseconds to wait") -> [w744]
          tunnel: w715 -> [w743]
          tunnel: [w743] -> w716
          frame #0 {
            n345 = Wait (ms)(milliseconds to wait=w744) -> ()  [unwired: 1 out]
          }
        }
      }
      frame "UI:Visibility" {
        n346 = stacked-sequence {
          tunnel: w746 -> [w766 w782 w799]
          frame #0 {
            n347 = Unbundle By Name(w766) -> ("Dataset.System Status.Compressor Amps"=w767:dbl, "Dataset.System Status.Power On Off"=w762:bool, "Dataset.Config Data.System Settings.Cascade"=w768:bool)
            n348 = Unbundle By Name(w766) -> ("System Ready"=w755:bool, "M2 Bootup"=w749:bool)
            n349 = local read "M2 Channels"() -> (w753:dbl[])
            n350 = Index Array(array=w753, index=3) -> (element=w751:dbl)
            n351 = local read "M1 Channels"() -> (w760:dbl[])
            n352 = Not A Number/Path/Refnum?(number/path/refnum=w751) -> (NaN/Path/Refnum?=w752:bool)
            n353 = Not(x=w752) -> (.not. x?=w754:bool)
            n354 = Round To Nearest(number=w767) -> (nearest integer value=w769:dbl)
            n355 = And(x=w749, y=w754) -> (x .and. y?=w747:bool)
            n356 = Not Equal To 0?(x=w769) -> (x != 0?=w765:bool)
            n357 = property on="M2 TSD Feedback" class="Bool (strict)"("Visible"=w747) -> ()  [unwired: 2 in, 2 out]
            n358 = Index Array(array=w760, index=3) -> (element=w759:dbl)
            n359 = Not A Number/Path/Refnum?(number/path/refnum=w759) -> (NaN/Path/Refnum?=w758:bool)
            n360 = Not(x=w758) -> (.not. x?=w757:bool)
            n361 = And(x=w757, y=w755) -> (x .and. y?=w748:bool)
            n362 = And(x=w762, y=w768) -> (x .and. y?=w761:bool)
            n363 = property on="M1 TSD Feedback" class="Bool (strict)"("Visible"=w748) -> ()  [unwired: 2 in, 2 out]
            n364 = property on="High Side RPM" class="DigNum (strict)"("Visible"=w761) -> ()  [unwired: 2 in, 2 out]
            n365 = property on="Low Side RPM" class="DigNum (strict)"("Visible"=w761) -> ()  [unwired: 2 in, 2 out]
            n366 = property on="Cascade Compressor controls" class="Clust (strict)"("Visible"=w761) -> ()  [unwired: 2 in, 2 out]
            n367 = Compound Arithmetic op=AND(w749, w765, w762) -> (w763:bool)
            n368 = Compound Arithmetic op=AND(w755, w765, w762) -> (w764:bool)
            n369 = property on="M1 Thermal State" class="Enum (strict)"("Visible"=w764) -> ()  [unwired: 2 in, 2 out]
            n370 = property on="M2 Thermal State" class="Enum (strict)"("Visible"=w763) -> ()  [unwired: 2 in, 2 out]
          }
          frame #1 {
            n371 = Unbundle By Name(w782) -> ("System Ready"=w774:bool, "M2 Bootup"=w775:bool)
            n372 = local read "M1 Channels"() -> (w773:dbl[])
            n373 = local read "M2 Channels"() -> (w772:dbl[])
            n374 = Index Array(array=w773, index=4) -> (element=w776:dbl)
            n375 = Index Array(array=w772, index=4) -> (element=w780:dbl)
            n376 = Not A Number/Path/Refnum?(number/path/refnum=w776) -> (NaN/Path/Refnum?=w778:bool)
            n377 = Not A Number/Path/Refnum?(number/path/refnum=w780) -> (NaN/Path/Refnum?=w781:bool)
            n378 = And(x=w775, y=w781) -> (x .and. y?=w770:bool)
            n379 = And(x=w778, y=w774) -> (x .and. y?=w771:bool)
            n380 = case shown="True" w770 {
              frame False {
              }
              frame True {
                w783 = u32 4 ("Number of Rows")
                n381 = property on="M2 Channels" class="Arr (strict)"("Number of Rows"=w783) -> ()  [unwired: 2 in, 2 out]
                n382 = property on="M2 Main Waveform" class="WFChart (strict)"("Active Plot"=w783, "LegNumRows"=w783) -> ()  [unwired: 2 in, 2 out]
              }
            }
            n383 = case shown="True" w771 {
              frame False {
              }
              frame True {
                w784 = u32 4 ("Number of Rows")
                n384 = property on="M1 Channels" class="Arr (strict)"("Number of Rows"=w784) -> ()  [unwired: 2 in, 2 out]
                n385 = property on="M1 Main Waveform" class="WFChart (strict)"("Active Plot"=w784, "LegNumRows"=w784) -> ()  [unwired: 2 in, 2 out]
              }
            }
          }
          frame #2 {
            # "Disable"
            # "Disable"
            n386 = Unbundle By Name(w799) -> ("Dataset.M2 Status.Head State"=w789:u16, "Dataset.Config Data.Piston Settings.Diameter (mm)"=w803:dbl, "Dataset.M2 Status.Safe Temp"=w796:bool, "Dataset.Config Data.Safe Temps.Enabled"=w793:bool, "M2 Bootup"=w792:bool)
            n387 = Unbundle By Name(w799) -> ("System Ready"=w791:bool, "Dataset.Config Data.Safe Temps.Enabled"=w797:bool, "Dataset.M1 Status.Safe Temp"=w798:bool, "Dataset.Config Data.Piston Settings.Diameter (mm)"=w804:dbl, "Dataset.M1 Status.Head State"=w786:u16)
            n388 = Greater Than 0?(x=w803) -> (x > 0?=w802:bool)
            n389 = Equal To 0?(x=w789) -> (x = 0?=w788:bool)
            n390 = Greater Than 0?(x=w804) -> (x > 0?=w805:bool)
            n391 = Equal To 0?(x=w786) -> (x = 0?=w785:bool)
            n392 = Compound Arithmetic op=AND(w796, w793, w792) -> (w790:bool)
            n393 = Compound Arithmetic op=AND(w791, w797, w798) -> (w787:bool)
            n394 = property on="M2 Safe Temp and Head State" class="Bool (strict)"("Value"=w788, "Visible"=w790) -> ()  [unwired: 2 in, 2 out]
            n395 = Not(x=w787) -> (.not. x?=w801:bool)
            n396 = Not(x=w790) -> (.not. x?=w800:bool)
            n397 = property on="M1 Safe Temp and Head State" class="Bool (strict)"("Visible"=w787, "Value"=w785) -> ()  [unwired: 2 in, 2 out]
            n398 = Compound Arithmetic op=AND(w802, w800, w792) -> (w794:bool)
            n399 = Compound Arithmetic op=AND(w791, w801, w805) -> (w795:bool)
            n400 = property on="M2 Power Drive Indicator" class="Bool"("Visible"=w794) -> ()  [unwired: 2 in, 2 out]
            n401 = property on="M2 Power Drive Control" class="Bool (strict)"("Visible"=w794) -> ()  [unwired: 2 in, 2 out]
            n402 = property on="M1 Power Drive Control" class="Bool (strict)"("Visible"=w795) -> ()  [unwired: 2 in, 2 out]
            n403 = property on="M1 Power Drive Indicator" class="Bool"("Visible"=w795) -> ()  [unwired: 2 in, 2 out]
          }
        }
      }
      frame "-----MACRO-----" {
        # "MACRO is used for groups of cases that need to be run together."
      }
      frame "MACRO:Initialize" {
        # "1. Initialize Core Data\n2. Set Front Panel State\n3. Detect the available systems"
        # "3."
        # "2."
        # "1."
        # "Send initialize sequence of commands"
        n404 = Variant To Data(error in=w826, type=TRUE ("Log Events?"), Variant=w824) -> (data=w822:bool, error out=w825:errorcluster)
        n405 = call "Messaging EnQ Single.vi"("Command"="SYS:Initialize", "error in (no error)"=w825) -> ("error out"=w818:errorcluster)  [unwired: 9 in]
        n406 = Select(t="Open", s=w822, f="Close") -> (s? t:f=w819:string)
        n407 = Format Into String(format string="UI:Front Panel State>>%s" ("Command"), w819) -> (resulting string=w827:string)  [unwired: 2 in, 1 out]
        n408 = call "Messaging EnQ Single.vi"("Command"=w827, "error in (no error)"=w818) -> ("error out"=w816:errorcluster)  [unwired: 9 in]
        n409 = call "Messaging EnQ Single.vi"("Command"="UI:Reinitialize Front Panel", "error in (no error)"=w816) -> ("error out"=w815:errorcluster)  [unwired: 9 in]
        n410 = call "Messaging EnQ Single.vi"("Command"="NS:Detect Systems", "error in (no error)"=w815) -> ("error out"=w810:errorcluster)  [unwired: 9 in]
        n411 = To Variant(anything=i32[] [0, 1, 2] ("Page array")) -> (Variant=w813:variant)
        n412 = call "Messaging EnQ Single.vi"("Command"="UI:Enable Tabs", "Data"=w813, "error in (no error)"=w810) -> ("error out"=w809:errorcluster)  [unwired: 8 in]
      }
      frame "MACRO:NS Update" {
        n413 = call "Messaging EnQ Single.vi"("Command"="NS:Update IP", "Data"=w835, "error in (no error)"=w834) -> ("error out"=w831:errorcluster)  [unwired: 8 in]
        n414 = call "Messaging EnQ Multiline String.vi"("Command(s)"="NS:Close Connection\nUI:Reinitialize Front Panel\nNS:Open Connection", "error in (no error)"=w831) -> ("error out"=w833:errorcluster)  [unwired: 9 in]
        n415 = disable-structure shown="Disabled" {
          disable-tunnel: w833 -> [w840 _]
          disable-tunnel: [w838 _] -> w830
          frame Disabled {
            n416 = call "Messaging EnQ Single.vi"("Command"="TCP:Close Connection", "error in (no error)"=w840) -> ("error out"=w838:errorcluster)  [unwired: 9 in]
          }
          frame Enabled {
          }
        }
      }
      frame "MACRO:Display Panel" {
        n417 = call "Messaging EnQ Multiline String.vi"("Command(s)"="UI:Arrange Controls\nUI:Visible Controls" ("Command"), "error in (no error)"=w854) -> ("error out"=w841:errorcluster)  [unwired: 9 in]
        n418 = To Variant(anything="°F" ("Command")) -> (Variant=w848:variant)
        n419 = call "Messaging EnQ Single.vi"("Command"="UI:Refresh Graph", "Data"=w848, "error in (no error)"=w841) -> ("error out"=w845:errorcluster)  [unwired: 8 in]
        n420 = Unbundle By Name(w853) -> ("Login"=w852:bool)
        n421 = To Variant(anything=w852) -> (Variant=w847:variant)
        n422 = call "Messaging EnQ Single.vi"("Command"="UI:Enable Controls", "Data"=w847, "error in (no error)"=w845) -> ("error out"=w843:errorcluster)  [unwired: 8 in]
        n423 = call "Messaging EnQ Single.vi"("Command"="UI:Reinitialize Front Panel" ("Command(s)"), "error in (no error)"=w843) -> ("error out"=w842:errorcluster)  [unwired: 9 in]
      }
      frame "MACRO:Shutdown" {
        (unwired) "UI:Front Panel State>>Close"
        # "Shutdown Process\n1. Stop Event Loop\n2. Stop Test\n3. Disconnection of Network Stream\n4. Disconnection of Network Shared Variable\n5. Disconnection of TCP\n6. Close Front Panel\n7. Logging, Stop Queue, and Exit"
        # "Add later"
        # "List of commands to send for shutting down."
        n424 = call "Messaging EnQ Multiline String.vi"("Command(s)"="NS:Close Connection\nSYS:Exit", "error in (no error)"=w858) -> ("error out"=w857:errorcluster)  [unwired: 9 in]
      }
      frame "------Network Stream------" {
        # "Deals with the Shared Variable Engine interface (network Streams)"
      }
      frame "NS:Detect Systems" {
        w864 = u32 0 items=["none"=0, "only if online"=1, "all"=3] ("Include Cached Results (all)")
        w865 = u32 18 items=["Hostname"=16, "Hostname (IP)"=18, "Hostname (MAC)"=19, "IP"=32, "IP (Hostname)"=33, "IP (MAC)"=35, "MAC"=48, "MAC (Hostname)"=49, "MAC (IP)"=50] ("Output (Hostname and IP)")
        n425 = call <vilib>:"Find Systems.vi"("error in (no error)"=w871, "Output (Hostname and IP)"=w865, "Include Cached Results (all)"=w864) -> ("error out"=w868:errorcluster, "Detected Systems"=w866:string[])  [unwired: 6 in, 1 out]
        "Detected Systems" <- w866
        n426 = property on="Menu Ring" class="Ring (strict)"(error in=w868, "Strings []"=w866, "Val(Sgnl)"=u16 0 ("Value (Signaling)")) -> (error out=w867:errorcluster)  [unwired: 1 in, 1 out]
        n427 = Bundle By Name(cluster=w870, "Detected Systems"=w866) -> (w869:T27)
      }
      frame "NS:Update IP" {
        (unwired) "CFX315" ("format string")
        n428 = Unbundle By Name(w881) -> ("Dataset.M1 Status.Package"=w875:string, "Detected Systems"=w879:string[])
        n429 = Variant To Data(error in=w885, type=0, Variant=w884) -> (data=w880:i32, error out=w877:errorcluster)
        n430 = Index Array(array=w879, index=w880) -> (element=w872:string)
        n431 = call "Update IP Address.vi"("error in"=w877, "Detected System"=w872, "Package Name"=w875) -> ("error out"=w876:errorcluster, "Shared Variable Address"=w873:string, "IP Address"=w874:string)  [unwired: 6 in]
        n432 = Bundle By Name(cluster=w881, "Connected System"=w872, "IP Address"=w874, "Shared Variable Address"=w873, "URI Directory"="/C/TTV Test Patterns/" ("relative uri")) -> (w883:T27)
      }
      frame "NS:Open Connection" {
        # "Create NS Writer Endpoint"
        # "Create NS Reader Endpoint"
        n433 = Unbundle By Name(w902) -> ("IP Address"=w900:string)
        n434 = Format Into String(format string="%s", initial string="//" ("string"), w900) -> (resulting string=w898:string)  [unwired: 1 in, 1 out]
        n435 = Concatenate Strings(w898, "/CFX315Writer" ("string")) -> (w911:string)
        n436 = Create Network Stream Reader Endpoint(5:1000 ("timeout in ms (-1)"), 7:1 ("reader buffer size"), 8:w905, 9:cluster{"Data":variant, "Timestamp":timestamp} {"Data"=variant, "Timestamp"=timestamp(0 s since 1904-01-01)} ("Dataset"), 10:w911, 11:"GUIReader1" ("reader name")) -> (0:w904:errorcluster, 3:w895:refnum<k21>)  [unwired: 1 in]
        n437 = Concatenate Strings(w898, "/CFX315Reader" ("writer name")) -> (w906:string)
        n438 = Create Network Stream Writer Endpoint(5:1000 ("timeout in ms (-1)"), 7:1 ("writer buffer size"), 8:w904, 9:variant, 10:w906, 11:"GUIWriter1" ("writer name")) -> (0:w897:errorcluster, 3:w896:refnum<k21>)  [unwired: 1 in]
        n439 = property class="Network Stream Endpoint"(reference=w896, error in=w897) -> (error out=w890:errorcluster, "Connected"=w886:bool)  [unwired: 1 out]
        n440 = Bundle By Name(cluster=w902, "System Ready"=FALSE, "reader endpoint"=w895, "writer endpoint"=w896, "Network Connection"=w886) -> (w894:T27)
        n441 = Unbundle By Name(w894) -> ("Connected System"=w893:string)
        n442 = Select(t="NS:Read\nUI:Module Enable" ("Command"), s=w886, f="NS:Open Connection" ("Command")) -> (s? t:f=w887:string)
        n443 = call "Messaging EnQ Multiline String.vi"("Command(s)"=w887, "error in (no error)"=w890) -> ("error out"=w892:errorcluster)  [unwired: 9 in]
      }
      frame "NS:Close Connection" {
        w917 = FALSE ("Network Connection")
        n444 = Unbundle By Name(w919) -> ("reader endpoint"=w922:refnum<k21>, "writer endpoint"=w921:refnum<k21>)
        n445 = Destroy Stream Endpoint(8:w924, 11:w921) -> (0:w923:errorcluster)
        n446 = Destroy Stream Endpoint(8:w923, 11:w922) -> (0:w920:errorcluster)
        n447 = Bundle By Name(cluster=w919, "Network Connection"=w917, "System Ready"=w917) -> (w918:T27)
      }
      frame "NS:Read" {
        n448 = Unbundle By Name(w931) -> ("Network Connection"=w925:bool, "Dataset"=w926:T32, "reader endpoint"=w930:refnum<k21>)
        n449 = shared-variable-read(w930, w937, 1000 ("timeout ms (-1)"), cluster{"Data":variant, "Timestamp":timestamp} {"Data"=variant, "Timestamp"=timestamp(0 s since 1904-01-01)} ("Dataset")) -> (w936:errorcluster, w935:bool, w934:cluster{"Data":variant, "Timestamp":timestamp})  [unwired: 1 out]
        n450 = Or(x=w935, y=w936) -> (x .or. y?=w939:bool)
        n451 = case shown="False" w939 {
          tunnel: [w957 w967] -> w940
          tunnel: w931 -> [w956 w968]
          tunnel: [w946 w965] -> w938
          tunnel: w926 -> [w952 _]
          tunnel: w936 -> [w950 w970]
          tunnel: w934 -> [w951 _]
          tunnel: w930 -> [_ w969]
          tunnel: [w945 FALSE ("Connected")] -> w929
          tunnel: [w944 _] -> w928
          tunnel: [w943 _] -> w927
          tunnel: w925 -> [w941 _]
          frame False {
            n452 = Unbundle By Name(w951) -> ("Timestamp"=→"Data Rx Timestamp":timestamp, "Data"=w955:variant)
            n453 = Variant To Data(error in=w950, type=w952, Variant=w955) -> (data=w953:T32, error out=w947:errorcluster)
            n454 = call "Messaging EnQ Single.vi"("Command"="UI:Update Network Down Data", "@Front?"=TRUE, "error in (no error)"=w947) -> ("error out"=w946:errorcluster)  [unwired: 8 in]
            n455 = call "Is Value Changed.vim"("value"=w941) -> ("changed or first call?"=w942:bool)
            n456 = case shown="False" w942 {
              tunnel: [FALSE ("Connected") w961] -> w945
              tunnel: ["" ("Name") "Start Streaming" ("Name")] -> w943
              tunnel: [FALSE ("Connected") w961] -> w944
              frame False {
              }
              frame True {
                w961 = TRUE ("Connected")
              }
            }
            n457 = Bundle By Name(cluster=w956, "Dataset"=w953) -> (w957:T27)
          }
          frame True {
            n458 = property class="Network Stream Endpoint"(reference=w969, error in=w970) -> (error out=w966:errorcluster, "Connected"=w964:bool)  [unwired: 1 out]
            n459 = case shown="False" w964 {
              tunnel: w966 -> [w975 w976]
              tunnel: [w973 w976] -> w965
              frame False {
                n460 = call <vilib>:"Clear Errors.vi"("error in (no error)"=w975) -> ("error out"=w974:errorcluster)  [unwired: 5 in, 1 out]
                n461 = call "Messaging EnQ Multiline String.vi"("Command(s)"="NS:Close Connection\nUI:Reinitialize Front Panel\nNS:Open Connection" ("Command"), "@Front?"=TRUE, "error in (no error)"=w974) -> ("error out"=w973:errorcluster)  [unwired: 8 in]
              }
              frame True {
              }
            }
            n462 = Bundle By Name(cluster=w968, "Network Connection"=w964) -> (w967:T27)
          }
        }
      }
      frame "NS:Write" {
        n463 = Index Array(array=w993) -> (element=w985:string)  [unwired: 1 in]
        n464 = case shown="\"M1 Enable\"" w985 {
          tunnel: w983 -> [w994 w1008 w1019 w1031 w1045 w1057 w1070 w1082 w1094 w1106 w1118 w1130 w1141 w1154 w1166]
          tunnel: [w996 w1006 w1017 w1030 w1043 w1055 w1068 w1080 w1092 w1105 w1112 w1124 w1142 w1151 w1162] -> w981
          tunnel: [w994 w1007 w1018 w1022 w1042 w1056 w1069 w1081 w1093 w1104 w1117 w1125 w1140 w1150 w1161] -> w980
          tunnel: w982 -> [w996 w1004 w1016 w1029 w1041 w1054 w1067 w1079 w1091 w1103 w1113 w1126 w1138 w1152 w1163]
          tunnel: ["No data to command" w1001 w1012 w1025 w1036 w1049 w1062 w1074 w1087 w1098 w1116 w1129 w1135 w1149 w1158] -> w979
          tunnel: [_ w1000 w1011 w1024 w1035 w1050 w1063 w1075 w1085 w1099 w1115 w1128 w1133 w1148 w1155] -> w978
          tunnel: w984 -> [_ w998 w1010 w1023 w1034 w1047 w1060 w1072 w1084 w1096 w1114 w1127 w1132 w1153 w1165]
          frame Default {
          }
          frame "Power On-Off" {
            w997 = NS_New_Data."System Power" ("New Data")
            n465 = Variant To Data(error in=w1008, type=TRUE, Variant=w998) -> (data=w1002:bool, error out=w1007:errorcluster)
            n466 = Bundle By Name(cluster=w1004, "Network Data Down.System Power On Off"=w1002, "Network Data Down.New Data"=w997) -> (w1006:T27)
            n467 = call <vilib>:"Space Constant.vi"() -> ("String"=w1003:string)
            n468 = Format Into String(w997) -> (resulting string=w999:string)  [unwired: 3 in, 1 out]
            n469 = Format Into String(w1002) -> (resulting string=w1000:string)  [unwired: 3 in, 1 out]
            n470 = Concatenate Strings(w999, w1003, w1000) -> (w1001:string)
          }
          frame "M1 Power Drive Control" {
            w1009 = NS_New_Data."M1 Power Drive" ("New Data")
            n471 = Variant To Data(error in=w1019, type=TRUE, Variant=w1010) -> (data=w1014:bool, error out=w1018:errorcluster)
            n472 = Format Into String(w1014) -> (resulting string=w1011:string)  [unwired: 3 in, 1 out]
            n473 = Bundle By Name(cluster=w1016, "Network Data Down.M1 Commands.Power Drive"=w1014, "Network Data Down.New Data"=w1009) -> (w1017:T27)
            n474 = call <vilib>:"Space Constant.vi"() -> ("String"=w1015:string)
            n475 = Format Into String(w1009) -> (resulting string=w1013:string)  [unwired: 3 in, 1 out]
            n476 = Concatenate Strings(w1013, w1015, w1011) -> (w1012:string)
          }
          frame "M2 Power Drive Control" {
            w1021 = NS_New_Data."M2 Power Drive" ("New Data")
            (unwired) FALSE ("data")
            n477 = Variant To Data(error in=w1031, type=TRUE, Variant=w1023) -> (data=w1027:bool, error out=w1022:errorcluster)
            n478 = Format Into String(w1027) -> (resulting string=w1024:string)  [unwired: 3 in, 1 out]
            n479 = Bundle By Name(cluster=w1029, "Network Data Down.M2 Commands.Power Drive"=w1027, "Network Data Down.New Data"=w1021) -> (w1030:T27)
            n480 = call <vilib>:"Space Constant.vi"() -> ("String"=w1028:string)
            n481 = Format Into String(w1021) -> (resulting string=w1026:string)  [unwired: 3 in, 1 out]
            n482 = Concatenate Strings(w1026, w1028, w1024) -> (w1025:string)
          }
          frame "M1 Set Temp" {
            w1033 = NS_New_Data."M1 Set Point" ("New Data")
            n483 = Variant To Data(error in=w1045, type=20.0 ("SET TEMP 1"), Variant=w1034) -> (data=w1039:dbl, error out=w1042:errorcluster)
            n484 = Number To Fractional String(number=w1039, precision (6)=i16 1) -> (F-format string=w1035:string)  [unwired: 2 in]
            n485 = Bundle By Name(cluster=w1041, "Network Data Down.M1 Commands.Set Temp"=w1039, "Network Data Down.New Data"=w1033) -> (w1043:T27)
            n486 = Format Into String(w1033) -> (resulting string=w1037:string)  [unwired: 3 in, 1 out]
            n487 = call <vilib>:"Space Constant.vi"() -> ("String"=w1038:string)
            n488 = Concatenate Strings(w1037, w1038, w1035) -> (w1036:string)
          }
          frame "M2 Set Temp" {
            w1046 = NS_New_Data."M2 Set Point" ("New Data")
            n489 = Variant To Data(error in=w1057, type=0.0 ("SET TEMP 1"), Variant=w1047) -> (data=w1051:dbl, error out=w1056:errorcluster)
            n490 = Number To Fractional String(number=w1051, precision (6)=i16 1) -> (F-format string=w1050:string)  [unwired: 2 in]
            n491 = Bundle By Name(cluster=w1054, "Network Data Down.M2 Commands.Set Temp"=w1051, "Network Data Down.New Data"=w1046) -> (w1055:T27)
            n492 = Format Into String(w1046) -> (resulting string=w1048:string)  [unwired: 3 in, 1 out]
            n493 = call <vilib>:"Space Constant.vi"() -> ("String"=w1053:string)
            n494 = Concatenate Strings(w1048, w1053, w1050) -> (w1049:string)
          }
          frame "M1 Feedback" {
            w1059 = NS_New_Data."M1 Feedback" ("New Data")
            n495 = Variant To Data(error in=w1070, type=u8 0 ("Network Data Down.M1 Commands.Feedback"), Variant=w1060) -> (data=w1065:u8, error out=w1069:errorcluster)
            n496 = Format Into String(w1065) -> (resulting string=w1063:string)  [unwired: 3 in, 1 out]
            n497 = Bundle By Name(cluster=w1067, "Network Data Down.M1 Commands.Feedback"=w1065, "Network Data Down.New Data"=w1059) -> (w1068:T27)
            n498 = Format Into String(w1059) -> (resulting string=w1061:string)  [unwired: 3 in, 1 out]
            n499 = call <vilib>:"Space Constant.vi"() -> ("String"=w1064:string)
            n500 = Concatenate Strings(w1061, w1064, w1063) -> (w1062:string)
          }
          frame "M2 Feedback" {
            w1071 = NS_New_Data."M2 Feedback" ("New Data")
            n501 = Variant To Data(error in=w1082, type=u8 0 ("Network Data Down.M2 Commands.Feedback"), Variant=w1072) -> (data=w1073:u8, error out=w1081:errorcluster)
            n502 = Bundle By Name(cluster=w1079, "Network Data Down.M2 Commands.Feedback"=w1073, "Network Data Down.New Data"=w1071) -> (w1080:T27)
            n503 = Format Into String(w1073) -> (resulting string=w1075:string)  [unwired: 3 in, 1 out]
            n504 = Format Into String(w1071) -> (resulting string=w1076:string)  [unwired: 3 in, 1 out]
            n505 = call <vilib>:"Space Constant.vi"() -> ("String"=w1077:string)
            n506 = Concatenate Strings(w1076, w1077, w1075) -> (w1074:string)
          }
          frame "M1 Package" {
            w1083 = NS_New_Data."M1 Package" ("New Data")
            n507 = Variant To Data(error in=w1094, type=u16 0 ("Network Data Down.M1 Commands.Package"), Variant=w1084) -> (data=w1088:u16, error out=w1093:errorcluster)
            n508 = Bundle By Name(cluster=w1091, "Network Data Down.M1 Commands.Package"=w1088, "Network Data Down.New Data"=w1083) -> (w1092:T27)
            n509 = Format Into String(w1088) -> (resulting string=w1085:string)  [unwired: 3 in, 1 out]
            n510 = Format Into String(w1083) -> (resulting string=w1086:string)  [unwired: 3 in, 1 out]
            n511 = call <vilib>:"Space Constant.vi"() -> ("String"=w1089:string)
            n512 = Concatenate Strings(w1086, w1089, w1085) -> (w1087:string)
          }
          frame "M2 Package" {
            w1095 = NS_New_Data."M2 Package" ("New Data")
            n513 = Variant To Data(error in=w1106, type=u16 0 ("Network Data Down.M2 Commands.Package"), Variant=w1096) -> (data=w1100:u16, error out=w1104:errorcluster)
            n514 = Bundle By Name(cluster=w1103, "Network Data Down.M2 Commands.Package"=w1100, "Network Data Down.New Data"=w1095) -> (w1105:T27)
            n515 = Format Into String(w1100) -> (resulting string=w1099:string)  [unwired: 3 in, 1 out]
            n516 = Format Into String(w1095) -> (resulting string=w1097:string)  [unwired: 3 in, 1 out]
            n517 = call <vilib>:"Space Constant.vi"() -> ("String"=w1101:string)
            n518 = Concatenate Strings(w1097, w1101, w1099) -> (w1098:string)
          }
          frame "M1 Enable" {
            w1108 = NS_New_Data."M1 Enable" ("New Data")
            n519 = Variant To Data(error in=w1118, type=TRUE, Variant=w1114) -> (data=w1107:bool, error out=w1117:errorcluster)
            n520 = Bundle By Name(cluster=w1113, "Network Data Down.M1 Commands.Enable"=w1107, "Network Data Down.New Data"=w1108) -> (w1112:T27)
            n521 = Format Into String(w1107) -> (resulting string=w1115:string)  [unwired: 3 in, 1 out]
            n522 = Format Into String(w1108) -> (resulting string=w1109:string)  [unwired: 3 in, 1 out]
            n523 = call <vilib>:"Space Constant.vi"() -> ("String"=w1110:string)
            n524 = Concatenate Strings(w1109, w1110, w1115) -> (w1116:string)
          }
          frame "M2 Enable" {
            w1119 = NS_New_Data."M2 Enable" ("New Data")
            n525 = Variant To Data(error in=w1130, type=TRUE, Variant=w1127) -> (data=w1121:bool, error out=w1125:errorcluster)
            n526 = Bundle By Name(cluster=w1126, "Network Data Down.M2 Commands.Enable"=w1121, "Network Data Down.New Data"=w1119) -> (w1124:T27)
            n527 = Format Into String(w1121) -> (resulting string=w1128:string)  [unwired: 3 in, 1 out]
            n528 = Format Into String(w1119) -> (resulting string=w1120:string)  [unwired: 3 in, 1 out]
            n529 = call <vilib>:"Space Constant.vi"() -> ("String"=w1122:string)
            n530 = Concatenate Strings(w1120, w1122, w1128) -> (w1129:string)
          }
          frame "Update Config" {
            w1131 = NS_New_Data."Config Data" ("New Data")
            w1133 = "Download"
            w1137 = T36 {"Packages"={"DUT Force lbf"={" 0"=0, " 1"=0, " 2"=0, "3"=0, "4"=0, "5"=0, " 6"=0, "7"=0, "8"=0, "9"=0}, "DUT Names"={"0"="", "1"="", "2"="", "3"="", "4"="", "5"="", "6"="", "7"="", "8"="", "9"=""}}, "Heater PID"={"P"=0.0, "I"=0.0, "D"=0.0}, "Piston Settings"={"Forces Slope"=0.0, "Forces Intercept"=0.0, "Transition Force"=0.0, "Up Force"=0.0, "Diameter (mm)"=0.0, "Delay (ms)"=0.0, "Pressure Ramp Delay (ms)"=0.0}, "Safe Temps"={"Minimum"=17, "Enabled"=TRUE, "Maximum"=95}, "System Settings"={"Number of Heads"=0, "60Hz Power"=TRUE, "FTC200"=TRUE, "AutoStartup"=FALSE, "Purge"=TRUE, "Sensors"=TRUE, "HandClamp"=TRUE, "ATE"=TRUE, "Benchtop"=TRUE, "Production"=TRUE, "Refrigerant"=0, "Handler"=TRUE, "Shuttle"=TRUE, "220V"=FALSE, "Cascade"=FALSE, "Suction Sensor"=0, "Discharge Sensor"=0}, "Stepper Settings "={"Microstepping"=0, "Velocity"=8}, "Set Point Range"={"Max"=0.0, "Min"=0.0}, "Pedestal Check DeltaT"=0.0, "Ramp Delta T"=0.0, "Ramp-SS Threshold"=0.0, "SS Tolerance"=0.0, "EEV PID"={"Ramp Up Target"=0.0, "Ramp Down Target"=0.0, "Steady State Target"=0.0, "Output"={"Max"=0.0, "Min"=0.0}, "EBB and Flow Temp TH"=0.0, "Cryomode EEV Max"=0.0, "Valve minimum opening "=0.0, "Ramp Up EEV Steps"=0.0, "Ramp Down EEV Steps"=0.0, "SS EEV Steps Reset"=0.0, "EBB and Flow Tol"=0.0, "Gains"={"P"=0.0, "I"=0.0, "D"=0.0}, "Dissabled Target"=0.0, "CryoMode Gains"={"P"=0.0, "I"=0.0, "D"=0.0}, "M1 SuperHeat Setpoint"=0.0, "M2 Gains"={"P"=0.0, "I"=0.0, "D"=0.0}, "Flow Curve"=0}, "Sleep Timeout"=0.0, "Bypass Values"={"Bypass Valve"=TRUE, "Flow Curve"=0, "Output"={"Max"=0, "Min"=0}, "Feedback"=0, "Cyth Bypass"=TRUE, "PID"={"P"=0.0, "I"=0.0, "D"=0.0}, "Pressure setpoint"=0, "Cryo Temp"=0, "Superheat Setpoint"=0, "Cryo Setpoint"=0}, "Default Temp"=0.0, "InTEC"={"Enabled"=FALSE, "IP"="192.168.1.100", "Port"=5000}, "M1 TSD"={"Gain"=0.0, "Offset"=0.0, "V Offset "=0.0}, "M2 TSD"={"Gain"=0.0, "Offset"=0.0, "V Offset "=0.0}, "M1 T-Case Calibration"={"Gain"=0.0, "Offset"=0.0}, "M2 T-Case Calibration"={"Gain"=0.0, "Offset"=0.0}, "Heater PID TSD"={"P"=0.0, "I"=0.0, "D"=0.0}, "M2 Heater PID"={"P"=0.0, "I"=0.0, "D"=0.0}}  # Config Data
            n531 = Variant To Data(error in=w1141, type=w1137, Variant=w1132) -> (data=w1139:T36, error out=w1140:errorcluster)
            n532 = Bundle By Name(cluster=w1138, "Network Data Down.Config Data"=w1139, "Network Data Down.New Data"=w1131) -> (w1142:T27)
            n533 = Format Into String(w1131) -> (resulting string=w1134:string)  [unwired: 3 in, 1 out]
            n534 = call <vilib>:"Space Constant.vi"() -> ("String"=w1136:string)
            n535 = Concatenate Strings(w1134, w1136, w1133) -> (w1135:string)
          }
          frame "Reboot RT" {
            w1144 = NS_New_Data."Stop RT" ("Network Data Down.New Data")
            # "Change Reboot"
            n536 = Variant To Data(error in=w1154, type=TRUE ("Stop RT"), Variant=w1153) -> (data=w1143:bool, error out=w1150:errorcluster)
            n537 = Format Into String(w1143) -> (resulting string=w1148:string)  [unwired: 3 in, 1 out]
            n538 = Format Into String(w1144) -> (resulting string=w1145:string)  [unwired: 3 in, 1 out]
            n539 = Bundle By Name(cluster=w1152, "Network Data Down.Stop RT"=w1143, "Network Data Down.New Data"=w1144) -> (w1151:T27)
            n540 = call <vilib>:"Space Constant.vi"() -> ("String"=w1146:string)
            n541 = Concatenate Strings(w1145, w1146, w1148) -> (w1149:string)
          }
          frame "Stop RT" {
            w1157 = NS_New_Data."Stop RT" ("Network Data Down.New Data")
            n542 = Variant To Data(error in=w1166, type=TRUE ("STop RT"), Variant=w1165) -> (data=w1156:bool, error out=w1161:errorcluster)
            n543 = Format Into String(w1156) -> (resulting string=w1155:string)  [unwired: 3 in, 1 out]
            n544 = Format Into String(w1157) -> (resulting string=w1159:string)  [unwired: 3 in, 1 out]
            n545 = Bundle By Name(cluster=w1163, "Network Data Down.Stop RT"=w1156, "Network Data Down.New Data"=w1157) -> (w1162:T27)
            n546 = call <vilib>:"Space Constant.vi"() -> ("String"=w1160:string)
            n547 = Concatenate Strings(w1159, w1160, w1155) -> (w1158:string)
          }
        }
        n548 = Unbundle By Name(w981) -> ("writer endpoint"=w991:refnum<k21>, "Network Data Down"=w988:T28)
        n549 = To Variant(anything=w988) -> (Variant=w987:variant)
        n550 = shared-variable-write(w991, w980, w987) -> (w990:refnum<k21>, w992:errorcluster)  [unwired: 1 in, 1 out]
        n551 = Flush Stream(8:w992, 9:0 ("timeout in ms (-1)"), 11:w990) -> (0:w989:errorcluster)  [unwired: 1 in, 2 out]
      }
      frame "----Network Shared Variables-----" {
      }
      frame "NSV:Write" {
        n552 = Unbundle By Name(w1179) -> ("IP Address"=w1178:string)
        n553 = Index Array(array=w1176) -> (element=w1171:string)  [unwired: 1 in]
        n554 = Concatenate Strings("ni.var.psp://", w1178, "/Network Shared Variables/") -> (w1177:string)
        n555 = case shown="Default" w1171 {
          selector: w1171 -> [_ w1188 w1200 w1212 w1224 w1236 _ w1257 _ _]
          tunnel: w1177 -> [_ w1189 w1201 w1213 w1225 w1237 w1241 w1258 w1267 w1277]
          tunnel: w1175 -> [w1182 w1192 w1204 w1216 w1228 w1240 w1253 w1263 w1273 w1283]
          tunnel: w1174 -> [_ w1191 w1203 w1215 w1227 w1239 w1252 w1262 w1272 w1282]
          tunnel: [w1182 w1184 w1197 w1209 w1221 w1233 w1247 w1261 w1270 w1280] -> w1173
          tunnel: [_ _ w1195 w1207 w1218 w1230 _ _ _ _] -> w1170
          tunnel: [_ _ _ _ _ _ _ _ w1264 w1274] -> w1169
          frame Default {
          }
          frame "Cascade Compressor controls" {
            n556 = Variant To Data(error in=w1192, type=T23 {"High Stage manual speed control"=FALSE, "Manual High stage frequency"=0.0, "Low Stage manual speed control"=FALSE, "Manual Low Stage frequency"=0.0} ("Cascade Compressor controls"), Variant=w1191) -> (data=w1186:T23, error out=w1187:errorcluster)
            n557 = Format Into String(format string="%s", initial string=w1189, w1188) -> (resulting string=w1185:string)  [unwired: 1 in, 1 out]
            n558 = shared-variable-write(w1185, w1187, w1186) -> (w1184:errorcluster)  [unwired: 1 out]
          }
          frame "M2 EEV Manual" {
            n559 = Variant To Data(error in=w1204, type=i16 0 ("M2 EEV Manual control"), Variant=w1203) -> (data=w1194:i16, error out=w1199:errorcluster)
            n560 = Format Into String(format string="%s", initial string=w1201, w1200) -> (resulting string=w1198:string)  [unwired: 1 in, 1 out]
            n561 = shared-variable-write(w1198, w1199, w1194) -> (w1197:errorcluster)  [unwired: 1 out]
            n562 = Number To Engineering String(2:i16 1 ("precision (6)"), 4:w1194) -> (0:w1195:string)  [unwired: 2 in]
          }
          frame "M1 EEV Manual" {
            n563 = Variant To Data(error in=w1216, type=i16 0 ("M2 EEV Manual control"), Variant=w1215) -> (data=w1206:i16, error out=w1211:errorcluster)
            n564 = Format Into String(format string="%s", initial string=w1213, w1212) -> (resulting string=w1210:string)  [unwired: 1 in, 1 out]
            n565 = shared-variable-write(w1210, w1211, w1206) -> (w1209:errorcluster)  [unwired: 1 out]
            n566 = Number To Engineering String(2:i16 1 ("precision (6)"), 4:w1206) -> (0:w1207:string)  [unwired: 2 in]
          }
          frame "M1 Heater output" {
            n567 = Variant To Data(error in=w1228, type=0.0 ("M1 Heater PWM"), Variant=w1227) -> (data=w1219:dbl, error out=w1223:errorcluster)
            n568 = Format Into String(format string="%s", initial string=w1225, w1224) -> (resulting string=w1222:string)  [unwired: 1 in, 1 out]
            n569 = shared-variable-write(w1222, w1223, w1219) -> (w1221:errorcluster)  [unwired: 1 out]
            n570 = Number To Engineering String(2:i16 1 ("precision (6)"), 4:w1219) -> (0:w1218:string)  [unwired: 2 in]
          }
          frame "M2 Heater Output" {
            n571 = Variant To Data(error in=w1240, type=0.0 ("M1 Heater PWM"), Variant=w1239) -> (data=w1231:dbl, error out=w1235:errorcluster)
            n572 = Format Into String(format string="%s", initial string=w1237, w1236) -> (resulting string=w1234:string)  [unwired: 1 in, 1 out]
            n573 = shared-variable-write(w1234, w1235, w1231) -> (w1233:errorcluster)  [unwired: 1 out]
            n574 = Number To Engineering String(2:i16 1 ("precision (6)"), 4:w1231) -> (0:w1230:string)  [unwired: 2 in]
          }
          frame "Thermal Load" {
            n575 = Variant To Data(error in=w1253, type=0.0 ("Numeric"), Variant=w1252) -> (data=w1248:dbl, error out=w1246:errorcluster)
            n576 = Format Into String(format string="%s", initial string=w1241, "Network Inputs" ("input 1")) -> (resulting string=w1242:string)  [unwired: 1 in, 1 out]
            n577 = Replace Array Subset(array=dbl[] [0.0, 0.0], new element=w1248, index=0) -> (w1245:dbl[])
            n578 = shared-variable-write(w1242, w1246, w1245) -> (w1247:errorcluster)  [unwired: 1 out]
          }
          frame "Manual Bypass Mode" {
            n579 = Variant To Data(error in=w1263, type=bool[] [] ("Manual Bypass Mode"), Variant=w1262) -> (data=w1255:bool[], error out=w1260:errorcluster)
            n580 = Format Into String(format string="%s", initial string=w1258, w1257) -> (resulting string=w1256:string)  [unwired: 1 in, 1 out]
            n581 = shared-variable-write(w1256, w1260, w1255) -> (w1261:errorcluster)  [unwired: 1 out]
          }
          frame "M1 TSD Feedback" {
            n582 = Variant To Data(error in=w1273, type=FALSE ("TSD Feedback"), Variant=w1272) -> (data=w1264:bool, error out=w1269:errorcluster)
            n583 = Format Into String(format string="%s", initial string=w1267, "TSD Feedback" ("input 1")) -> (resulting string=w1266:string)  [unwired: 1 in, 1 out]
            n584 = shared-variable-write(w1266, w1269, w1264) -> (w1270:errorcluster)  [unwired: 1 out]
          }
          frame "M2 TSD Feedback" {
            n585 = Variant To Data(error in=w1283, type=FALSE ("TSD Feedback"), Variant=w1282) -> (data=w1274:bool, error out=w1279:errorcluster)
            n586 = Format Into String(format string="%s", initial string=w1277, "TSD Feedback" ("input 1")) -> (resulting string=w1276:string)  [unwired: 1 in, 1 out]
            n587 = shared-variable-write(w1276, w1279, w1274) -> (w1280:errorcluster)  [unwired: 1 out]
          }
        }
      }
      frame "NSV:Read" {
        n588 = Unbundle By Name(w1288) -> ("IP Address"=w1289:string)
        n589 = Concatenate Strings("ni.var.psp://", w1289, "/Network Shared Variables/") -> (w1287:string)
        n590 = for {
          tunnel: w1285 -> [w1294]
          tunnel: [w1295] -> w1284
          tunnel: w1286 -> [w1293] mode=indexing
          tunnel: w1287 -> [w1292]
          n591 = Concatenate Strings(w1292, w1293) -> (w1296:string)
          n592 = case shown="\"TCP Command\"" w1293 {
            tunnel: w1294 -> [w1301 w1312 w1328 w1345 w1351 w1357 w1362 w1367 w1372 w1377 w1384 w1389 w1401 w1404 w1419]
            tunnel: [w1299 w1302 w1313 w1345 w1350 w1356 w1360 w1365 w1371 w1373 w1383 w1388 w1397 w1402 w1418] -> w1295
            tunnel: w1296 -> [w1300 w1311 w1327 _ w1349 w1355 w1361 w1366 w1369 w1376 w1382 w1387 w1400 w1406 w1421]
            frame "BootupTime" {
              n593 = shared-variable-read(w1300, w1301, timestamp(0 s since 1904-01-01)) -> (w1299:errorcluster, →"Boot Up Time":timestamp)  [unwired: 2 out]
            }
            frame "Output Cluster" {
              # "Read the RT Information to debug GUI"
              n594 = shared-variable-read(w1311, w1312, T5 {"Condensing Pressure"=0.0, "Suction Pressure"=0.0, "Bypass steps"=0, "Operating Time"=0.0, "SubCooling"=0.0, "Superheat"=0.0, "M1 Superheat"=0.0, "M2 Superheat"=0.0, "Autotune output"=0.0, "M1 Testing Elapsed Time"=0.0, "M2 Testing Elapsed Time"=0.0, "M1 Valve Control Mode"=0, "System Amps"=0.0, "Compressor Run Time"=0.0, "SD card free Space"=0.0, "Free Memory"=0.0, "M1 Pressure Feedback"=0.0, "M2 Pressure Feedback"=0.0, "Compression Ratio"=0.0, "Serial Number"=0.0, "M1 AC Load V"=0.0, "M1 AC Load W"=0.0, "M1 DC Load W"=0.0, "M1 RH"=0.0, "RH Threshold"=0.0} ("output cluster")) -> (w1302:errorcluster, w1309:T5)  [unwired: 2 out]
              "data out" <- w1309
              n595 = Unbundle By Name(w1309) -> ("RH Threshold"=w1304:dbl, "M1 RH"=w1305:dbl, "M1 Superheat"=→"M1 Superheat":dbl, "M1 Testing Elapsed Time"=→"M1 Testing Elapsed Time":dbl, "M1 AC Load V"=→"M1 AC Load V":dbl)
              n596 = Bundle("RH Threshold"=w1304, "M1 RH"=w1305) -> (→"M1 Humidity":cluster{"RH Threshold":dbl, "M1 RH":dbl})  [unwired: 1 in]
            }
            frame "TSD" {
              n597 = shared-variable-read(w1327, w1328, T3 {"TSD Millivolts"=0.0, "X factor"=0.0, "Offset"=0.0, "TSD Temp"=0.0, "TSD Feedback"=FALSE, "TSD Max"=0.0, "TSD Min"=0.0} ("TSD Data")) -> (w1314:errorcluster, w1323:T3)  [unwired: 2 out]
              n598 = Unbundle By Name(w1323) -> ("TSD Millivolts"=w1325:dbl, "X factor"=w1319:dbl, "Offset"=w1318:dbl)
              n599 = in-place {
                in-place-border: "Change TSD" -> [w1335]
                in-place-border: w1314 -> [w1330]
                in-place-border: [w1329] -> w1313
                n600 = in-place-match #1(w1319) -> (w1334:dbl)
                n601 = in-place-match #2(w1318) -> (w1332:dbl)
                n602 = case shown="False" w1335 {
                  tunnel: w1334 -> [w1338 w1344]
                  tunnel: [w1338 w1342] -> w1333
                  tunnel: w1332 -> [w1337 w1343]
                  tunnel: [w1337 w1341] -> w1331
                  tunnel: w1330 -> [w1336 w1340]
                  tunnel: [w1336 w1339] -> w1329
                  frame False {
                  }
                  frame True {
                    n603 = call "New TSD Values.vi"("Error In"=w1340, "Offset"=w1343, "X factor"=w1344) -> ("Error Out"=w1339:errorcluster, "Offset out"=w1341:dbl, "X factor out"=w1342:dbl)  [unwired: 6 in]
                  }
                }
                n604 = in-place-match #1(w1333) -> (w1317:dbl)
                n605 = in-place-match #2(w1331) -> (w1316:dbl)
              }
              n606 = Equal To 0?(x=w1325) -> (x = 0?=w1324:bool)
              n607 = Select(t=nan, s=w1324, f=w1325) -> (s? t:f=w1322:dbl)
              n608 = Bundle By Name(cluster=w1323, "TSD Millivolts"=w1322, "X factor"=w1317, "Offset"=w1316) -> (→"TSD Data":T3)
            }
            frame "DC PS Load Watts" {
              # "We dont use DC power Supply Anymore, now the TTV uses AC programmable power supply.  It tells the cobra exaclty how many watts the TTV is producing"
              # "This is for testing and datalogging purpose"
            }
            frame "Event Log" {
              n609 = shared-variable-read(w1349, w1351, T20 [] ("Event Log")) -> (w1350:errorcluster, w1347:T20)  [unwired: 2 out]
              n610 = call "Is Value Changed.vim"("value"=w1347) -> ("changed or first call?"=w1346:bool)
              n611 = case shown="True" w1346 {
                tunnel: w1347 -> [_ w1352]
                frame False {
                }
                frame True {
                  "Event log" <- w1352
                }
              }
            }
            frame "AI", Default {
              # "NVIDIA Testing"
              # "Analog Inputs"
              n612 = shared-variable-read(w1355, w1357, dbl[] [] ("AI (V) 2")) -> (w1356:errorcluster, →"AI (V)":dbl[])  [unwired: 2 out]
            }
            frame "Errors" {
              n613 = shared-variable-read(w1361, w1362, string[] [] ("Errors 2")) -> (w1360:errorcluster, →"Errors" →"Error":string[])  [unwired: 2 out]
            }
            frame "TCP Command" {
              # "The list of ports with connection status"
              n614 = shared-variable-read(w1366, w1367, string[] [] ("Errors 2")) -> (w1365:errorcluster, →"TCP commands":string[])  [unwired: 2 out]
            }
            frame "compressor manual frequency control" {
              w1370 = T23 {"High Stage manual speed control"=FALSE, "Manual High stage frequency"=0.0, "Low Stage manual speed control"=FALSE, "Manual Low Stage frequency"=0.0}  # Cascade Compressor controls
              # "king cobra compressor RPM"
              n615 = shared-variable-read(w1369, w1372, w1370) -> (w1371:errorcluster, w1368:T23)  [unwired: 2 out]
              n616 = local write "Cascade Compressor controls"(w1368) -> ()
            }
            frame "Stack Light State" {
              # "Monitoring RT Status"
              n617 = shared-variable-read(w1376, w1377, T2."Sleeping Fault" ("Stack light states")) -> (w1373:errorcluster, →"Stack light states":T2)  [unwired: 2 out]
            }
            frame "M1 Values" {
              # "Array that includes EEV PID Output"
              n618 = shared-variable-read(w1382, w1384, dbl[] [0.0, 0.0]) -> (w1383:errorcluster, w1380:dbl[])  [unwired: 2 out]
              n619 = Index Array(array=w1380) -> (element #1=→"M1 Buffer":dbl, element #2=→"M1 Valve Output":dbl)  [unwired: 2 in]
            }
            frame "M2 Values" {
              n620 = disable-structure shown="Disabled" {
                disable-tunnel: [w1396 _] -> w1391
                disable-tunnel: dbl[] [0.0, 0.0] -> [w1395 _]
                disable-tunnel: w1389 -> [w1394 _]
                disable-tunnel: [w1393 _] -> w1388
                disable-tunnel: w1387 -> [w1392 _]
                frame Disabled {
                  n621 = shared-variable-read(w1392, w1394, w1395) -> (w1393:errorcluster, w1396:dbl[])  [unwired: 2 out]
                }
                frame Enabled {
                }
              }
              n622 = Index Array(array=w1391) -> (element #1=→"M2 Buffer":dbl, element #2=→"M2 Valve Output":dbl)  [unwired: 2 in]
            }
            frame "TCP Connections" {
              n623 = shared-variable-read(w1400, w1401, T22 [{"port "=1300, "remote address"="", "Connection timeout ms"=100, "Waiting for connection"=TRUE, "Waiting for Command"=TRUE, "timeout ms"=5000}] ("TCP Connections")) -> (w1397:errorcluster, →"TCP Connections":T22)  [unwired: 2 out]
            }
            frame "TSD Feedback" {
              n624 = shared-variable-read(w1406, w1404, FALSE ("data type")) -> (w1403:errorcluster, w1410:bool)  [unwired: 2 out]
              n625 = disable-structure shown="Enabled" {
                disable-tunnel: w1403 -> [w1414 _]
                disable-tunnel: [w1413 _] -> w1402
                frame Disabled {
                  n626 = flat-sequence {
                    tunnel: w1414 -> [w1416]
                    tunnel: [w1416] -> w1413
                    tunnel: u32 5000 ("milliseconds to wait") -> [w1415]
                    frame #0 {
                      n627 = Wait (ms)(milliseconds to wait=w1415) -> ()  [unwired: 1 out]
                    }
                  }
                }
                frame Enabled {
                }
              }
              n628 = call "Is Value Changed.vim"("value"=w1410) -> ("changed or first call?"=w1409:bool)
              n629 = Equal?(x=w1410, y=FALSE) -> (x = y?=w1411:bool)
              n630 = And(x=w1411, y=w1409) -> (x .and. y?=w1405:bool)
              n631 = case shown="False" w1405 {
                tunnel: w1410 -> [w1417 _]
                frame False {
                  n632 = property on="M1 TSD Feedback" class="Bool (strict)"("Value"=w1417) -> ()  [unwired: 2 in, 2 out]
                }
                frame True {
                }
              }
            }
            frame "M2 TSD Feedback" {
              n633 = disable-structure shown="Disabled" {
                disable-tunnel: [w1431 _] -> w1425
                disable-tunnel: FALSE ("data type") -> [w1430 _]
                disable-tunnel: w1421 -> [w1429 _]
                disable-tunnel: w1419 -> [w1428 _]
                disable-tunnel: [w1427 _] -> w1418
                frame Disabled {
                  n634 = shared-variable-read(w1429, w1428, w1430) -> (w1427:errorcluster, w1431:bool)  [unwired: 2 out]
                }
                frame Enabled {
                }
              }
              n635 = call "Is Value Changed.vim"("value"=w1425) -> ("changed or first call?"=w1424:bool)
              n636 = Equal?(x=w1425, y=FALSE) -> (x = y?=w1426:bool)
              n637 = And(x=w1426, y=w1424) -> (x .and. y?=w1420:bool)
              n638 = case shown="False" w1420 {
                tunnel: w1425 -> [w1432 _]
                frame False {
                  n639 = property on="M2 TSD Feedback" class="Bool (strict)"("Value"=w1432) -> ()  [unwired: 2 in, 2 out]
                }
                frame True {
                }
              }
            }
          }
        }
      }
      frame "--------WebDAV----------" {
      }
      frame "WEB:Open Session" {
        n640 = Unbundle By Name(w1448) -> ("IP Address"=w1449:string)
        n641 = Unbundle By Name(w1448) -> ("URI Directory"=w1437:string)
        n642 = Format Into String(format string="%s/files", initial string="http://" ("host uri prefix"), w1449) -> (resulting string=w1443:string)  [unwired: 1 in, 1 out]
        n643 = call "WebDAV FGV.vi"("WebDAV States"=WebDAV_states."Open Sess", "error in (no error)"=w1445, "host uri prefix"=w1443) -> ("error out"=w1441:errorcluster, "session handle out"=w1438:T51)  [unwired: 6 in, 1 out]
        n644 = call <vilib>:"Path Info.vi"("session handle"=w1438, "relative uri"=w1437, "error in (no error)"=w1441) -> ("is directory?"=w1439:bool, "error out"=w1440:errorcluster)  [unwired: 9 in, 2 out]
        n645 = case shown="True" w1439 {
          tunnel: w1440 -> [_ w1465]
          tunnel: w1437 -> [w1453 w1460]
          tunnel: [w1455 w1458] -> w1442
          tunnel: [string[] [] w1462] -> w1447
          tunnel: ["Create directory " ("String") w1459] -> w1436
          frame False {
            # "Don't connect the error in"
            n646 = call "WebDAV FGV.vi"("WebDAV States"=WebDAV_states."Create Dir", "relative uri"=w1453) -> ("error out"=w1455:errorcluster)  [unwired: 7 in, 2 out]
          }
          frame True {
            n647 = call "WebDAV FGV.vi"("WebDAV States"=WebDAV_states."Refresh Dir", "error in (no error)"=w1465, "relative uri"=w1460) -> ("error out"=w1458:errorcluster, "file list"=w1457:T52[])  [unwired: 6 in, 1 out]
            n648 = for {
              tunnel: w1457 -> [w1467] mode=indexing
              tunnel: [w1466] -> w1462 mode=indexing
              n649 = Unbundle By Name(w1467) -> ("display name"=w1466:string)
            }
            n650 = Index Array(array=w1462) -> (element=w1463:string)  [unwired: 1 in]
            n651 = property on="Pattern File" class="CmbBox"("Val(Sgnl)"=w1463, "Strings[]"=w1462) -> ()  [unwired: 2 in, 2 out]
            n652 = Concatenate Strings("Open WebDAV" ("String"), w1460) -> (w1459:string)
          }
        }
        n653 = Bundle By Name(cluster=w1448, "File list in SoM"=w1447) -> (w1446:T27)
      }
      frame "WEB:Close Session" {
        n654 = call "WebDAV FGV.vi"("WebDAV States"=WebDAV_states."Close Sess", "error in (no error)"=w1474) -> ("error out"=w1473:errorcluster)  [unwired: 7 in, 2 out]
        n655 = Unbundle By Name(w1471) -> ("URI Directory"=w1470:string)
        n656 = Concatenate Strings("Close WebDAV  " ("String"), w1470) -> (w1469:string)
      }
      frame "-----------TCP-------------" {
      }
      frame "TCP:Open Connection" {
        w1489 = u16 3000  # port
        n657 = Unbundle By Name(w1485) -> ("IP Address"=w1491:string)
        n658 = TCP Open Connection(address=w1491, remote port or service name=w1489, error in (no error)=w1490) -> (connection ID=w1493:refnum<k5>, error out=w1492:errorcluster)  [unwired: 2 out]
        n659 = call-poly <vilib>:"Read Meta Data.vi"("error in"=w1492, "connection ID"=w1493) -> ("error out"=w1482:errorcluster, "connection info out"=w1481:T30)  [unwired: 1 in, 7 out]
        n660 = Unbundle By Name(w1481) -> ("connection ID"=w1480:refnum<k5>)
        n661 = Not A Number/Path/Refnum?(number/path/refnum=w1480) -> (NaN/Path/Refnum?=w1479:bool)
        n662 = Not(x=w1479) -> (.not. x?=w1478:bool)
        n663 = Bundle By Name(cluster=w1485, "TCP connection info"=w1481, "TCP Connection"=w1478) -> (w1484:T27)
        n664 = Number To Decimal String(number=w1489) -> (decimal integer string=w1483:string)  [unwired: 1 in]
      }
      frame "TCP:Read Dataset" {
        n665 = Unbundle By Name(w1496) -> ("Dataset"=w1497:T32, "TCP connection info"=w1498:T30)
        n666 = call-poly <vilib>:"Read Message.vi"("options"=T45 {"ignore timeout error"=TRUE, "timeout ms (1000)"=1000} ("Options"), "error in"=w1504, "connection info in"=w1498) -> ("error out"=w1502:errorcluster, "name"=w1500:T31, "data string"=w1501:string, "timed out?"=w1503:bool)  [unwired: 2 in, 3 out]
        n667 = case shown="False" w1503 {
          tunnel: w1501 -> [w1510 _]
          tunnel: w1500 -> [w1511 _]
          tunnel: w1502 -> [w1509 w1585]
          tunnel: [w1508 w1585] -> w1499
          tunnel: w1497 -> [w1507 _]
          tunnel: w1496 -> [w1506 w1584]
          tunnel: [w1505 w1584] -> w1495
          frame False {
            n668 = case shown="\"M1 History Data \"" w1511 {
              tunnel: w1510 -> [_ w1519 w1533 w1545 w1551 w1563 w1575]
              tunnel: w1509 -> [w1513 w1521 w1535 w1547 w1555 w1567 w1579]
              tunnel: [w1513 w1520 w1534 w1546 w1554 w1566 w1578] -> w1508
              tunnel: w1507 -> [_ _ _ w1543 w1550 w1562 w1574]
              tunnel: w1506 -> [w1512 w1516 w1530 w1542 w1553 w1565 w1577]
              tunnel: [w1512 w1515 w1529 w1542 w1552 w1564 w1576] -> w1505
              frame Default {
              }
              frame "M1 History Data " {
                n669 = Unflatten From JSON(JSON string=w1519, type and defaults=cluster{"Y":dbl[], "dt":dbl, "t0":dbl}[] [], error in (no error)=w1521) -> (value=w1517:cluster{"Y":dbl[], "dt":dbl, "t0":dbl}[], error out=w1520:errorcluster)  [unwired: 4 in]
                n670 = for {
                  tunnel: w1517 -> [w1524] mode=indexing
                  tunnel: [w1523] -> w1514 mode=indexing
                  tunnel: [w1522] -> _ mode=indexing
                  n671 = Unbundle By Name(w1524) -> ("t0"=w1526:dbl, "dt"=w1527:dbl, "Y"=w1523:dbl[])
                  n672 = To Time Stamp(1:w1526) -> (0:w1525:timestamp)
                  n673 = Bundle By Name("t0"=w1525, "dt"=w1527, "Y"=w1523) -> (w1522:waveform(dbl))  [unwired: 1 in]
                }
                n674 = Bundle By Name(cluster=w1516, "M1 History Temps"=w1514) -> (w1515:T27)
              }
              frame "M2 History Data" {
                n675 = Unflatten From JSON(JSON string=w1533, type and defaults=cluster{"Y":dbl[], "dt":dbl, "t0":dbl}[] [], error in (no error)=w1535) -> (value=w1531:cluster{"Y":dbl[], "dt":dbl, "t0":dbl}[], error out=w1534:errorcluster)  [unwired: 4 in]
                n676 = for {
                  tunnel: w1531 -> [w1538] mode=indexing
                  tunnel: [w1537] -> _ mode=indexing
                  tunnel: [w1536] -> w1528 mode=indexing
                  n677 = Unbundle By Name(w1538) -> ("t0"=w1540:dbl, "dt"=w1541:dbl, "Y"=w1536:dbl[])
                  n678 = To Time Stamp(1:w1540) -> (0:w1539:timestamp)
                  n679 = Bundle By Name("t0"=w1539, "dt"=w1541, "Y"=w1536) -> (w1537:waveform(dbl))  [unwired: 1 in]
                }
                n680 = Bundle By Name(cluster=w1530, "M2 History Temps"=w1528) -> (w1529:T27)
              }
              frame "System Module" {
                w1544 = T53 {"Power On Off"=FALSE, "Discharge Temp"=0.0, "Liquid Temp"=0.0, "Suction Temp"=0.0, "Ambient Temp"=0.0, "Sleep"=FALSE, "System Status"=0, "M1 Actuated"=FALSE, "M2 Actuated"=FALSE, "Sleep Timer"=0.0, "M1 Bin"={"Bin String"="", "Bin Color"=1}, "M2 Bin"={"Bin String"="", "Bin Color"=1}, "Discharge Pressure"=0.0, "Suction Pressure"=0.0, "Compression Ratio"=0.0, "Compressor Amps"=0.0, "Compressor Hours"=0.0, "Bypass Steps"=0, "SubCooling"=0.0, "SuperHeat"=0.0, "Serial Number"="", "EMO detected"=FALSE, "EMO Tripped"=FALSE, "Thermal cutoff"=FALSE, "Thermal cutoff 2"=FALSE, "High Pressure switch"=FALSE, "Running Time"="", "SOM Status"={"Boot Up Time"="", "Software Version"="", "CPU Usage"=0.0, "Memory Available"=0.0, "SD card free space"=0.0, "SOM Storage"=0.0}, "Cascade Extra"={"Discharge Temp High Side"=0.0, "Suction Temp High Side"=0.0, "Liquid Temp High side"=0.0, "Discharge Pressure 2"=0.0, "Suction Pressure 2"=0.0, "Low Side RPM"=0.0, "High Side RPM"=0.0}}  # System Status
                # "Timestamp can't unflatten from JSON"
                n681 = Unbundle By Name(w1543) -> ()  [unwired: 1 out]
                n682 = Unflatten From JSON(JSON string=w1545, type and defaults=w1544, error in (no error)=w1547) -> (error out=w1546:errorcluster)  [unwired: 4 in, 1 out]
              }
              frame "M1 Status" {
                n683 = Unbundle By Name(w1550) -> ("M1 Status"=w1549:T34)
                n684 = Unflatten From JSON(JSON string=w1551, type and defaults=w1549, error in (no error)=w1555) -> (value=w1548:T34, error out=w1554:errorcluster)  [unwired: 4 in]
                n685 = disable-structure shown="Disabled" {
                  disable-tunnel: w1553 -> [w1558 w1559]
                  disable-tunnel: [w1557 w1559] -> w1552
                  disable-tunnel: w1548 -> [w1556 _]
                  frame Disabled {
                    n686 = Bundle By Name(cluster=w1558, "Dataset.M1 Status"=w1556) -> (w1557:T27)
                  }
                  frame Enabled {
                  }
                }
              }
              frame "M2 Status" {
                n687 = Unbundle By Name(w1562) -> ("M2 Status"=w1561:T35)
                n688 = Unflatten From JSON(JSON string=w1563, type and defaults=w1561, error in (no error)=w1567) -> (value=w1560:T35, error out=w1566:errorcluster)  [unwired: 4 in]
                n689 = disable-structure shown="Enabled" {
                  disable-tunnel: w1565 -> [w1570 w1571]
                  disable-tunnel: [w1569 w1571] -> w1564
                  disable-tunnel: w1560 -> [w1568 _]
                  frame Disabled {
                    n690 = Bundle By Name(cluster=w1570, "Dataset.M2 Status"=w1568) -> (w1569:T27)
                  }
                  frame Enabled {
                  }
                }
              }
              frame "Config Data" {
                n691 = Unbundle By Name(w1574) -> ("Config Data"=w1573:T36)
                n692 = Unflatten From JSON(JSON string=w1575, type and defaults=w1573, error in (no error)=w1579) -> (value=w1572:T36, error out=w1578:errorcluster)  [unwired: 4 in]
                n693 = disable-structure shown="Enabled" {
                  disable-tunnel: w1577 -> [w1582 w1583]
                  disable-tunnel: [w1581 w1583] -> w1576
                  disable-tunnel: w1572 -> [w1580 _]
                  frame Disabled {
                    n694 = Bundle By Name(cluster=w1582, "Network Data Down.Config Data"=w1580) -> (w1581:T27)
                  }
                  frame Enabled {
                  }
                }
              }
            }
          }
          frame True {
          }
        }
      }
      frame "TCP:Write" {
        n695 = Index Array(array=w1594) -> (element=w1590:string)  [unwired: 1 in]
        n696 = case shown="\"Power On-Off\"" w1590 {
          tunnel: w1593 -> [w1598 w1605 w1611 w1618 w1628 w1636 w1645 w1653 w1661 w1669 w1676 w1683 w1690 w1697 w1704]
          tunnel: [w1598 w1601 w1608 w1614 w1624 w1630 w1640 w1647 w1656 w1664 w1675 w1681 w1685 w1695 w1700] -> w1587
          tunnel: w1592 -> [_ w1603 w1610 w1617 w1626 w1635 w1643 w1651 w1659 w1667 w1674 w1682 w1688 w1696 w1703]
          tunnel: [_ w1600 w1607 w1613 w1623 w1631 w1639 w1648 w1655 w1663 w1673 w1680 w1684 w1694 w1699] -> w1591
          tunnel: [_ w1599 w1606 _ _ _ _ _ _ _ w1672 w1679 _ w1693 w1698] -> w1589
          tunnel: [_ _ _ _ w1620 w1629 w1638 w1646 w1654 w1662 _ _ _ _ _] -> w1586
          frame Default {
            (unwired) "No data to command"
          }
          frame "Power On-Off" {
            n697 = Variant To Data(error in=w1605, type=TRUE, Variant=w1603) -> (data=w1599:bool, error out=w1602:errorcluster)
            n698 = call <vilib>:"Flatten To JSON String.vi"("error in (no error)"=w1602, "Variant"=w1599) -> ("error out"=w1601:errorcluster, "JSON String"=w1600:string)  [unwired: 8 in]
          }
          frame "M1 Power Drive Control" {
            n699 = Variant To Data(error in=w1611, type=TRUE, Variant=w1610) -> (data=w1606:bool, error out=w1609:errorcluster)
            n700 = call <vilib>:"Flatten To JSON String.vi"("error in (no error)"=w1609, "Variant"=w1606) -> ("error out"=w1608:errorcluster, "JSON String"=w1607:string)  [unwired: 8 in]
          }
          frame "M2 Power Drive Control" {
            n701 = Variant To Data(error in=w1618, type=TRUE, Variant=w1617) -> (data=w1615:bool, error out=w1616:errorcluster)
            n702 = call <vilib>:"Flatten To JSON String.vi"("error in (no error)"=w1616, "Variant"=w1615) -> ("error out"=w1614:errorcluster, "JSON String"=w1613:string)  [unwired: 8 in]
          }
          frame "M1 Set Temp" {
            n703 = Variant To Data(error in=w1628, type=20.0 ("SET TEMP 1"), Variant=w1626) -> (data=w1621:dbl, error out=w1625:errorcluster)
            n704 = call <vilib>:"Flatten To JSON String.vi"("error in (no error)"=w1625, "Variant"=w1621) -> ("error out"=w1624:errorcluster, "JSON String"=w1623:string)  [unwired: 8 in]
            n705 = Number To Engineering String(2:i16 1 ("precision (6)"), 4:w1621) -> (0:w1620:string)  [unwired: 2 in]
          }
          frame "M2 Set Temp" {
            n706 = Variant To Data(error in=w1636, type=0.0 ("SET TEMP 1"), Variant=w1635) -> (data=w1633:dbl, error out=w1632:errorcluster)
            n707 = call <vilib>:"Flatten To JSON String.vi"("error in (no error)"=w1632, "Variant"=w1633) -> ("error out"=w1630:errorcluster, "JSON String"=w1631:string)  [unwired: 8 in]
            n708 = Number To Engineering String(2:i16 1 ("precision (6)"), 4:w1633) -> (0:w1629:string)  [unwired: 2 in]
          }
          frame "M1 Feedback" {
            n709 = Variant To Data(error in=w1645, type=u8 0 ("Network Data Down.M1 Commands.Feedback"), Variant=w1643) -> (data=w1641:u8, error out=w1642:errorcluster)
            n710 = call <vilib>:"Flatten To JSON String.vi"("error in (no error)"=w1642, "Variant"=w1641) -> ("error out"=w1640:errorcluster, "JSON String"=w1639:string)  [unwired: 8 in]
            n711 = Format Into String(w1641) -> (resulting string=w1638:string)  [unwired: 3 in, 1 out]
          }
          frame "M2 Feedback" {
            n712 = Variant To Data(error in=w1653, type=u8 0 ("Network Data Down.M2 Commands.Feedback"), Variant=w1651) -> (data=w1649:u8, error out=w1650:errorcluster)
            n713 = call <vilib>:"Flatten To JSON String.vi"("error in (no error)"=w1650, "Variant"=w1649) -> ("error out"=w1647:errorcluster, "JSON String"=w1648:string)  [unwired: 8 in]
            n714 = Format Into String(w1649) -> (resulting string=w1646:string)  [unwired: 3 in, 1 out]
          }
          frame "M1 Package" {
            n715 = Variant To Data(error in=w1661, type=u16 0 ("Network Data Down.M1 Commands.Package"), Variant=w1659) -> (data=w1657:u16, error out=w1658:errorcluster)
            n716 = call <vilib>:"Flatten To JSON String.vi"("error in (no error)"=w1658, "Variant"=w1657) -> ("error out"=w1656:errorcluster, "JSON String"=w1655:string)  [unwired: 8 in]
            n717 = Format Into String(w1657) -> (resulting string=w1654:string)  [unwired: 3 in, 1 out]
          }
          frame "M2 Package" {
            n718 = Variant To Data(error in=w1669, type=u16 0 ("Network Data Down.M2 Commands.Package"), Variant=w1667) -> (data=w1665:u16, error out=w1666:errorcluster)
            n719 = call <vilib>:"Flatten To JSON String.vi"("error in (no error)"=w1666, "Variant"=w1665) -> ("error out"=w1664:errorcluster, "JSON String"=w1663:string)  [unwired: 8 in]
            n720 = Format Into String(w1665) -> (resulting string=w1662:string)  [unwired: 3 in, 1 out]
          }
          frame "M1 Enable" {
            n721 = Variant To Data(error in=w1676, type=TRUE, Variant=w1674) -> (data=w1672:bool, error out=w1670:errorcluster)
            n722 = call <vilib>:"Flatten To JSON String.vi"("error in (no error)"=w1670, "Variant"=w1672) -> ("error out"=w1675:errorcluster, "JSON String"=w1673:string)  [unwired: 8 in]
          }
          frame "M2 Enable" {
            n723 = Variant To Data(error in=w1683, type=TRUE, Variant=w1682) -> (data=w1679:bool, error out=w1677:errorcluster)
            n724 = call <vilib>:"Flatten To JSON String.vi"("error in (no error)"=w1677, "Variant"=w1679) -> ("error out"=w1681:errorcluster, "JSON String"=w1680:string)  [unwired: 8 in]
          }
          frame "Update Config" {
            w1689 = T36 {"Packages"={"DUT Force lbf"={" 0"=0, " 1"=0, " 2"=0, "3"=0, "4"=0, "5"=0, " 6"=0, "7"=0, "8"=0, "9"=0}, "DUT Names"={"0"="", "1"="", "2"="", "3"="", "4"="", "5"="", "6"="", "7"="", "8"="", "9"=""}}, "Heater PID"={"P"=0.0, "I"=0.0, "D"=0.0}, "Piston Settings"={"Forces Slope"=0.0, "Forces Intercept"=0.0, "Transition Force"=0.0, "Up Force"=0.0, "Diameter (mm)"=0.0, "Delay (ms)"=0.0, "Pressure Ramp Delay (ms)"=0.0}, "Safe Temps"={"Minimum"=17, "Enabled"=TRUE, "Maximum"=95}, "System Settings"={"Number of Heads"=0, "60Hz Power"=TRUE, "FTC200"=TRUE, "AutoStartup"=FALSE, "Purge"=TRUE, "Sensors"=TRUE, "HandClamp"=TRUE, "ATE"=TRUE, "Benchtop"=TRUE, "Production"=TRUE, "Refrigerant"=0, "Handler"=TRUE, "Shuttle"=TRUE, "220V"=FALSE, "Cascade"=FALSE, "Suction Sensor"=0, "Discharge Sensor"=0}, "Stepper Settings "={"Microstepping"=0, "Velocity"=8}, "Set Point Range"={"Max"=0.0, "Min"=0.0}, "Pedestal Check DeltaT"=0.0, "Ramp Delta T"=0.0, "Ramp-SS Threshold"=0.0, "SS Tolerance"=0.0, "EEV PID"={"Ramp Up Target"=0.0, "Ramp Down Target"=0.0, "Steady State Target"=0.0, "Output"={"Max"=0.0, "Min"=0.0}, "EBB and Flow Temp TH"=0.0, "Cryomode EEV Max"=0.0, "Valve minimum opening "=0.0, "Ramp Up EEV Steps"=0.0, "Ramp Down EEV Steps"=0.0, "SS EEV Steps Reset"=0.0, "EBB and Flow Tol"=0.0, "Gains"={"P"=0.0, "I"=0.0, "D"=0.0}, "Dissabled Target"=0.0, "CryoMode Gains"={"P"=0.0, "I"=0.0, "D"=0.0}, "M1 SuperHeat Setpoint"=0.0, "M2 Gains"={"P"=0.0, "I"=0.0, "D"=0.0}, "Flow Curve"=0}, "Sleep Timeout"=0.0, "Bypass Values"={"Bypass Valve"=TRUE, "Flow Curve"=0, "Output"={"Max"=0, "Min"=0}, "Feedback"=0, "Cyth Bypass"=TRUE, "PID"={"P"=0.0, "I"=0.0, "D"=0.0}, "Pressure setpoint"=0, "Cryo Temp"=0, "Superheat Setpoint"=0, "Cryo Setpoint"=0}, "Default Temp"=0.0, "InTEC"={"Enabled"=FALSE, "IP"="192.168.1.100", "Port"=5000}, "M1 TSD"={"Gain"=0.0, "Offset"=0.0, "V Offset "=0.0}, "M2 TSD"={"Gain"=0.0, "Offset"=0.0, "V Offset "=0.0}, "M1 T-Case Calibration"={"Gain"=0.0, "Offset"=0.0}, "M2 T-Case Calibration"={"Gain"=0.0, "Offset"=0.0}, "Heater PID TSD"={"P"=0.0, "I"=0.0, "D"=0.0}, "M2 Heater PID"={"P"=0.0, "I"=0.0, "D"=0.0}}  # Config Data
            n725 = Variant To Data(error in=w1690, type=w1689, Variant=w1688) -> (data=w1687:T36, error out=w1686:errorcluster)
            n726 = call <vilib>:"Flatten To JSON String.vi"("error in (no error)"=w1686, "Variant"=w1687) -> ("error out"=w1685:errorcluster, "JSON String"=w1684:string)  [unwired: 8 in]
          }
          frame "Reboot RT" {
            n727 = Variant To Data(error in=w1697, type=TRUE ("Stop RT"), Variant=w1696) -> (data=w1693:bool, error out=w1691:errorcluster)
            n728 = call <vilib>:"Flatten To JSON String.vi"("error in (no error)"=w1691, "Variant"=w1693) -> ("error out"=w1695:errorcluster, "JSON String"=w1694:string)  [unwired: 8 in]
          }
          frame "Stop RT" {
            n729 = Variant To Data(error in=w1704, type=TRUE ("STop RT"), Variant=w1703) -> (data=w1698:bool, error out=w1701:errorcluster)
            n730 = call <vilib>:"Flatten To JSON String.vi"("error in (no error)"=w1701, "Variant"=w1698) -> ("error out"=w1700:errorcluster, "JSON String"=w1699:string)  [unwired: 8 in]
          }
        }
        n731 = Unbundle By Name(w1596) -> ("TCP connection info"=w1595:T30)
        n732 = call-poly <vilib>:"Write Message.vi"("error in"=w1587, "data"=w1591, "name"=w1590, "connection info in"=w1595) -> ("error out"=w1597:errorcluster)  [unwired: 1 in, 6 out]
      }
      frame "TCP:Close Connection" {
        w1707 = 66 items=["No Error", "Argument Error", "Memory Full", "Out of Zone", "End of File", "File Already Open", "Generic File IO Error", "File Not Found", "File Permission Error", "Disk Full", "Duplicate Path", "Too Many Files Open", "Not Enabled", "Resource File Not Found", "Cannot Add Resource", "Resource Not Found", "Image Not Found", "Image Memory Error", "Pen Does Not Exist", "Config Bad Type", "Config Token Not Found", "Config Parse Error", "Config Memory Error", "Bad External Code Format", "Bad External Code Offset", "External Code Not Present", "Null Window", "Destroy Window Mixup", "Null Menu", "Print Aborted", "Bad Print Record", "Print Driver Error", "Windows Error During Print", "Memory Error During Print", "Print Dialog Error", "Generic Print Error", "Invalid Device Refnum", "Device Not Found", "Device Parameter Error", "Device Unit Error", "Can't Open Device", "Device Call Aborted", "Generic Error", "Cancelled By User", "Object ID Too Low", "Object ID Too High", "Object Not In Heap", "Unknown Heap", "Bad DefProc ID", "DefProc Not In Table", "Message Out Of Range", "Null Method", "Unknown Message", "Manager Call Not Supported", "Bad address", "Connection In progress", "Connection timed out", "Connection is already in progress", "Network attribute not supported", "Network error", "Address in use", "System out of memory", "Connection aborted", "Connection refused", "Connection is not connected", "Connection is already connected", "Connection closed", "Initialize error (interapplication manager)", "Bad occurrence", "Wait on unbound occurrence handler", "Occurrence queue overflow", "Bad path", "Semaphore not signaled", "Unrecognized type (interapplication manager)"] ("1st Error to Convert")
        n733 = Unbundle By Name(w1711) -> ("TCP connection info"=w1710:T30)
        n734 = call-poly <vilib>:"Get Connection Reference.vi"("error in"=w1712, "connection info in"=w1710) -> ("error out"=w1713:errorcluster, "connection ID out"=w1714:refnum<k5>)  [unwired: 8 out]
        n735 = TCP Close Connection(connection ID=w1714, error in (no error)=w1713) -> (error out=w1706:errorcluster)  [unwired: 2 out]
        n736 = call <vilib>:"Error to Warning.vi"("1st Error to Convert"=w1707, "error in"=w1706) -> ("warning out"=w1705:errorcluster)  [unwired: 3 in, 10 out]
      }
      frame "----------Database -----------" {
      }
      frame "DB:Login" {
        n737 = Variant To Data(error in=w1732, type=T46."Supervisor" ("f"), Variant=w1731) -> (data=w1720:T46, error out=w1718:errorcluster)
        n738 = case shown="\"Operator\", Default" w1720 {
          tunnel: [i32[] [0, 1, 2, 3, 4, 5] ("Page array") i32[] [0, 1, 2, 3] ("Page array") i32[] [0, 1, 2] ("Page array") i32[] [0, 1, 2] ("Page array")] -> w1722
          tunnel: [TRUE ("Visible") TRUE ("Visible") _ _] -> w1721
          tunnel: ["Supervisor" ("Command") "Engineer" ("Command") "Operator" ("Command") "Guest" ("Command")] -> w1719
          tunnel: w1718 -> [w1734 w1738 w1742 w1745]
          tunnel: [w1734 w1738 w1742 w1745] -> w1717
          frame "Supervisor" {
          }
          frame "Engineer" {
          }
          frame "Operator", Default {
          }
          frame "Guest" {
          }
        }
        n739 = To Variant(anything=w1722) -> (Variant=w1727:variant)
        n740 = call "Messaging EnQ Single.vi"("Command"="UI:Enable Tabs", "Data"=w1727, "error in (no error)"=w1717) -> ("error out"=w1725:errorcluster)  [unwired: 8 in]
        n741 = To Variant(anything=w1721) -> (Variant=w1723:variant)
        n742 = call "Messaging EnQ Single.vi"("Command"="UI:Enable Controls", "Data"=w1723, "error in (no error)"=w1725) -> ("error out"=w1733:errorcluster)  [unwired: 8 in]
        n743 = Bundle By Name(cluster=w1729, "Login"=w1721) -> (w1728:T27)
      }
      frame "DB:Event Logger" {
        # "5.12.2021 Johathan asked me to remove  saving the event logging to file"
        n744 = Variant To Data(error in=w1760, type=T21 {"Name"="", "Time Stamp"=timestamp(0 s since 1904-01-01), "Code"=0, "Source"="", "Value"="", "Boolean"=FALSE, "Description"="", "Error"=FALSE, "Warning"=FALSE, " Fault"=FALSE} ("Event"), Variant=w1759) -> (data=w1750:T21, error out=w1751:errorcluster)
        n745 = Unbundle By Name(w1761) -> ("Event Log"=w1762:T21[])
        n746 = call "Event Logger.vi"("Error In"=w1751, "Event"=w1750) -> ("Error Out"=w1748:errorcluster, "Event out"=w1749:T21)  [unwired: 8 in]
        n747 = Insert Into Array(array=w1762, new element=w1749) -> (w1757:T21[])  [unwired: 1 in]
        "GUI Events" <- w1757
        n748 = Bundle By Name(cluster=w1761, "Event Log"=w1757) -> (w1756:T27)
        n749 = Unbundle By Name(w1749) -> ("Description"=w1753:string)
        n750 = Unbundle By Name(w1756) -> ("Core.VI Name"=w1754:string)
        n751 = disable-structure shown="Disabled" {
          disable-tunnel: [w1768 w1769] -> w1755
          disable-tunnel: w1754 -> [w1766 _]
          disable-tunnel: w1753 -> [w1765 _]
          disable-tunnel: w1752 -> [w1764 _]
          disable-tunnel: w1748 -> [w1763 w1769]
          frame Disabled {
            n752 = call "Save Log FGV.vi"("Case"=w1764, "State"=Save_Log_State."Write", "Error In"=w1763, "Descripition"=w1765, "VI Name"=w1766) -> ("Error Out"=w1768:errorcluster)  [unwired: 6 in]
          }
          frame Enabled {
          }
        }
      }
      frame "----------- Application---------" {
      }
      frame "APP:Update Config" {
        # "Confirm Config Data modified"
        n753 = Unbundle By Name(w1780) -> ("Dataset.Config Data"=w1777:T36)
        n754 = Index Array(array=w1779) -> (element=w1778:string)  [unwired: 1 in]
        n755 = case shown="\"Package\"" w1778 {
          tunnel: w1777 -> [w1786 w1790]
          tunnel: [w1782 w1793] -> w1776
          tunnel: [w1783 w1792] -> w1775
          tunnel: [w1784 w1791] -> w1774
          tunnel: w1773 -> [w1788 w1789]
          frame "Package" {
            n756 = Unbundle By Name(w1786) -> ("Packages"=w1787:T54)
            n757 = call "Modified Packages.vi"("error in"=w1788, "Pagckages in"=w1787) -> ("error out"=w1782:errorcluster, "Cancel?"=w1783:bool, "Modified Packages"=w1785:T55)  [unwired: 6 in]
            n758 = Bundle By Name(cluster=w1786, "Packages"=w1785) -> (w1784:T36)
          }
          frame "Configure", Default {
            n759 = call "Update Config Data.vi"("error in (no error)"=w1789, "Config Data Current"=w1790) -> ("error out"=w1793:errorcluster, "Canceled"=w1792:bool, "Modified Config Data"=w1791:T36)  [unwired: 7 in]
          }
        }
        n760 = case shown="False" w1775 {
          tunnel: [w1796 w1798] -> w1781
          tunnel: w1776 -> [w1797 w1798]
          tunnel: w1774 -> [w1795 _]
          tunnel: "NS:Write>>Update Config" ("Command(s)") -> [w1794 _]
          frame False {
            n761 = call "Messaging EnQ Single.vi"("Command"=w1794, "Data"=w1795, "error in (no error)"=w1797) -> ("error out"=w1796:errorcluster)  [unwired: 8 in]
          }
          frame True {
          }
        }
      }
      frame "APP:Power Sequence(GUI)" {
        n762 = Unbundle By Name(w1799) -> ("Core.VI Path"=w1810:path)
        n763 = Strip Path(path=w1810) -> (stripped path=w1809:path)  [unwired: 1 out]
        n764 = Index Array(array=w1808) -> (element=w1807:string)  [unwired: 1 in]
        n765 = property on="Pattern File" class="CmbBox"(error in=w1804) -> (error out=w1803:errorcluster, "Value"=w1802:string)  [unwired: 1 in, 1 out]
        n766 = Build Path(base path=w1809, name or relative path="Power Pattern Configuration") -> (appended path=w1806:path)
        n767 = case shown="\"Delete Seq\"" w1807 {
          tunnel: w1806 -> [w1814 w1846 _ w1889 w1893 w1954 _]
          tunnel: w1805 -> [_ w1831 w1873 _ _ _ _]
          tunnel: w1803 -> [w1815 w1845 w1872 w1890 w1896 w1956 w1966]
          tunnel: w1802 -> [_ _ _ _ w1895 w1955 _]
          tunnel: [w1813 w1840 w1864 w1885 w1891 w1944 w1968] -> w1801
          tunnel: w1799 -> [w1812 w1834 w1860 w1886 w1892 w1949 w1973]
          tunnel: [w1812 w1833 w1859 w1886 w1892 w1948 w1972] -> w1800
          tunnel: w1799 -> [_ _ _ _ w1894 _ _]
          frame "Initialize" {
            n768 = call <vilib>:"Check if File or Folder Exists.vi"("error in (no error)"=w1815, "path"=w1814) -> ("error out"=w1820:errorcluster, "file or folder exists?"=w1822:bool, "dup path"=w1821:path)  [unwired: 7 in]
            n769 = case shown="False" w1822 {
              tunnel: w1821 -> [w1828 w1829]
              tunnel: w1820 -> [w1827 w1830]
              tunnel: [w1826 w1830] -> w1823
              tunnel: [w1825 w1829] -> w1824
              frame False {
                n770 = Create Folder(path (use dialog)=w1828, error in=w1827) -> (created path=w1825:path, error out=w1826:errorcluster)  [unwired: 1 in, 1 out]
              }
              frame True {
              }
            }
            n771 = List Folder(path=w1824, error in=w1823) -> (filenames=w1819:string[], error out=w1818:errorcluster)  [unwired: 2 in, 2 out]
            n772 = Index Array(array=w1819, index=0) -> (element=w1817:string)
            n773 = property on="Pattern File" class="CmbBox"(error in=w1818, "Strings[]"=w1819, "Val(Sgnl)"=w1817) -> (error out=w1813:errorcluster)  [unwired: 1 in, 1 out]
          }
          frame "Pattern File", Default {
            n774 = Variant To Data(error in=w1845, type="", Variant=w1831) -> (data=w1848:string, error out=w1842:errorcluster)
            n775 = Build Path(base path=w1846, name or relative path=w1848) -> (appended path=w1844:path)
            n776 = Empty String/Path?(string/path=w1848) -> (empty?=w1843:bool)
            n777 = case shown="False" w1843 {
              tunnel: [w1853 T25 [] ("Power Seq out")] -> w1832
              tunnel: [w1852 w1855] -> w1839
              tunnel: [T40."Enabled" ("Disabled") T40."Disabled and Grayed Out" ("Disabled")] -> w1835
              tunnel: w1842 -> [w1850 w1855]
              tunnel: w1844 -> [w1849 _]
              frame False {
                n778 = call "Config Power Sequence.vi"("Get/Update"=enum16{"Get Seq", "Update Seq"}."Get Seq", "Error In"=w1850, "Seq file path"=w1849) -> ("Error Out"=w1852:errorcluster, "Power Seq out"=w1853:T25)  [unwired: 6 in, 1 out]
              }
              frame True {
              }
            }
            n779 = property on="Power Seq" class="Arr (strict)"(error in=w1839, "Val(Sgnl)"=w1832) -> (error out=w1838:errorcluster)  [unwired: 1 in, 1 out]
            n780 = control-ref of="Save Seq"() -> (w1837:refnum<vi>)
            n781 = property class="Bool"(reference=w1837, error in=w1838, "DisabledEnum"=w1835) -> (error out=w1841:errorcluster)  [unwired: 1 out]
            n782 = control-ref of="Delete Seq"() -> (w1836:refnum<vi>)
            n783 = Bundle By Name(cluster=w1834, "TTV Test.Power Seq"=w1832) -> (w1833:T27)
            n784 = property class="Bool"(reference=w1836, error in=w1841, "DisabledEnum"=w1835) -> (error out=w1840:errorcluster)  [unwired: 1 out]
          }
          frame "Power Sequence" {
            n785 = Variant To Data(error in=w1872, type=cluster{"Iteration No":i32, "Power Seq":T25} {"Iteration No"=0, "Power Seq"=[]} ("output cluster"), Variant=w1873) -> (data=w1875:cluster{"Iteration No":i32, "Power Seq":T25}, error out=w1877:errorcluster)
            n786 = Unbundle By Name(w1875) -> ("Iteration No"=w1876:i32, "Power Seq"=w1878:T25)
            n787 = Variant To Data(error in=w1877, type=T25 [] ("Power Seq out"), Variant=w1878) -> (data=w1858:T25, error out=w1870:errorcluster)
            n788 = Less Than 0?(x=w1876) -> (x < 0?=w1874:bool)
            n789 = case shown="False" w1874 {
              tunnel: ["" "Infinite Cycle" ("Command")] -> w1871
              tunnel: w1876 -> [w1881 _]
              tunnel: [w1881 1 ("Plot.Plot Interpolation")] -> w1869
              frame False {
              }
              frame True {
              }
            }
            "Infinite Test" <- w1871
            n790 = property on="Test Graph" class="WFChart (strict)"("History Data"=dbl[] [], "Plot.Plot Interpolation"=u8 3) -> ()  [unwired: 2 in, 2 out]
            n791 = call "Set Seqence.vi"("Error In"=w1870, "Iteration"=w1869, "Power Seq"=w1858) -> ("Error Out"=w1865:errorcluster, "Waveform Graph"=w1867:u32[])  [unwired: 7 in]
            n792 = To Double Precision Float(number=w1867) -> (double precision float=→"Test Graph":dbl[])
            n793 = control-ref of="Save Seq"() -> (w1863:refnum<vi>)
            n794 = Bundle By Name(cluster=w1860, "TTV Test.Power Seq"=w1858) -> (w1859:T27)
            n795 = property class="Bool"(reference=w1863, error in=w1865, "DisabledEnum"=T40."Enabled" ("Disabled")) -> (error out=w1864:errorcluster)  [unwired: 1 out]
          }
          frame "Refresh Seq" {
            n796 = List Folder(path=w1889, error in=w1890) -> (filenames=w1887:string[], error out=w1888:errorcluster)  [unwired: 2 in, 2 out]
            n797 = property on="Pattern File" class="CmbBox"(error in=w1888, "Strings[]"=w1887) -> (error out=w1885:errorcluster)  [unwired: 1 in, 1 out]
          }
          frame "Save Seq" {
            n798 = Unbundle By Name(w1894) -> ("TTV Test.Power Seq"=w1903:T25)
            n799 = Format Into String(format string="Overwrite it to %s", w1895) -> (resulting string=w1897:string)  [unwired: 2 in, 1 out]
            n800 = call <vilib>:"Three Button Dialog.vi"("Window Title (\"\")"="Save file (.ini)" ("Window Title (\"\")"), "Center Button Text (\"No\")"="Save as" ("Center Button Text (\"No\")"), "message"=w1897) -> ("Which Button?"=w1901:T56)  [unwired: 8 in]
            n801 = case shown="\"Center Button\"" w1901 {
              tunnel: "Enter the filename(.ini)" ("Message title") -> [_ w1932 _ _]
              tunnel: w1893 -> [w1912 w1924 _ _]
              tunnel: w1896 -> [w1909 w1926 w1942 w1943]
              tunnel: [w1905 w1922 w1942 w1943] -> w1891
              tunnel: w1895 -> [w1911 _ _ _]
              tunnel: w1903 -> [w1904 w1921 _ _]
              frame "Left Button", Default {
                n802 = Build Path(base path=w1912, name or relative path=w1911) -> (appended path=w1910:path)
                n803 = Empty String/Path?(string/path=w1911) -> (empty?=w1913:bool)
                n804 = case shown="False" w1913 {
                  tunnel: w1910 -> [w1917 w1918]
                  tunnel: w1909 -> [w1916 w1919]
                  tunnel: [w1915 w1918] -> w1906
                  tunnel: [w1914 w1919] -> w1907
                  frame False {
                    n805 = Delete(path (use dialog)=w1917, error in=w1916) -> (deleted path=w1915:path, error out=w1914:errorcluster)  [unwired: 3 in, 1 out]
                  }
                  frame True {
                  }
                }
                n806 = call "Config Power Sequence.vi"("Get/Update"=enum16{"Get Seq", "Update Seq"}."Update Seq", "Error In"=w1907, "Power Seq"=w1904, "Seq file path"=w1906) -> ("Error Out"=w1905:errorcluster)  [unwired: 5 in, 2 out]
              }
              frame "Center Button" {
                w1929 = ".ini" ("regular expression")
                n807 = call "User Input Dialog.vi"("Message title"=w1932) -> ("OK?"=w1928:bool, "Message out"=w1925:string)  [unwired: 7 in, 1 out]
                n808 = Match Pattern(string=w1925, regular expression=w1929) -> (match substring=w1931:string)  [unwired: 1 in, 3 out]
                n809 = Build Path(base path=w1924, name or relative path=w1925) -> (appended path=w1923:path)
                n810 = Equal?(x=w1931, y=w1929) -> (x = y?=w1930:bool)
                n811 = And(x=w1928, y=w1930) -> (x .and. y?=w1927:bool)
                n812 = case shown="True" w1927 {
                  tunnel: w1923 -> [_ w1941]
                  tunnel: w1926 -> [w1933 w1940]
                  tunnel: [w1933 w1934] -> w1922
                  tunnel: w1921 -> [_ w1938]
                  tunnel: enum16{"Get Seq", "Update Seq"}."Update Seq" ("Get/Update") -> [_ w1937]
                  frame False {
                  }
                  frame True {
                    n813 = call "Config Power Sequence.vi"("Get/Update"=w1937, "Error In"=w1940, "Power Seq"=w1938, "Seq file path"=w1941) -> ("Error Out"=w1935:errorcluster, "Seq path out"=w1939:path)  [unwired: 5 in, 1 out]
                    n814 = Strip Path(path=w1939) -> (name=w1936:string)  [unwired: 1 out]
                    n815 = property on="Pattern File" class="CmbBox"(error in=w1935, "Value"=w1936) -> (error out=w1934:errorcluster)  [unwired: 1 in, 1 out]
                  }
                }
              }
              frame "Right Button" {
              }
              frame "Window Close" {
              }
            }
          }
          frame "Delete Seq" {
            w1947 = T25 [] ("Power Seq out")
            n816 = Build Path(base path=w1954, name or relative path=w1955) -> (appended path=w1958:path)
            n817 = Delete(path (use dialog)=w1958, confirm (F)=TRUE, error in=w1956) -> (deleted path=w1960:path, error out=w1959:errorcluster)  [unwired: 2 in, 1 out]
            n818 = Strip Path(path=w1960) -> (stripped path=w1961:path)  [unwired: 1 out]
            n819 = List Folder(path=w1961, error in=w1959) -> (filenames=w1952:string[], error out=w1953:errorcluster)  [unwired: 2 in, 2 out]
            n820 = property on="Pattern File" class="CmbBox"(error in=w1953, "Strings[]"=w1952, "Value"="") -> (error out=w1950:errorcluster)  [unwired: 1 in, 1 out]
            n821 = property on="Power Seq" class="Arr (strict)"(error in=w1950, "Val(Sgnl)"=w1947) -> (error out=w1945:errorcluster)  [unwired: 1 in, 1 out]
            n822 = Bundle By Name(cluster=w1949, "TTV Test.Power Seq"=w1947) -> (w1948:T27)
            n823 = property on="Test Graph" class="WFChart (strict)"(error in=w1945, "History Data"=dbl[] [] ("Power Pattern Graph")) -> (error out=w1944:errorcluster)  [unwired: 1 in, 1 out]
          }
          frame "Clear Seq" {
            w1967 = T40."Disabled and Grayed Out" ("Disabled")
            w1971 = T25 [] ("Power Seq out")
            n824 = control-ref of="Save Seq"() -> (w1962:refnum<vi>)
            n825 = property class="Bool"(reference=w1962, error in=w1966, "DisabledEnum"=w1967) -> (error out=w1965:errorcluster)  [unwired: 1 out]
            n826 = control-ref of="Delete Seq"() -> (w1963:refnum<vi>)
            n827 = property class="Bool"(reference=w1963, error in=w1965, "DisabledEnum"=w1967) -> (error out=w1964:errorcluster)  [unwired: 1 out]
            n828 = property on="Pattern File" class="CmbBox"(error in=w1964, "Value"="") -> (error out=w1974:errorcluster)  [unwired: 1 in, 1 out]
            n829 = property on="Power Seq" class="Arr (strict)"(error in=w1974, "Val(Sgnl)"=w1971) -> (error out=w1969:errorcluster)  [unwired: 1 in, 1 out]
            n830 = Bundle By Name(cluster=w1973, "TTV Test.Power Seq"=w1971) -> (w1972:T27)
            n831 = property on="Test Graph" class="WFChart (strict)"(error in=w1969, "History Data"=dbl[] [] ("Power Pattern Graph")) -> (error out=w1968:errorcluster)  [unwired: 1 in, 1 out]
          }
        }
      }
      frame "APP:TTV Test" {
        # "Control the power on/off and voltage to Chroma AC Power Supply"
        n832 = Index Array(array=w1983) -> (element=w1982:string)  [unwired: 1 in]
        n833 = case shown="\"Stop Test\"" w1982 {
          tunnel: w1981 -> [w2012 w2055 w2165 w2181 w2195 w2295]
          tunnel: w1980 -> [w2011 _ _ _ _ _]
          tunnel: [w1988 w2062 w2153 w2170 w2191 w2294] -> w1979
          tunnel: w1977 -> [w2008 w2067 w2150 w2179 w2193 w2293]
          tunnel: [w2006 w2066 w2149 w2178 w2192 w2293] -> w1978
          tunnel: w1977 -> [_ w2075 w2158 _ w2194 _]
          tunnel: w1976 -> [w1987 w2054 _ w2168 _ _]
          frame "Power", Default {
            w2003 = 1 ("Current Cycle")
            n834 = Variant To Data(error in=w2012, type=FALSE ("Output"), Variant=w2011) -> (data=w2009:bool, error out=w2010:errorcluster)
            n835 = case shown="True" w2009 {
              tunnel: [w2018 w2038] -> w1989
              tunnel: w2010 -> [w2024 w2033]
              tunnel: [FALSE w2039] -> w2007
              tunnel: [T40."Disabled and Grayed Out" ("Disabled") T40."Enabled" ("Disabled")] -> w2002
              tunnel: [T40."Enabled" ("Disabled") T40."Disabled and Grayed Out" ("Disabled")] -> w1994
              tunnel: [w2019 w2032] -> w1986
              tunnel: w1987 -> [w2019 w2032]
              tunnel: [FALSE ("Boolean") TRUE ("Boolean")] -> w1985
              tunnel: ["PS off" ("Description") "PS on" ("Description")] -> w1984
              frame False {
                # "Power off to disconnect PS and switch the mode to edit the power sequence"
                n836 = call "Serial FGV.vi"("Status"=enum16{"Config", "Read", "Write", "Close"}."Write", "Error In"=w2024, "Command"="OUTPUT OFF\n") -> ("Error Out"=w2027:errorcluster)  [unwired: 5 in, 3 out]
                n837 = call "Serial FGV.vi"("Status"=enum16{"Config", "Read", "Write", "Close"}."Close", "Error In"=w2027) -> ("Error Out"=w2018:errorcluster)  [unwired: 6 in, 3 out]
                n838 = property on="Test Graph" class="WFChart (strict)"("History Data"=dbl[] [], "Plot.Plot Interpolation"=u8 3) -> ()  [unwired: 2 in, 2 out]
              }
              frame True {
                w2034 = u16 19200 items=["4800"=4800, "9600"=9600, "19200"=19200, "38400"=38400, "57600"=57600] ("Baud Rate")
                # "Power on and check out the system error"
                n839 = local read "Serial Port"() -> (w2037:string)
                n840 = To Unsigned Long Integer(number=w2034) -> (unsigned 32bit integer=w2052:u32)
                n841 = Bundle By Name(cluster=T47 {"baud rate"=19200, "data bits"=8, "parity"=enum."None", "stop bits"=10, "flow control"=0} ("Serial Settings"), "baud rate"=w2052) -> (w2051:T47)
                n842 = Type Cast(type=refnum<visa-resource-name> refnum ("VISA resource name"), x=w2037) -> (*(type *) &x=w2050:refnum<visa-resource-name>)
                n843 = call "Serial FGV.vi"("Status"=enum16{"Config", "Read", "Write", "Close"}."Config", "Error In"=w2033, "Serial Settings"=w2051, "VISA resource name"=w2050) -> ("Error Out"=w2047:errorcluster)  [unwired: 4 in, 3 out]
                n844 = call "Serial FGV.vi"("Status"=enum16{"Config", "Read", "Write", "Close"}."Write", "Error In"=w2047, "Command"="SYSTEM:ERROR?\n") -> ("Error Out"=w2043:errorcluster)  [unwired: 5 in, 3 out]
                n845 = call "Serial FGV.vi"("delay before read (ms)"=u32 10, "Status"=enum16{"Config", "Read", "Write", "Close"}."Read", "Error In"=w2043) -> ("Error Out"=w2038:errorcluster, "Response"=w2041:string)  [unwired: 5 in, 2 out]
                n846 = Equal?(x="NO", y=w2041) -> (x = y?=w2039:bool)
              }
            }
            n847 = Bundle By Name(cluster=T21 {"Name"="", "Time Stamp"=timestamp(0 s since 1904-01-01), "Code"=0, "Source"="", "Value"="", "Boolean"=FALSE, "Description"="", "Error"=FALSE, "Warning"=FALSE, " Fault"=FALSE} ("Event"), "Boolean"=w1985, "Description"=w1984, "Name"=w1986) -> (w1993:T21)
            n848 = To Variant(anything=w1993) -> (Variant=w1992:variant)
            n849 = call "Messaging EnQ Single.vi"("Command"="DB:Event Logger", "Data"=w1992, "error in (no error)"=w1989) -> ("error out"=w1988:errorcluster)  [unwired: 8 in]
            n850 = control-ref of="Pattern File"() -> (w2001:refnum<vi>)
            n851 = control-ref of="Seq Controls"() -> (w1999:refnum<vi>)
            n852 = control-ref of="Iteration No"() -> (w1998:refnum<vi>)
            n853 = control-ref of="Menu Ring"() -> (w1997:refnum<vi>)
            n854 = control-ref of="Power Seq"() -> (w2000:refnum<vi>)
            n855 = control-ref of="Manual IP"() -> (w1996:refnum<vi>)
            n856 = property on="Time" class="DigNum (strict)"("Value"=0.0 ("Time")) -> ()  [unwired: 2 in, 2 out]
            n857 = Build Array(w2001, w2000, w1999, w1998, w1997, w1996) -> (w1995:refnum<vi>[])
            n858 = Bundle By Name(cluster=w2008, "TTV Test.Current Cycle"=w2003, "TTV Test.Step"=0 ("Step"), "TTV Test.PS Connection"=w2007) -> (w2006:T27)
            n859 = property on="Cycle" class="DigNum (strict)"("Value"=w2003) -> ()  [unwired: 2 in, 2 out]
            n860 = for {
              tunnel: w1995 -> [w2015] mode=indexing
              tunnel: w1994 -> [w2014]
              n861 = property class="Ctl"(reference=w2015, "DisabledEnum"=w2014) -> ()  [unwired: 1 in, 2 out]
            }
            n862 = property on="Start Test" class="Bool"("DisabledEnum"=w2002) -> ()  [unwired: 2 in, 2 out]
            n863 = property on="Reset Test" class="Bool"("DisabledEnum"=w2002) -> ()  [unwired: 2 in, 2 out]
            n864 = property on="Stop Test" class="Bool"("DisabledEnum"=w2002) -> ()  [unwired: 2 in, 2 out]
          }
          frame "Start Test" {
            n865 = Unbundle By Name(w2075) -> ("TTV Test.Current Cycle"=w2068:i32, "TTV Test.Step"=w2069:i32, "TTV Test.Power Seq"=w2070:T25, "TTV Test.PS Connection"=w2074:bool)
            n866 = local read "Iteration No"() -> (w2073:i32)
            n867 = Not Equal To 0?(x=w2073) -> (x != 0?=w2072:bool)
            n868 = Compound Arithmetic op=AND(w2074, w2072) -> ()  [unwired: 1 out]
            n869 = case shown="False" TRUE {
              tunnel: w2070 -> [_ w2132]
              tunnel: w2069 -> [w2083 w2133]
              tunnel: w2068 -> [w2082 w2134]
              tunnel: [FALSE TRUE] -> w2065
              tunnel: [w2085 w2120] -> w2063
              tunnel: [FALSE TRUE] -> w2061
              tunnel: [w2087 w2118] -> w2060
              tunnel: [w2083 w2116] -> w2059
              tunnel: [w2082 w2115] -> w2058
              tunnel: w2055 -> [w2095 w2111]
              tunnel: [T40."Enabled" ("Disabled") T40."Disabled and Grayed Out" ("Disabled")] -> w2056
              tunnel: [T40."Disabled and Grayed Out" ("Disabled") T40."Enabled" ("Disabled")] -> w2057
              tunnel: w2054 -> [_ w2100]
              frame False {
                # "Set up Time out"
                # "Try to connect to the power supply until the boot time set up"
                n870 = property on="Boot Time(s)" class="DigNum (strict)"(error in=w2095) -> (error out=w2085:errorcluster, "Value"=w2093:u32)  [unwired: 1 in, 1 out]
                n871 = Increment(x=w2093) -> (x+1=w2094:u32)
                "Boot Time(s)" <- w2094
                n872 = Greater Or Equal?(x=w2094, y="Boot Time out(s)") -> (x >= y?=w2088:bool)
                n873 = Wait (ms)(milliseconds to wait=u32 1000) -> ()  [unwired: 1 out]
                n874 = Select(t="Stop Test" ("Command"), s=w2088, f="Start Test" ("Command")) -> (s? t:f=w2092:string)
                n875 = Concatenate Strings("APP:TTV Test>>" ("Command"), w2092) -> (w2087:string)
              }
              frame True {
                n876 = First Call?() -> (First Call?: T/F=w2135:bool)
                n877 = case shown="False" w2135 {
                  tunnel: [T48."Resume" ("Timer Mode") T48."Start Timer" ("Timer Mode")] -> w2106
                  tunnel: w2133 -> [w2138 _]
                  tunnel: w2132 -> [w2140 w2145]
                  tunnel: [w2139 w2144] -> w2131
                  tunnel: [w2138 w2143] -> w2116
                  tunnel: w2134 -> [w2137 _]
                  tunnel: [w2137 1 ("Current Cycle")] -> w2115
                  frame False {
                    n878 = Index Array(array=w2140, index=w2138) -> (element=w2139:T57)
                  }
                  frame True {
                    w2143 = 0 ("Step No")
                    n879 = Index Array(array=w2145, index=w2143) -> (element=w2144:T57)
                  }
                }
                n880 = property on="Test Graph" class="WFChart (strict)"(error in=w2111, "History Data"=dbl[] [], "Plot.Plot Interpolation"=u8 2) -> (error out=w2112:errorcluster)  [unwired: 1 in, 1 out]
                n881 = Unbundle By Name(w2131) -> ("Name"=→"Step":string, "Head Load(W)"=w2125:u32, "Duration"=w2105:i32)
                n882 = call "Timing FGV.vi"("Time Target (s)"=w2105, "Timer Mode"=w2106, "Error In"=w2112) -> ("Error Out"=w2117:errorcluster)  [unwired: 6 in, 2 out]
                n883 = Bundle By Name(cluster=T21 {"Name"="", "Time Stamp"=timestamp(0 s since 1904-01-01), "Code"=0, "Source"="", "Value"="", "Boolean"=FALSE, "Description"="", "Error"=FALSE, "Warning"=FALSE, " Fault"=FALSE} ("Event"), "Boolean"=TRUE, "Description"="Start TTV Test", "Name"=w2100) -> (w2104:T21)
                n884 = To Variant(anything=w2104) -> (Variant=w2103:variant)
                n885 = call "Messaging EnQ Single.vi"("Command"="DB:Event Logger", "Data"=w2103) -> ()  [unwired: 9 in, 1 out]
                n886 = Number To Fractional String(number=w2125, precision (6)=3) -> (F-format string=w2127:string)  [unwired: 1 in, 1 out]
                n887 = Concatenate Strings("VOLTAGE:AC " ("Command"), w2127, "\n" ("Command"), "OUTPUT ON\n" ("Command")) -> (w2107:string)
                n888 = call "Serial FGV.vi"("Status"=enum16{"Config", "Read", "Write", "Close"}."Write", "Error In"=w2117, "Command"=w2107) -> ("Error Out"=w2120:errorcluster)  [unwired: 5 in, 3 out]
                n889 = Concatenate Strings("NS:Write>>" ("Command"), "TTV Test" ("Command")) -> (w2118:string)
              }
            }
            n890 = Bundle By Name(cluster=w2067, "TTV Test.Current Cycle"=w2058, "TTV Test.Step"=w2059, "TTV Test.OutputState"=w2065) -> (w2066:T27)
            n891 = To Variant(anything=w2061) -> (Variant=w2064:variant)
            n892 = property on="Start Test" class="Bool"("DisabledEnum"=w2056) -> ()  [unwired: 2 in, 2 out]
            n893 = property on="Reset Test" class="Bool"("DisabledEnum"=w2056) -> ()  [unwired: 2 in, 2 out]
            n894 = property on="Stop Test" class="Bool"("DisabledEnum"=w2057) -> ()  [unwired: 2 in, 2 out]
            n895 = disable-structure shown="Disabled" {
              disable-tunnel: w2064 -> [w2079 _]
              disable-tunnel: w2063 -> [w2078 _]
              disable-tunnel: [w2077 _] -> w2062
              disable-tunnel: w2060 -> [w2076 _]
              frame Disabled {
                n896 = call "Messaging EnQ Single.vi"("Command"=w2076, "Data"=w2079, "error in (no error)"=w2078) -> ("error out"=w2077:errorcluster)  [unwired: 8 in]
              }
              frame Enabled {
              }
            }
          }
          frame "Reset Test" {
            n897 = property on="Cycle" class="DigNum (strict)"(error in=w2165, "Value"=1 ("Cycle")) -> (error out=w2148:errorcluster)  [unwired: 1 in, 1 out]
            n898 = property on="Step" class="Str"(error in=w2148, "Value"="") -> (error out=w2161:errorcluster)  [unwired: 1 in, 1 out]
            n899 = property on="Time" class="DigNum (strict)"(error in=w2161, "Value"=0.0 ("Time")) -> (error out=w2159:errorcluster)  [unwired: 1 in, 1 out]
            n900 = Unbundle By Name(w2158) -> ("TTV Test.Power Seq"=w2154:T25)
            n901 = property on="Test Graph" class="WFChart (strict)"(error in=w2159, "History Data"=dbl[] []) -> (error out=w2155:errorcluster)  [unwired: 1 in, 1 out]
            n902 = Index Array(array=w2154, index=0) -> (element=w2156:T57)
            n903 = Unbundle By Name(w2156) -> ("Duration"=w2146:i32)
            n904 = call "Timing FGV.vi"("Time Target (s)"=w2146, "Timer Mode"=T48."Start Timer", "Error In"=w2155) -> ("Error Out"=w2153:errorcluster)  [unwired: 6 in, 2 out]
            n905 = Bundle By Name(cluster=w2150, "TTV Test.Current Cycle"=1 ("Current Cycle"), "TTV Test.Step"=0 ("Step")) -> (w2149:T27)
          }
          frame "Stop Test" {
            w2177 = T40."Enabled" ("Disabled")
            n906 = call "Serial FGV.vi"("Status"=enum16{"Config", "Read", "Write", "Close"}."Write", "Error In"=w2181, "Command"="OUTPUT OFF\n") -> ("Error Out"=w2182:errorcluster)  [unwired: 5 in, 3 out]
            n907 = To Variant(anything=FALSE ("Start Stop Test")) -> (Variant=w2187:variant)
            n908 = call "Messaging EnQ Single.vi"("Command"="NS:Write>>TTV Test", "Data"=w2187, "error in (no error)"=w2182) -> ("error out"=w2188:errorcluster)  [unwired: 8 in]
            n909 = call "Timing FGV.vi"("Timer Mode"=T48."Pause", "Error In"=w2188) -> ("Error Out"=w2171:errorcluster)  [unwired: 7 in, 2 out]
            n910 = Bundle By Name(cluster=T21 {"Name"="", "Time Stamp"=timestamp(0 s since 1904-01-01), "Code"=0, "Source"="", "Value"="", "Boolean"=FALSE, "Description"="", "Error"=FALSE, "Warning"=FALSE, " Fault"=FALSE} ("Event"), "Boolean"=FALSE, "Description"="Stop TTV Test", "Name"=w2168) -> (w2175:T21)
            n911 = To Variant(anything=w2175) -> (Variant=w2174:variant)
            n912 = call "Messaging EnQ Single.vi"("Command"="DB:Event Logger", "Data"=w2174, "error in (no error)"=w2171) -> ("error out"=w2170:errorcluster)  [unwired: 8 in]
            n913 = Bundle By Name(cluster=w2179, "TTV Test.OutputState"=FALSE ("Start Stop Test")) -> (w2178:T27)
            n914 = property on="Start Test" class="Bool"("DisabledEnum"=w2177) -> ()  [unwired: 2 in, 2 out]
            n915 = property on="Reset Test" class="Bool"("DisabledEnum"=w2177) -> ()  [unwired: 2 in, 2 out]
            n916 = property on="Stop Test" class="Bool"("DisabledEnum"=T40."Disabled and Grayed Out" ("Disabled")) -> ()  [unwired: 2 in, 2 out]
          }
          frame "Read TTV power" {
            n917 = Unbundle By Name(w2194) -> ("TTV Test.Step"=w2203:i32, "TTV Test.Power Seq"=w2201:T25, "TTV Test.Current Cycle"=w2204:i32)
            n918 = call "Timing FGV.vi"("Timer Mode"=T48."Read Time", "Error In"=w2195) -> ("Error Out"=w2197:errorcluster, "Elapsed Time (s.ms)"=w2200:dbl, "Has Time Elapsed"=w2196:bool)  [unwired: 7 in]
            n919 = case shown="True" w2196 {
              tunnel: [w2209 w2239] -> w2202
              tunnel: w2197 -> [w2212 w2238]
              tunnel: [w2221 w2238] -> w2198
              tunnel: [TRUE w2243] -> w2199
              tunnel: w2200 -> [w2207 _]
              tunnel: w2201 -> [_ w2242]
              tunnel: w2203 -> [w2209 w2240]
              tunnel: w2204 -> [w2210 w2237]
              tunnel: [w2210 w2244] -> w2190
              frame False {
                # "timing equation : \n\nidle    delay   read  \n100 +  250 + 640+10 = 1000 ( one second)"
                # "Then, make timing a second"
                # "Make sure the connection"
                # "Time delay = 250 ms"
                # "Read power from the power supply"
                n920 = disable-structure shown="Enabled" {
                  disable-tunnel: [w2227 _] -> w2206
                  frame Enabled {
                    # "Create signal simulated"
                    n921 = for {
                      N: 1 -> [_]
                      tunnel: [w2230] -> w2227
                      n922 = Random Number (0-1)() -> (number: 0 to 1=w2232:dbl)
                      n923 = Multiply(x=w2232, y=100.0) -> (x*y=w2230:dbl)
                      n924 = Wait (ms)(milliseconds to wait=u32 1) -> ()  [unwired: 1 out]
                    }
                  }
                  frame Disabled {
                  }
                }
                n925 = call "Serial FGV.vi"("Status"=enum16{"Config", "Read", "Write", "Close"}."Write", "Error In"=w2212, "Command"="FETCH:POWER:AC:APPARENT?\n") -> ("Error Out"=w2218:errorcluster)  [unwired: 5 in, 3 out]
                n926 = call "Serial FGV.vi"("delay before read (ms)"=u32 640, "Status"=enum16{"Config", "Read", "Write", "Close"}."Read", "Error In"=w2218) -> ("Error Out"=w2211:errorcluster, "Response"=w2217:string)  [unwired: 5 in, 2 out]
                n927 = Fract/Exp String To Number(string=w2217) -> ()  [unwired: 3 in, 2 out]
                n928 = Build Array(w2206) -> (w2205:dbl[])
                n929 = property on="Test Graph" class="WFChart (strict)"("History Data"=w2205) -> ()  [unwired: 2 in, 2 out]
                n930 = call "Serial FGV.vi"("Status"=enum16{"Config", "Read", "Write", "Close"}."Write", "Error In"=w2211, "Command"="OUTPUT?\n") -> ("Error Out"=w2226:errorcluster)  [unwired: 5 in, 3 out]
                n931 = call "Serial FGV.vi"("delay before read (ms)"=u32 10, "Status"=enum16{"Config", "Read", "Write", "Close"}."Read", "Error In"=w2226) -> ("Error Out"=w2221:errorcluster, "Response"=w2225:string)  [unwired: 5 in, 2 out]
                n932 = Equal?(x="ON" ("Command"), y=w2225) -> ()  [unwired: 1 out]
                "Time" <- w2207
              }
              frame True {
                # "When done for a step, check out if the current step reach out the end of step and iteration"
                n933 = local read "Iteration No"() -> (w2235:i32)
                n934 = Array Size(array=w2242) -> (size(s)=w2246:i32)
                n935 = Greater Or Equal?(x=w2237, y=w2235) -> (x >= y?=w2236:bool)
                n936 = Equal?(x=w2240, y=w2246) -> (x = y?=w2245:bool)
                n937 = case shown="False" w2245 {
                  tunnel: w2236 -> [_ w2265]
                  tunnel: w2237 -> [w2250 w2264]
                  tunnel: [w2250 w2263] -> w2244
                  tunnel: [TRUE w2262] -> w2243
                  tunnel: w2242 -> [w2253 w2261]
                  tunnel: [w2251 w2260] -> w2241
                  tunnel: [w2249 w2259] -> w2234
                  tunnel: w2240 -> [w2248 w2257]
                  tunnel: [w2247 w2258] -> w2239
                  frame False {
                    n938 = Increment(x=w2248) -> (x+1=w2247:i32)
                    n939 = Index Array(array=w2253, index=w2247) -> (element=w2252:T57)
                    n940 = Unbundle By Name(w2252) -> ("Name"=w2249:string, "Duration"=w2251:i32)
                  }
                  frame True {
                    n941 = Index Array(array=w2261, index=0) -> (element=w2255:T57)
                    n942 = case shown="True" w2265 {
                      tunnel: w2264 -> [w2272 w2277]
                      tunnel: [w2271 w2277] -> w2263
                      tunnel: [TRUE FALSE] -> w2262
                      tunnel: [w2270 0 ("Duration")] -> w2260
                      tunnel: [w2268 w2276] -> w2259
                      tunnel: [0 w2274] -> w2258
                      tunnel: w2257 -> [_ w2274]
                      tunnel: w2255 -> [w2266 w2273]
                      frame False {
                        n943 = Increment(x=w2272) -> (x+1=w2271:i32)
                        n944 = Unbundle By Name(w2266) -> ("Name"=w2268:string, "Duration"=w2270:i32)
                      }
                      frame True {
                        n945 = Unbundle By Name(w2273) -> ("Name"=w2276:string)
                      }
                    }
                  }
                }
                n946 = property on="Step" class="Str"("Value"=w2234) -> ()  [unwired: 2 in, 2 out]
                n947 = To Double Precision Float(number=w2241) -> ()  [unwired: 1 out]
                n948 = call "Timing FGV.vi"("Timer Mode"=T48."Start Timer") -> ()  [unwired: 8 in, 3 out]
              }
            }
            "Cycle" <- w2190
            n949 = case shown="False" w2199 {
              tunnel: w2198 -> [w2280 w2291]
              tunnel: [w2284 w2291] -> w2191
              frame False {
                n950 = disable-structure shown="Enabled" {
                  disable-tunnel: w2280 -> [w2289 w2290]
                  disable-tunnel: [w2288 w2290] -> w2279
                  frame Enabled {
                    n951 = call <vilib>:"Clear Errors.vi"("error in (no error)"=w2289) -> ("error out"=w2288:errorcluster)  [unwired: 5 in, 1 out]
                  }
                  frame Disabled {
                  }
                }
                n952 = Concatenate Strings("APP:TTV Test>>" ("Command"), "Stop Test" ("Command")) -> (w2281:string)
                n953 = disable-structure shown="Disabled" {
                  disable-tunnel: [w2287 _] -> w2284
                  disable-tunnel: w2281 -> [w2286 _]
                  disable-tunnel: w2279 -> [w2285 _]
                  frame Disabled {
                    n954 = call "Messaging EnQ Single.vi"("Command"=w2286, "error in (no error)"=w2285) -> ("error out"=w2287:errorcluster)  [unwired: 9 in]
                  }
                  frame Enabled {
                  }
                }
              }
              frame True {
              }
            }
            n955 = Bundle By Name(cluster=w2193, "TTV Test.Step"=w2202, "TTV Test.Current Cycle"=w2190) -> (w2192:T27)
          }
          frame "Custom Command" {
            n956 = Concatenate Strings("Command", "\n" ("Command")) -> (w2300:string)
            n957 = call "Serial FGV.vi"("Status"=enum16{"Config", "Read", "Write", "Close"}."Write", "Error In"=w2295, "Command"=w2300) -> ("Error Out"=w2297:errorcluster)  [unwired: 5 in, 3 out]
            n958 = call "Serial FGV.vi"("delay before read (ms)"=u32 10, "Status"=enum16{"Config", "Read", "Write", "Close"}."Read", "Error In"=w2297) -> ("Error Out"=w2294:errorcluster, "Response"=→"Response":string)  [unwired: 5 in, 2 out]
          }
        }
      }
      frame "APP:Load TDMS" {
        n959 = Unbundle By Name(w2306) -> ("IP Address"=w2304:string)
        n960 = call "Dialog TDMS Datalog.vi"("Error In"=w2303, "IP Adrress"=w2304) -> ("Error Out"=w2305:errorcluster)  [unwired: 9 in]
      }
    }
    n961 = call "Add Event.vi"("Log?"=w18, "Name"=w19, "Value"=w15, "Error In"=w21, "Description"=w16, "Boolean"=w17) -> ("Error Out"=w20:errorcluster)  [unwired: 5 in]
  }
  n962 = while {
    tunnel: w10 -> [w2312]
    tunnel: [w2311] -> w13
    stop <- w2313 stop-if-true
    # "Controller"
    n963 = local read "Login TO"() -> (w2307:i32)
    n964 = Multiply(x=60000, y=w2307) -> (x*y=w2308:i32)
    n965 = event shown="[7] \"Login\", \"Datalog\", \"Login TO\": Value Change" {
      selector: _ -> [_ _ _ _ _ _ _ _ _ _ _ _]
      dyn-events: _ -> [_ _ _ _ _ _ _ _ _ _ _ _]
      timeout: w2308 -> [_ _ _ _ _ _ _ _ _ _ _ _]
      tunnel: [w2316 _ _ _ _ _ _ _ _ _ _ w2821] -> w2313
      tunnel: [w2315 w2324 w2339 w2445 w2516 w2666 w2687 w2705 w2757 w2790 w2805 w2824] -> w2311
      tunnel: w2312 -> [w2319 w2328 w2330 w2446 w2515 w2667 w2688 w2706 w2754 w2789 w2806 w2825]
      tunnel: "Net Cluster" -> [_ _ _ _ w2512 w2668 _ _ _ _ _ _]
      event Timeout {
        # "Logout when not received any event for 10 min"
        n966 = event-data() -> ()  [unwired: 1 in, 1 out]
        n967 = property on="Login" class="Bool (strict)"(error in=w2319, "Val(Sgnl)"=T19 FALSE ("Value (Signaling)")) -> (error out=w2317:errorcluster)  [unwired: 1 in, 1 out]
        n968 = call "Messaging AE.vi"("Error In"=w2317) -> ("Error Out"=w2315:errorcluster, "queue out"=w2318:refnum<queue>)  [unwired: 9 in]
        n969 = Not A Number/Path/Refnum?(number/path/refnum=w2318) -> (NaN/Path/Refnum?=w2316:bool)
      }
      event "M1 Set Temp", "M1 Package", "M1 Feedback", "M1 Power Drive Control", "M2 Set Temp", "M2 Package", "M2 Feedback", "M2 Power Drive Control": Value Change {
        n970 = event-data() -> ("CtlRef"=w2329:refnum<vi>, "NewVal"=w2320:variant)  [unwired: 1 in]
        n971 = property class="Ctl"(reference=w2329) -> ("Caption.Text"=w2322:string)  [unwired: 1 in, 2 out]
        n972 = Concatenate Strings("NS:Write>>" ("Command"), w2322) -> (w2327:string)
        n973 = call "Messaging EnQ Single.vi"("Command"=w2327, "Data"=w2320, "error in (no error)"=w2328) -> ("error out"=w2325:errorcluster)  [unwired: 8 in]
        n974 = Concatenate Strings("TCP:Write>>" ("Command"), w2322) -> (w2321:string)
        n975 = call "Messaging EnQ Single.vi"("Command"=w2321, "Data"=w2320, "error in (no error)"=w2325) -> ("error out"=w2324:errorcluster)  [unwired: 8 in]
      }
      event "Power On-Off", "Shutdown", "Reboot RT", "M1 Commands Panel.M1 Enable", "M2 Commands Panel.M2 Enable": Value Change {
        n976 = event-data() -> ("CtlRef"=w2344:refnum<vi>, "NewVal"=w2342:bool)  [unwired: 1 in]
        n977 = property class="Bool"(reference=w2344) -> ("Caption.Text"=w2333:string)  [unwired: 1 in, 2 out]
        n978 = Concatenate Strings("TCP:Write>>" ("Command"), w2333) -> (w2332:string)
        n979 = property on="Comp" class="Bool (strict)"() -> ("Value"=w2343:bool)  [unwired: 2 in, 2 out]
        n980 = Concatenate Strings("NS:Write>>" ("Command"), w2333) -> (w2331:string)
        n981 = case shown="\"M1 Enable\", \"M2 Enable\"" w2333 {
          tunnel: w2343 -> [_ _ w2384 w2414 w2430]
          tunnel: [w2345 w2353 w2386 w2411 w2427] -> w2338
          tunnel: [_ w2354 w2387 w2421 w2437] -> w2337
          tunnel: w2342 -> [_ _ w2385 _ _]
          tunnel: "Are you sure you want to " ("message") -> [_ w2352 _ w2416 w2432]
          tunnel: [w2345 w2348 w2383 w2412 w2428] -> w2336
          tunnel: w2332 -> [_ w2346 w2382 w2410 w2426]
          tunnel: w2331 -> [_ w2347 w2381 w2409 w2425]
          frame Default {
            w2345 = ""
          }
          frame "Power On-Off" {
            n982 = local read "Play/Pause"() -> (w2355:bool)
            n983 = Format Into String(format string="%s", initial string=w2352, "pause?" ("message")) -> (resulting string=w2349:string)  [unwired: 1 in, 1 out]
            n984 = case shown="False" w2355 {
              tunnel: w2349 -> [_ w2377]
              tunnel: [w2358 w2372] -> w2357
              tunnel: [w2363 w2374] -> w2353
              tunnel: w2347 -> [w2365 w2375]
              tunnel: w2346 -> [w2366 w2376]
              tunnel: [w2364 w2373] -> w2348
              frame False {
                n985 = property on="M2 Enable" class="Bool (strict)"() -> ("Value"=w2360:bool)  [unwired: 2 in, 2 out]
                n986 = property on="M1 Enable" class="Bool (strict)"() -> ("Value"=w2361:bool)  [unwired: 2 in, 2 out]
                n987 = Not(x=w2360) -> (.not. x?=w2359:bool)
                n988 = Not(x=w2361) -> (.not. x?=w2362:bool)
                n989 = And(x=w2362, y=w2359) -> (x .and. y?=w2358:bool)
                n990 = case shown="True" w2358 {
                  tunnel: [w2369 w2371] -> w2364
                  tunnel: [w2368 w2371] -> w2363
                  tunnel: "At least one head must be \nenabled to run on" ("message") -> [_ w2370]
                  tunnel: w2366 -> [w2369 _]
                  tunnel: w2365 -> [w2368 _]
                  frame False {
                  }
                  frame True {
                    w2371 = ""
                    n991 = One Button Dialog(message=w2370) -> ()  [unwired: 1 in, 1 out]
                  }
                }
              }
              frame True {
                n992 = Two Button Dialog(message=w2377) -> (T button?=w2372:bool)  [unwired: 2 in]
                n993 = case shown="False" w2372 {
                  tunnel: w2376 -> [_ w2379]
                  tunnel: w2375 -> [_ w2380]
                  tunnel: [w2378 w2380] -> w2374
                  tunnel: [w2378 w2379] -> w2373
                  frame False {
                    w2378 = ""
                  }
                  frame True {
                  }
                }
              }
            }
            n994 = Not(x=w2357) -> (.not. x?=w2356:bool)
            n995 = To Variant(anything=w2356) -> (Variant=w2354:variant)
          }
          frame "M1 Enable", "M2 Enable" {
            n996 = case shown="True" w2384 {
              tunnel: [w2389 w2398] -> w2386
              tunnel: [w2390 w2397] -> w2387
              tunnel: w2385 -> [w2391 w2392]
              tunnel: w2381 -> [w2389 w2395]
              tunnel: w2382 -> [w2388 w2394]
              tunnel: [w2388 w2393] -> w2383
              frame False {
                n997 = To Variant(anything=w2391) -> (Variant=w2390:variant)
              }
              frame True {
                n998 = property on="M2 Enable" class="Bool (strict)"() -> ("Value"=w2402:bool)  [unwired: 2 in, 2 out]
                n999 = property on="M1 Enable" class="Bool (strict)"() -> ("Value"=w2396:bool)  [unwired: 2 in, 2 out]
                n1000 = Not(x=w2402) -> (.not. x?=w2401:bool)
                n1001 = Not(x=w2396) -> (.not. x?=w2400:bool)
                n1002 = And(x=w2400, y=w2401) -> (x .and. y?=w2399:bool)
                n1003 = case shown="False" w2399 {
                  tunnel: w2392 -> [w2404 _]
                  tunnel: [w2405 w2407] -> w2398
                  tunnel: [w2406 _] -> w2397
                  tunnel: w2395 -> [w2405 _]
                  tunnel: w2394 -> [w2403 _]
                  tunnel: [w2403 w2407] -> w2393
                  frame False {
                    n1004 = To Variant(anything=w2404) -> (Variant=w2406:variant)
                  }
                  frame True {
                    w2407 = ""
                    n1005 = One Button Dialog(message="At least one head must be \nenabled to run on") -> ()  [unwired: 1 in, 1 out]
                  }
                }
              }
            }
          }
          frame "Stop RT" {
            n1006 = Format Into String(format string="%s", initial string=w2416, "stop?" ("message")) -> (resulting string=w2420:string)  [unwired: 1 in, 1 out]
            n1007 = Two Button Dialog(message=w2420) -> (T button?=w2415:bool)  [unwired: 2 in]
            n1008 = Not(x=w2414) -> (.not. x?=w2417:bool)
            n1009 = And(x=w2417, y=w2415) -> (x .and. y?=w2413:bool)
            n1010 = case shown="False" w2413 {
              tunnel: w2410 -> [_ w2424]
              tunnel: w2409 -> [_ w2423]
              tunnel: [w2422 w2424] -> w2412
              tunnel: [w2422 w2423] -> w2411
              frame False {
                w2422 = ""
              }
              frame True {
              }
            }
            n1011 = To Variant(anything=w2413) -> (Variant=w2421:variant)
          }
          frame "Reboot RT" {
            n1012 = Format Into String(format string="%s", initial string=w2432, " Reboot RT?" ("message")) -> (resulting string=w2436:string)  [unwired: 1 in, 1 out]
            n1013 = Two Button Dialog(message=w2436) -> (T button?=w2431:bool)  [unwired: 2 in]
            n1014 = Not(x=w2430) -> (.not. x?=w2433:bool)
            n1015 = And(x=w2433, y=w2431) -> (x .and. y?=w2429:bool)
            n1016 = case shown="True" w2429 {
              tunnel: w2426 -> [_ w2440]
              tunnel: w2425 -> [_ w2439]
              tunnel: [w2438 w2440] -> w2428
              tunnel: [w2438 w2439] -> w2427
              frame False {
                w2438 = ""
              }
              frame True {
              }
            }
            n1017 = To Variant(anything=w2429) -> (Variant=w2437:variant)
          }
        }
        n1018 = call "Messaging EnQ Single.vi"("Command"=w2338, "Data"=w2337, "error in (no error)"=w2330) -> ("error out"=w2340:errorcluster)  [unwired: 8 in]
        n1019 = call "Messaging EnQ Single.vi"("Command"=w2336, "Data"=w2337, "error in (no error)"=w2340) -> ("error out"=w2339:errorcluster)  [unwired: 8 in]
      }
      event "M1 Commands Panel.M1 TSD Feedback", "Cascade Compressor controls", "M2 Commands Panel.M2 TSD Feedback", "Manual Bypass Mode", "M1 Heater output", "M1 EEV Manual", "M2 Heater Output", "M2 EEV Manual": Value Change {
        n1020 = event-data() -> ("CtlRef"=w2447:refnum<vi>, "NewVal"=w2444:variant)  [unwired: 1 in]
        n1021 = property class="Ctl"(reference=w2447) -> ("Caption.Text"=w2441:string)  [unwired: 1 in, 2 out]
        n1022 = case shown="Default" w2441 {
          selector: w2441 -> [w2449 _ _ _ _]
          tunnel: w2446 -> [w2453 w2456 w2470 w2484 w2498]
          tunnel: [w2452 w2455 w2469 w2483 w2497] -> w2445
          tunnel: w2444 -> [w2451 w2454 w2468 w2482 w2496]
          tunnel: "Manual Bypass Mode" -> [_ w2462 w2476 w2490 w2504]
          tunnel: "NSV:Write>>" ("DNL_Message") -> [w2450 w2459 w2473 w2487 w2501]
          frame Default {
            n1023 = Concatenate Strings(w2450, w2449) -> (w2448:string)
            n1024 = call "Messaging EnQ Single.vi"("Command"=w2448, "Data"=w2451, "error in (no error)"=w2453) -> ("error out"=w2452:errorcluster)  [unwired: 8 in]
          }
          frame "M2 EEV Manual control" {
            n1025 = Index Array(array=w2462, index=3) -> (element=w2460:bool)
            n1026 = Concatenate Strings(w2459, "M2 EEV Manual" ("format string")) -> (w2458:string)
            n1027 = case shown="True" w2460 {
              tunnel: w2458 -> [_ w2467]
              tunnel: w2456 -> [w2463 w2466]
              tunnel: [w2463 w2465] -> w2455
              tunnel: w2454 -> [_ w2464]
              frame False {
              }
              frame True {
                n1028 = call "Messaging EnQ Single.vi"("Command"=w2467, "Data"=w2464, "error in (no error)"=w2466) -> ("error out"=w2465:errorcluster)  [unwired: 8 in]
              }
            }
          }
          frame "M1 EEV Manual control" {
            n1029 = Index Array(array=w2476, index=1) -> (element=w2474:bool)
            n1030 = Concatenate Strings(w2473, "M1 EEV Manual" ("format string")) -> (w2472:string)
            n1031 = case shown="True" w2474 {
              tunnel: w2472 -> [_ w2481]
              tunnel: w2470 -> [w2477 w2480]
              tunnel: [w2477 w2479] -> w2469
              tunnel: w2468 -> [_ w2478]
              frame False {
              }
              frame True {
                n1032 = call "Messaging EnQ Single.vi"("Command"=w2481, "Data"=w2478, "error in (no error)"=w2480) -> ("error out"=w2479:errorcluster)  [unwired: 8 in]
              }
            }
          }
          frame "M1 Heater PWM" {
            n1033 = Index Array(array=w2490, index=0) -> (element=w2488:bool)
            n1034 = Concatenate Strings(w2487, "M1 Heater output" ("format string")) -> (w2486:string)
            n1035 = case shown="False" w2488 {
              tunnel: w2486 -> [_ w2495]
              tunnel: w2484 -> [w2491 w2494]
              tunnel: [w2491 w2493] -> w2483
              tunnel: w2482 -> [_ w2492]
              frame False {
              }
              frame True {
                n1036 = call "Messaging EnQ Single.vi"("Command"=w2495, "Data"=w2492, "error in (no error)"=w2494) -> ("error out"=w2493:errorcluster)  [unwired: 8 in]
              }
            }
          }
          frame "M2 Heater PWM" {
            n1037 = Index Array(array=w2504, index=2) -> (element=w2502:bool)
            n1038 = Concatenate Strings(w2501, "M2 Heater Output" ("format string")) -> (w2500:string)
            n1039 = case shown="False" w2502 {
              tunnel: w2500 -> [_ w2509]
              tunnel: w2498 -> [w2505 w2508]
              tunnel: [w2505 w2507] -> w2497
              tunnel: w2496 -> [_ w2506]
              frame False {
              }
              frame True {
                n1040 = call "Messaging EnQ Single.vi"("Command"=w2509, "Data"=w2506, "error in (no error)"=w2508) -> ("error out"=w2507:errorcluster)  [unwired: 8 in]
              }
            }
          }
        }
      }
      event "Net Cluster.Menu Ring", "Net Cluster.IP Override": Value Change {
        n1041 = event-data() -> ("NewVal"=w2513:variant, "CtlRef"=w2517:refnum<vi>)  [unwired: 1 in]
        n1042 = Unbundle By Name(w2512) -> ("Menu Ring"=w2511:u16, "Manual IP"=w2510:string)
        n1043 = property class="Ctl"(reference=w2517) -> ("Label.Text"=w2514:string)  [unwired: 1 in, 2 out]
        n1044 = case shown="\"IP Override\"" w2514 {
          tunnel: w2513 -> [_ w2657]
          tunnel: [w2524 w2659] -> w2516
          tunnel: w2515 -> [w2523 w2658]
          tunnel: w2511 -> [w2519 _]
          tunnel: w2510 -> [w2518 _]
          frame "IP Override" {
            n1045 = property on="Menu Ring" class="Ring (strict)"() -> ("Strings []"=w2522:string[])  [unwired: 2 in, 2 out]
            n1046 = for {
              tunnel: "\\b[0-9]+\\.[0-9]+\\.[0-9]+\\.[0-9]+" ("regular expression") -> [w2528]
              tunnel: w2522 -> [w2527] mode=indexing
              tunnel: [w2526] -> w2520 mode=indexing
              n1047 = xnode ("Match Regular Expression")("input string"=w2527, "regular expression"=w2528) -> ("whole match"=w2526:string)  [unwired: 4 in, 4 out]
            }
            n1048 = Empty String/Path?(string/path=w2518) -> (empty?=w2525:bool)
            n1049 = case shown="False" w2525 {
              tunnel: w2519 -> [w2652 _]
              tunnel: w2518 -> [w2654 _]
              tunnel: [w2647 w2655] -> w2524
              tunnel: w2523 -> [w2646 w2655]
              tunnel: w2520 -> [w2643 _]
              frame False {
                n1050 = Search 1D Array(1D array=w2643, element=w2654) -> (index of element=w2650:i32)  [unwired: 1 in]
                n1051 = To Unsigned Word Integer(number=w2650) -> (unsigned 16bit integer=w2649:u16)
                n1052 = Equal?(x=w2650, y=-1) -> (x = y?=w2653:bool)
                n1053 = Select(t=w2652, s=w2653, f=w2649) -> (s? t:f=w2644:u16)
                n1054 = To Variant(anything=w2644) -> (Variant=w2645:variant)
                n1055 = property on="Menu Ring" class="Ring (strict)"("Value"=w2644) -> ()  [unwired: 2 in, 2 out]
                n1056 = call "Messaging EnQ Single.vi"("Command"="MACRO:NS Update", "Data"=w2645, "error in (no error)"=w2646) -> ("error out"=w2647:errorcluster)  [unwired: 8 in]
              }
              frame True {
              }
            }
          }
          frame "Menu Ring", Default {
            n1057 = call "Is Value Changed.vim"("value"=w2657) -> ("changed or first call?"=w2656:bool)
            n1058 = case shown="False" w2656 {
              tunnel: [w2660 w2663] -> w2659
              tunnel: w2658 -> [w2660 w2662]
              tunnel: w2657 -> [_ w2661]
              frame False {
              }
              frame True {
                n1059 = call "Messaging EnQ Single.vi"("Command"="MACRO:NS Update", "Data"=w2661, "error in (no error)"=w2662) -> ("error out"=w2663:errorcluster)  [unwired: 8 in]
              }
            }
          }
        }
      }
      event "Net Cluster.System Ready": Value Change {
        n1060 = event-data() -> ()  [unwired: 1 in, 1 out]
        n1061 = Unbundle By Name(w2668) -> ("System Ready"=w2665:bool)
        n1062 = case shown="True" w2665 {
          tunnel: w2667 -> [w2669 w2673]
          tunnel: [w2669 w2672] -> w2666
          frame False {
          }
          frame True {
            n1063 = Two Button Dialog(message="Are you sure you want to disconnect?") -> (T button?=w2670:bool)  [unwired: 2 in]
            n1064 = case shown="False" w2670 {
              tunnel: w2673 -> [w2674 w2680]
              tunnel: [w2674 w2676] -> w2672
              frame False {
              }
              frame True {
                n1065 = call "Messaging EnQ Single.vi"("Command"="NS:Close Connection", "error in (no error)"=w2680) -> ("error out"=w2677:errorcluster)  [unwired: 9 in]
                n1066 = call "Messaging EnQ Single.vi"("Command"="NS:Update IP", "Data"=variant, "error in (no error)"=w2677) -> ("error out"=w2676:errorcluster)  [unwired: 8 in]
              }
            }
          }
        }
      }
      event "Configure", "Package", "Graph Temp Unit", "Net Cluster.Refresh": Value Change {
        n1067 = event-data() -> ("CtlRef"=w2686:refnum<vi>, "NewVal"=w2682:bool)  [unwired: 1 in]
        n1068 = property class="Bool"(reference=w2686) -> ("Label.Text"=w2685:string)  [unwired: 1 in, 2 out]
        n1069 = case shown="\"Refresh\", Default" w2685 {
          selector: w2685 -> [_ _ w2698 w2701]
          tunnel: ["NS:Detect Systems" ("Command(s)") "UI:Refresh Graph" ("Command") w2697 w2700] -> w2684
          tunnel: [TRUE ("@Front?") _ _ _] -> w2683
          tunnel: w2682 -> [_ w2695 _ _]
          tunnel: [_ w2691 _ _] -> w2681
          frame "Refresh", Default {
          }
          frame "Graph Temp Unit" {
            n1070 = Select(t="°C" ("Command"), s=w2695, f="°F" ("Command")) -> (s? t:f=w2692:string)
            n1071 = To Variant(anything=w2692) -> (Variant=w2691:variant)
          }
          frame "Configure" {
            n1072 = Concatenate Strings("APP:Update Config>>" ("Command(s)"), w2698) -> (w2697:string)
          }
          frame "Package" {
            n1073 = Concatenate Strings("APP:Update Config>>" ("Command(s)"), w2701) -> (w2700:string)
          }
        }
        n1074 = call "Messaging EnQ Single.vi"("Command"=w2684, "@Front?"=w2683, "Data"=w2681, "error in (no error)"=w2688) -> ("error out"=w2687:errorcluster)  [unwired: 7 in]
      }
      event "Datalog", "Login TO": Value Change {
        n1075 = event-data() -> ("OldVal"=w2703:variant, "CtlRef"=w2708:refnum<vi>, "NewVal"=w2704:variant)  [unwired: 1 in]
        n1076 = property class="Ctl"(reference=w2708) -> ("Label.Text"=w2707:string)  [unwired: 1 in, 2 out]
        n1077 = case shown="\"Login TO\"" w2707 {
          tunnel: w2706 -> [w2709 w2714 w2722 w2724]
          tunnel: [w2709 w2710 w2720 w2730] -> w2705
          tunnel: w2704 -> [_ w2713 _ w2727]
          tunnel: w2703 -> [_ w2712 _ _]
          frame Default {
          }
          frame "Login TO" {
            n1078 = Variant To Data(type=0 ("Login TO"), Variant=w2712) -> (data=w2717:i32)  [unwired: 1 in, 1 out]
            n1079 = Variant To Data(error in=w2714, type=0 ("Login TO"), Variant=w2713) -> (data=w2718:i32, error out=w2710:errorcluster)
            n1080 = Equal To 0?(x=w2718) -> (x = 0?=w2719:bool)
            n1081 = Select(t=w2717, s=w2719, f=w2718) -> (s? t:f=w2711:i32)
            n1082 = property on="Login TO" class="DigNum (strict)"("Value"=w2711) -> ()  [unwired: 2 in, 2 out]
          }
          frame "Datalog" {
            n1083 = call "Messaging EnQ Single.vi"("Command"="APP:Load TDMS", "error in (no error)"=w2722) -> ("error out"=w2720:errorcluster)  [unwired: 9 in]
          }
          frame "Login" {
            n1084 = Variant To Data(error in=w2724, type=FALSE, Variant=w2727) -> (data=w2725:bool, error out=w2723:errorcluster)
            n1085 = case shown="True" w2725 {
              tunnel: w2723 -> [w2733 w2740]
              tunnel: [w2733 w2735] -> w2731
              tunnel: [T46."Operator" ("f") w2736] -> w2732
              frame False {
              }
              frame True {
                n1086 = call "Login.vi"("error in"=w2740) -> ("error out"=w2739:errorcluster, "OK?"=w2737:bool, "Level"=w2738:T46)  [unwired: 7 in]
                n1087 = case shown="False" w2737 {
                  tunnel: w2739 -> [w2742 w2745]
                  tunnel: w2738 -> [_ w2746]
                  tunnel: [T46."Operator" ("f") w2746] -> w2736
                  tunnel: [w2741 w2745] -> w2735
                  frame False {
                    n1088 = property on="Login" class="Bool (strict)"(error in=w2742, "Value"=FALSE ("Login")) -> (error out=w2741:errorcluster)  [unwired: 1 in, 1 out]
                  }
                  frame True {
                  }
                }
              }
            }
            n1089 = To Variant(anything=w2732) -> (Variant=w2729:variant)
            n1090 = call "Messaging EnQ Single.vi"("Command"="DB:Login", "Data"=w2729, "error in (no error)"=w2731) -> ("error out"=w2730:errorcluster)  [unwired: 8 in]
          }
        }
      }
      event "Pattern File", "Seq Controls", "Iteration No": Value Change {
        n1091 = event-data() -> ("CtlRef"=w2756:refnum<vi>, "NewVal"=w2751:variant)  [unwired: 1 in]
        n1092 = property class="Ctl"(reference=w2756) -> ("Label.Text"=w2752:string)  [unwired: 1 in, 2 out]
        n1093 = case shown="\"Seq Controls\"" w2752 {
          selector: w2752 -> [w2759 _ _ _]
          tunnel: [w2761 w2766 w2769 _] -> w2747
          tunnel: [w2760 w2765 w2770 w2774] -> w2753
          tunnel: w2751 -> [w2761 _ _ w2780]
          tunnel: w2754 -> [w2760 w2765 w2770 w2781]
          tunnel: [w2759 "Power Sequence" ("Command") "Power Sequence" ("Command") w2775] -> w2748
          tunnel: "Power Seq" -> [_ w2764 w2773 _]
          tunnel: "Iteration No" -> [_ w2762 w2768 _]
          frame Default {
          }
          frame "Power Seq" {
            n1094 = Bundle("Iteration No"=w2762, "Power Seq"=w2764) -> (w2767:cluster{"Iteration No":i32, "Power Seq":T25})  [unwired: 1 in]
            n1095 = To Variant(anything=w2767) -> (Variant=w2766:variant)
          }
          frame "Iteration No" {
            n1096 = Bundle("Iteration No"=w2768, "Power Seq"=w2773) -> (w2772:cluster{"Iteration No":i32, "Power Seq":T25})  [unwired: 1 in]
            n1097 = To Variant(anything=w2772) -> (Variant=w2769:variant)
          }
          frame "Seq Controls" {
            n1098 = Variant To Data(error in=w2781, type=T26 {"Refresh Seq"=FALSE, "Save Seq"=FALSE, "Delete Seq"=FALSE, "Clear Seq"=FALSE} ("Seq Controls"), Variant=w2780) -> (data=w2778:T26, error out=w2774:errorcluster)
            n1099 = Cluster To Array(cluster=w2778) -> (array=w2777:bool[])
            n1100 = Search 1D Array(1D array=w2777, element=TRUE) -> (index of element=w2776:i32)  [unwired: 1 in]
            n1101 = case shown="2" w2776 {
              tunnel: ["Refresh Seq" ("Command") "Save Seq" ("Command") "Delete Seq" ("Command") "Clear Seq" ("Command")] -> w2775
              frame 0, Default {
              }
              frame 1 {
              }
              frame 2 {
              }
              frame 3 {
              }
            }
          }
        }
        n1102 = Concatenate Strings("APP:Power Sequence(GUI)>>" ("Command"), w2748) -> (w2758:string)
        n1103 = call "Messaging EnQ Single.vi"("Command"=w2758, "Data"=w2747, "error in (no error)"=w2753) -> ("error out"=w2757:errorcluster)  [unwired: 8 in]
      }
      event "Power", "Start Test", "Stop Test", "Reset Test", "Serial Port", "Custom Command": Value Change {
        n1104 = event-data() -> ("CtlRef"=w2788:refnum<vi>, "NewVal"=w2787:variant)  [unwired: 1 in]
        n1105 = property class="Ctl"(reference=w2788) -> ("Label.Text"=w2791:string)  [unwired: 1 in, 2 out]
        n1106 = case shown="Default" w2791 {
          selector: w2791 -> [w2797 _]
          tunnel: "APP:TTV Test>>" ("Command") -> [w2798 _]
          tunnel: w2787 -> [w2795 _]
          tunnel: w2789 -> [w2794 w2802]
          tunnel: [w2793 w2801] -> w2790
          frame Default {
            n1107 = Concatenate Strings(w2798, w2797) -> (w2796:string)
            n1108 = call "Messaging EnQ Single.vi"("Command"=w2796, "Data"=w2795, "error in (no error)"=w2794) -> ("error out"=w2793:errorcluster)  [unwired: 8 in]
          }
          frame "Serial Port" {
            n1109 = constructor class="SerialPort"(error in=w2802) -> (reference out=w2803:refnum<k24>, error out=w2804:errorcluster)  [unwired: 2 in, 1 out]
            n1110 = invoke on="牢焊农 畴靛" class="SerialPort" method="GetPortNames"(reference=w2803, error in=w2804) -> (error out=w2800:errorcluster, "GetPortNames"=w2799:string[])  [unwired: 1 in, 1 out]
            n1111 = property on="Serial Port" class="CmbBox"(error in=w2800, "Strings[]"=w2799) -> (error out=w2801:errorcluster)  [unwired: 1 in, 1 out]
          }
        }
      }
      event "Tab Control": Value Change {
        # "Make sure File path : application error"
        n1112 = event-data() -> ("NewVal"=w2807:T6)  [unwired: 1 in]
        n1113 = disable-structure shown="Enabled" {
          disable-tunnel: w2807 -> [w2812 _]
          disable-tunnel: w2806 -> [w2811 _]
          disable-tunnel: [w2810 _] -> w2805
          frame Disabled {
            n1114 = Equal?(x=w2812, y=T6."TEST" ("NewVal")) -> (x = y?=w2809:bool)
            n1115 = case shown="True" w2809 {
              tunnel: w2811 -> [w2813 w2815]
              tunnel: [w2813 w2814] -> w2810
              frame False {
              }
              frame True {
                n1116 = Concatenate Strings("APP:Power Sequence(GUI)>>" ("Command"), "Initialize" ("Command")) -> (w2818:string)
                n1117 = call "Messaging EnQ Single.vi"("Command"=w2818, "error in (no error)"=w2815) -> ("error out"=w2814:errorcluster)  [unwired: 9 in]
              }
            }
          }
          frame Enabled {
          }
        }
      }
      event Panel Close? {
        n1118 = event-data() -> ()  [unwired: 1 in, 1 out]
        n1119 = Two Button Dialog(message="Are you sure you want to Stop the Application?") -> (T button?=w2822:bool)  [unwired: 2 in]
        n1120 = case shown="True" w2822 {
          tunnel: w2825 -> [w2828 w2832]
          tunnel: [w2828 w2831] -> w2824
          tunnel: [FALSE ("Discard?") TRUE ("Discard?")] -> w2821
          tunnel: "MACRO:Shutdown" ("Command") -> [_ w2830]
          tunnel: [TRUE ("Discard?") FALSE ("Discard?")] -> w2819
          frame False {
          }
          frame True {
            n1121 = call "Messaging EnQ Single.vi"("Command"=w2830, "error in (no error)"=w2832) -> ("error out"=w2831:errorcluster)  [unwired: 9 in]
          }
        }
        n1122 = event-data("Discard?"=w2819) -> ()  [unwired: 1 in, 1 out]
      }
    }
  }
  n1123 = Merge Errors(w13, w12) -> (→"Error Out":errorcluster)
